vi "Text control 2 v6.6_pump-specific.vi"() -> ()   [LabVIEW 2016]
panel:
  in  "Tab Control":enum32{"Main", "Other parameters"}(tab)
  out "Line running":i32
  out "Total lines":i32
  out "Path":path=path "C:/users/rlp38/09Apr2009LTtesting/test2.txt"
  out "I vs Vg":cluster{"Y data in":dbl[], "X data in":dbl[]}[](graph)
  out "Is max":dbl format="%.2e"
  out "Id max":dbl format="%.2e"
  out "Ig max":dbl format="%.2e"
  out "Imax vs time":cluster{"Y data in":dbl[], "X data in":dbl[]}[](graph)
  out "Imin vs time":cluster{"Y data in":dbl[], "X data in":dbl[]}[](graph)
  out "I vs Vd":cluster{"Y data in":dbl[], "X data in":dbl[]}[](graph)
  in  "Script":string="#-------------------------------------------------------\n# SPM pump cleaning script\n#\n# Version: 0.5\n# Author: Dimitrios Simatos\n# Last updated: 2018-01-05\n#-------------------------------------------------------\n# Description\n#\n# This script is designed to run the cleaning sequence of the SPM OEM pump.\n# This script needs to be run 4 times!\n#-------------------------------------------------------\n# Changes\n#\n# Placed initialization and hard stop commands in the beginning.\n#-------------------------------------------------------\n# Important points\n#\n# Never leave any liquid in the pump to dry after the experiments. If they dry, the residue may block the valve.\n# Always run the cleaning cycle after the experiments.\n# Use clockwise rotation when going up in valve port numbers and vice versa.\n#-------------------------------------------------------\n# Things to do before running the script\n#\n# Set time units to minutes.\n# Set filenames.\n# Replace the tubing, if necessary.\n#-------------------------------------------------------\n# Port connections\n#\n# Port 1: Waste\n# Port 2: Waste\n# Port 3: Various cleaning liquids\n# Port 4: Waste\n# Port 5: Waste\n# Port 6: Waste\n#\n# Between each of the 4 runs, the settings of Port 3 will change, according to the cleaning protocol.\n# The settings for Port 3 are:\n# 1st run: 1% v/v solution of sodium hypochlorite in ultrapure water\n# 2nd run: 0.1% w/v solution of sodium dodecyl sulfate in ultrapure water\n# 3rd run: Ultrapure water\n# 4th run: Waste (in air, not immersed in liquid)\n#-------------------------------------------------------\n# Cleaning protocol for the SPM OEM pump (from the manual)\n#\n# A cleaning procedure should be performed at the end of each day or in between two different experiments.\n# An effective cleaning can be performed in the following manner:\n# • Bleach solution to kill microorganisms\n# 1. Prepare a solution of 1% chlorine bleach and deionized water\n#    NOTE: Prepare a 1% v/v solution of sodium hypochlorite in deionized water\n# 2. Prepare a reservoir and place 1 tubing in the bleach solution and 5 tubings in a waste recipient\n# 3. Pick up the bleach solution through 1 port to entirely fill the syringe\n# 4. Sequentially output the syringe content through the remaining ports and throw it to the waste\n# 5. Repeat operation at least 2 times\n# • Detergent solution to remove debris\n# 1. Prepare a solution of 0.1% detergent and deionized water\n#    NOTE: Prepare a 0.1% w/v solution of sodium dodecyl sulfate in deionized water\n# 2. Move the tubing from the bleach solution reservoir and place it into a reservoir of detergent solution\n# 3. Pick up the detergent solution through 1 port to entirely fill the syringe\n# 4. Sequentially output the detergent solution through the remaining ports into the waste recipient\n# 5. Repeat operation at least 2 times\n# • Rinsing water to prepare the pump for your next experiment\n# 1. Move the tubing from the detergent solution reservoir and place it into a reservoir of deionized water\n# 2. Pick up the rinsing solution through 1 port to entirely fill the syringe\n# 3. Sequentially output the rinse water through the remaining ports into the waste recipient\n# 4. Repeat operation at least 2 times\n# • Replace the tubing, if necessary\n#-------------------------------------------------------\n# Pumping cycles and execution time\n#\n# Execution time for a single cycle: 6 x (1 min + 10 sec) = 7 minutes\n# Total execution time: 4 x 7 = 28 minutes\n# Since the script has to run 4 times, the cleaning lasts for: 4 x 28 = 112 minutes\n# Air must be the last to be pumped through the valve, to remove all liquids.\n# There are 4 pumping cycles. Each one draws a different liquid through port 3 and pumps it sequentially through ports 1,2,4,5,6.\n# During the sequential pumping, each port receives 200 ml of liquid (20% of the total syringe volume = 600 \"plunger units\")\n# The device must be disconnected from the port during the cleaning procedure.\n# All cycles are similar, except cycle 1 has the initialization command uncommented and the first report valve command commented.\n#-------------------------------------------------------\n# Volume of liquid needed\n#\n# Volume of liquid needed per cycle: 1 ml\n# Total volume of liquid needed per script run: 4 x 1 = 4 ml\n# Since the script has to run 4 times, the first 3 with different liquids, I need:\n# 4 ml of 1% v/v solution of sodium hypochlorite in ultrapure water\n# 4 ml of 0.1% w/v solution of sodium dodecyl sulfate in ultrapure water\n# 4 ml of ultrapure water\n#-------------------------------------------------------\n# Parameters\n#\n# Syringe size: 1 ml\n# Step resolution N = 0.01 mm\n# Drawing flow V = 300 pulses/second (6000 ul/min)\n# Pumping flow V = 300 pulses/second (6000 ul/min)\n#-------------------------------------------------------\n# Pump initialization\npump /1T #hard stop pump\npump /1ZR #initialize pump\n#-------------------------------------------------------\n# Cycle 1\n# Fill the syringe\npump /1Q #query pump\npump /1? #report absolute plunger position\n#pump /1?6 #report valve position\nwait-min 1 #wait 1 minute\npump /1N0R #set step resolution: 0.01 mm\npump /1Q #query pump\npump /1? #report absolute plunger position (the plunger should be at 0)\npump /1?6 #report valve position\nwait 1000 #wait 1 second\npump /1V300R #choose speed: 300 steps/s (6000 ul/min)\npump /1Q #query pump\nwait 1000 #wait 1 second\npump /1I3R #go to port 3, clockwise rotation\npump /1Q #query pump\npump /1?6 #report valve position\nwait 1000 #wait 1 second\npump /1A3000R #go to absolute position 3000 (= draw 1 ml)\nwait 30000 #wait 30 seconds\npump /1Q #query pump\npump /1? #report absolute plunger position (the plunger should have finished moving)\n#pump /1?6 #report valve position\n# The sequential pumping begins\n# Port 1\npump /1O1R #switch to port 1, counterclockwise rotation\npump /1Q #query pump\npump /1?6 #report valve position\npump /1A2400R #go to absolute position 2400 (= pump 200 ul)\npump /1Q #query pump\npump /1? #report absolute plunger position (the plunger should be moving to 0)\nwait-min 1 #wait 1 minute\npump /1? #report absolute plunger position (the plunger should have finished moving)\n# Port 2\npump /1I2R #switch to port 2, clockwise rotation\npump /1Q #query pump\npump /1?6 #report valve position\npump /1A1800R #go to absolute position 1800 (= pump 200 ul)\npump /1Q #query pump\npump /1? #report absolute plunger position (the plunger should be moving to 0)\nwait-min 1 #wait 1 minute\npump /1? #report absolute plunger position (the plunger should have finished moving)\n# Port 4\npump /1I4R #switch to port 4, clockwise rotation\npump /1Q #query pump\npump /1?6 #report valve position\npump /1A1200R #go to absolute position 1200 (= pump 200 ul)\npump /1Q #query pump\npump /1? #report absolute plunger position (the plunger should be moving to 0)\nwait-min 1 #wait 1 minute\npump /1? #report absolute plunger position (the plunger should have finished moving)\n# Port 5\npump /1I5R #switch to port 5, clockwise rotation\npump /1Q #query pump\npump /1?6 #report valve position\npump /1A600R #go to absolute position 600 (= pump 200 ul)\npump /1Q #query pump\npump /1? #report absolute plunger position (the plunger should be moving to 0)\nwait-min 1 #wait 1 minute\npump /1? #report absolute plunger position (the plunger should have finished moving)\n# Port 6\npump /1I6R #switch to port 6, clockwise rotation\npump /1Q #query pump\npump /1?6 #report valve position\npump /1A0R #go to absolute position 0 (= pump 200 ul)\npump /1Q #query pump\npump /1? #report absolute plunger position (the plunger should be moving to 0)\nwait-min 1 #wait 1 minute\npump /1? #report absolute plunger position (the plunger should have finished moving)\n#-------------------------------------------------------\n# Cycle 2\n# Fill the syringe\n#pump /1ZR #initialize pump\npump /1Q #query pump\npump /1? #report absolute plunger position\npump /1?6 #report valve position\nwait-min 1 #wait 1 minute\npump /1N0R #set step resolution: 0.01 mm\npump /1Q #query pump\npump /1? #report absolute plunger position (the plunger should be at 0)\npump /1?6 #report valve position\nwait 1000 #wait 1 second\npump /1V300R #choose speed: 300 steps/s (6000 ul/min)\npump /1Q #query pump\nwait 1000 #wait 1 second\npump /1O3R #go to port 3, counterclockwise rotation\npump /1Q #query pump\npump /1?6 #report valve position\nwait 1000 #wait 1 second\npump /1A3000R #go to absolute position 3000 (= draw 1 ml)\nwait 30000 #wait 30 seconds\npump /1Q #query pump\npump /1? #report absolute plunger position (the plunger should have finished moving)\n#pump /1?6 #report valve position\n# The sequential pumping begins\n# Port 1\npump /1O1R #switch to port 1, counterclockwise rotation\npump /1Q #query pump\npump /1?6 #report valve position\npump /1A2400R #go to absolute position 2400 (= pump 200 ul)\npump /1Q #query pump\npump /1? #report absolute plunger position (the plunger should be moving to 0)\nwait-min 1 #wait 1 minute\npump /1? #report absolute plunger position (the plunger should have finished moving)\n# Port 2\npump /1I2R #switch to port 2, clockwise rotation\npump /1Q #query pump\npump /1?6 #report valve position\npump /1A1800R #go to absolute position 1800 (= pump 200 ul)\npump /1Q #query pump\npump /1? #report absolute plunger position (the plunger should be moving to 0)\nwait-min 1 #wait 1 minute\npump /1? #report absolute plunger position (the plunger should have finished moving)\n# Port 4\npump /1I4R #switch to port 4, clockwise rotation\npump /1Q #query pump\npump /1?6 #report valve position\npump /1A1200R #go to absolute position 1200 (= pump 200 ul)\npump /1Q #query pump\npump /1? #report absolute plunger position (the plunger should be moving to 0)\nwait-min 1 #wait 1 minute\npump /1? #report absolute plunger position (the plunger should have finished moving)\n# Port 5\npump /1I5R #switch to port 5, clockwise rotation\npump /1Q #query pump\npump /1?6 #report valve position\npump /1A600R #go to absolute position 600 (= pump 200 ul)\npump /1Q #query pump\npump /1? #report absolute plunger position (the plunger should be moving to 0)\nwait-min 1 #wait 1 minute\npump /1? #report absolute plunger position (the plunger should have finished moving)\n# Port 6\npump /1I6R #switch to port 6, clockwise rotation\npump /1Q #query pump\npump /1?6 #report valve position\npump /1A0R #go to absolute position 0 (= pump 200 ul)\npump /1Q #query pump\npump /1? #report absolute plunger position (the plunger should be moving to 0)\nwait-min 1 #wait 1 minute\npump /1? #report absolute plunger position (the plunger should have finished moving)\n#-------------------------------------------------------\n# Cycle 3\n# Fill the syringe\n#pump /1ZR #initialize pump\npump /1Q #query pump\npump /1? #report absolute plunger position\npump /1?6 #report valve position\nwait-min 1 #wait 1 minute\npump /1N0R #set step resolution: 0.01 mm\npump /1Q #query pump\npump /1? #report absolute plunger position (the plunger should be at 0)\npump /1?6 #report valve position\nwait 1000 #wait 1 second\npump /1V300R #choose speed: 300 steps/s (6000 ul/min)\npump /1Q #query pump\nwait 1000 #wait 1 second\npump /1O3R #go to port 3, counterclockwise rotation\npump /1Q #query pump\npump /1?6 #report valve position\nwait 1000 #wait 1 second\npump /1A3000R #go to absolute position 3000 (= draw 1 ml)\nwait 30000 #wait 30 seconds\npump /1Q #query pump\npump /1? #report absolute plunger position (the plunger should have finished moving)\n#pump /1?6 #report valve position\n# The sequential pumping begins\n# Port 1\npump /1O1R #switch to port 1, counterclockwise rotation\npump /1Q #query pump\npump /1?6 #report valve position\npump /1A2400R #go to absolute position 2400 (= pump 200 ul)\npump /1Q #query pump\npump /1? #report absolute plunger position (the plunger should be moving to 0)\nwait-min 1 #wait 1 minute\npump /1? #report absolute plunger position (the plunger should have finished moving)\n# Port 2\npump /1I2R #switch to port 2, clockwise rotation\npump /1Q #query pump\npump /1?6 #report valve position\npump /1A1800R #go to absolute position 1800 (= pump 200 ul)\npump /1Q #query pump\npump /1? #report absolute plunger position (the plunger should be moving to 0)\nwait-min 1 #wait 1 minute\npump /1? #report absolute plunger position (the plunger should have finished moving)\n# Port 4\npump /1I4R #switch to port 4, clockwise rotation\npump /1Q #query pump\npump /1?6 #report valve position\npump /1A1200R #go to absolute position 1200 (= pump 200 ul)\npump /1Q #query pump\npump /1? #report absolute plunger position (the plunger should be moving to 0)\nwait-min 1 #wait 1 minute\npump /1? #report absolute plunger position (the plunger should have finished moving)\n# Port 5\npump /1I5R #switch to port 5, clockwise rotation\npump /1Q #query pump\npump /1?6 #report valve position\npump /1A600R #go to absolute position 600 (= pump 200 ul)\npump /1Q #query pump\npump /1? #report absolute plunger position (the plunger should be moving to 0)\nwait-min 1 #wait 1 minute\npump /1? #report absolute plunger position (the plunger should have finished moving)\n# Port 6\npump /1I6R #switch to port 6, clockwise rotation\npump /1Q #query pump\npump /1?6 #report valve position\npump /1A0R #go to absolute position 0 (= pump 200 ul)\npump /1Q #query pump\npump /1? #report absolute plunger position (the plunger should be moving to 0)\nwait-min 1 #wait 1 minute\npump /1? #report absolute plunger position (the plunger should have finished moving)\n#-------------------------------------------------------\n# Cycle 4\n# Fill the syringe\n#pump /1ZR #initialize pump\npump /1Q #query pump\npump /1? #report absolute plunger position\npump /1?6 #report valve position\nwait-min 1 #wait 1 minute\npump /1N0R #set step resolution: 0.01 mm\npump /1Q #query pump\npump /1? #report absolute plunger position (the plunger should be at 0)\npump /1?6 #report valve position\nwait 1000 #wait 1 second\npump /1V300R #choose speed: 300 steps/s (6000 ul/min)\npump /1Q #query pump\nwait 1000 #wait 1 second\npump /1O3R #go to port 3, counterclockwise rotation\npump /1Q #query pump\npump /1?6 #report valve position\nwait 1000 #wait 1 second\npump /1A3000R #go to absolute position 3000 (= draw 1 ml)\nwait 30000 #wait 30 seconds\npump /1Q #query pump\npump /1? #report absolute plunger position (the plunger should have finished moving)\n#pump /1?6 #report valve position\n# The sequential pumping begins\n# Port 1\npump /1O1R #switch to port 1, counterclockwise rotation\npump /1Q #query pump\npump /1?6 #report valve position\npump /1A2400R #go to absolute position 2400 (= pump 200 ul)\npump /1Q #query pump\npump /1? #report absolute plunger position (the plunger should be moving to 0)\nwait-min 1 #wait 1 minute\npump /1? #report absolute plunger position (the plunger should have finished moving)\n# Port 2\npump /1I2R #switch to port 2, clockwise rotation\npump /1Q #query pump\npump /1?6 #report valve position\npump /1A1800R #go to absolute position 1800 (= pump 200 ul)\npump /1Q #query pump\npump /1? #report absolute plunger position (the plunger should be moving to 0)\nwait-min 1 #wait 1 minute\npump /1? #report absolute plunger position (the plunger should have finished moving)\n# Port 4\npump /1I4R #switch to port 4, clockwise rotation\npump /1Q #query pump\npump /1?6 #report valve position\npump /1A1200R #go to absolute position 1200 (= pump 200 ul)\npump /1Q #query pump\npump /1? #report absolute plunger position (the plunger should be moving to 0)\nwait-min 1 #wait 1 minute\npump /1? #report absolute plunger position (the plunger should have finished moving)\n# Port 5\npump /1I5R #switch to port 5, clockwise rotation\npump /1Q #query pump\npump /1?6 #report valve position\npump /1A600R #go to absolute position 600 (= pump 200 ul)\npump /1Q #query pump\npump /1? #report absolute plunger position (the plunger should be moving to 0)\nwait-min 1 #wait 1 minute\npump /1? #report absolute plunger position (the plunger should have finished moving)\n# Port 6\npump /1I6R #switch to port 6, clockwise rotation\npump /1Q #query pump\npump /1?6 #report valve position\npump /1A0R #go to absolute position 0 (= pump 200 ul)\npump /1Q #query pump\npump /1? #report absolute plunger position (the plunger should be moving to 0)\nwait-min 1 #wait 1 minute\npump /1? #report absolute plunger position (the plunger should have finished moving)\n#-------------------------------------------------------"
  out "Command running:":string
  out "Serial port data":string
  out "Elapsed Time":dbl caption="Elapsed Time (s)"
  in  "Time Units":u16(ring)=1 items=["Seconds", "Minutes", "Hours"]
  in  "Time Offset":dbl caption="Set Start Time (s)"
  in  "Reset":bool
  in  "Auto Reset":bool
  in  "integration time":u32(slide) max=2 step=1 scale=0.0..2.0
  in  "Interrupt scan":bool
  out "Absolute plunger position vs time":cluster{"Y data in":dbl[], "X data in":dbl[]}[](graph)
  out "Valve position vs time":cluster{"Y data in":dbl[], "X data in":dbl[]}[](graph)
  out "Is on":dbl format="%.2e"
  out "Id on":dbl format="%.2e"
  out "Ig on":dbl format="%.2e"
  out "Ion vs time":cluster{"Y data in":dbl[], "X data in":dbl[]}[](graph)
  out "Ioff vs time":cluster{"Y data in":dbl[], "X data in":dbl[]}[](graph)
  out "Ig min":dbl format="%.2e"
  out "Id min":dbl format="%.2e"
  out "Is min":dbl format="%.2e"
  out "Is off":dbl format="%.2e"
  out "Id off":dbl format="%.2e"
  out "Ig off":dbl format="%.2e"
  in  "Integration time (long)":dbl=0.32 min=0.04 max=2.0 step=0.02 format="%.2f"
  in  "Integration time (short)":dbl=0.0019 min=8e-05 max=0.0019 step=8e-05 format="%^.0e"
  in  "Gate: Compliance":dbl=0.001 format="%.8f"
  in  "Drain: Compliance":dbl=0.001 format="%.8f"
  in  "Hard stop pump":bool
  in  "Halt pump":bool
  in  "Interrupt program":bool
  in  "Suffix (script)":string="step_1_up-H2O_initial_script.txt"
  in  "Filename (variable part)":string="step_1_up-H2O_initial_"
  in  "Plot output curve extrema vs time":bool
  in  "Plot transfer curve extrema vs time":bool=TRUE
  in  "Plot sample extrema vs time":bool
  out "I vs time (Bias Stress)":cluster{"Y data in":dbl[], "X data in":dbl[]}[](graph)
  in  "Gate Range\nmode":u16(ring) items=["Auto", "Limited", "Fixed"]
  in  "Gate Range":u8(slide)=6 max=11 scale=0.0..11.0
  in  "Source/Drain\nRange mode":u16(ring) items=["Auto", "Limited", "Fixed"]
  in  "Source/Drain Range":u8(slide)=6 max=11 scale=0.0..11.0
  in  "Panel Controls":T1={"Emergency Stop"=refnum, "TransGraph Max"=1e-05, "Text/Graph (text=false)"=TRUE} {"TransGraph Max" format="%.2e"}
  in  "Panel Controls 2":T2={"Emergency Stop"=refnum, "TransGraph Max"=1e-05, "Text/Graph (text=false)"=TRUE, "TransGraph Min"=1e-11} {"TransGraph Min" format="%.2e"; "TransGraph Max" format="%.2e"}
  in  "SMU4":cluster{"on/off":bool, "Voltage":dbl} {"Voltage" min=-100.0 max=100.0 format="%.2f"}
  in  "Full Reset":bool
  in  "Standby":T3
  out "error out":errorcluster
  in  "Delay before read (ms)":u32=1000
  in  "byte count":u32=64
  in  "Serial End Mode for Reads":u16(ring)=2 items=["None", "LastBit", "TermChar"]
  in  "Timeout (ms)":u32=10000
  in  "Enable Termination\nChar (T)":bool=TRUE
  in  "Termination char\n(0xA = '\\n' = LF)\n(0xD = '\\r' = CR)":u8=13 format="%.0x"
  in  "flow control":u16(ring) items=["None"=0, "XON/XOFF"=1, "RTS/CTS"=2, "DTR/DSR"=4]
  in  "stop bits":u16(ring)=10 items=["1.0"=10, "1.5"=15, "2.0"=20]
  in  "parity":u16(ring) items=["None", "Odd", "Even", "Mark", "Space"]
  in  "data bits":u16=8 min=5 max=8 step=1
  in  "VISA resource name":refnum<visa-resource-name>="COM6"
  in  "baud rate":u32=9600
  out "Timings Indicator":T4
  in  "Timings (overwritten by the Front Panel)":T5={"integration time"=0, "Short/Long integration time"=0.00064, "hold time (sec)"=0.0, "delay time (sec)"=0.0, "Step Time (0 disables)"=0.0, "sweep method"=0, "Pulse period"=0.005, "Base voltage"=0.0, "Pulse width"=0.0005} {"Pulse width" min=0.0005 max=0.1 step=0.0001 format="%.4f"; "Base voltage" format="%^.4e"; "Pulse period" min=0.005 max=1.0 step=0.0001 format="%.4f"; "sweep method" items=["Continuous", "Pulsed"]; "Step Time (0 disables)" format="%.2f"; "delay time (sec)" format="%.4f"; "hold time (sec)" format="%.4f"; "Short/Long integration time" format="%^.0e"; "integration time" scale=0.0..2.0}
  out "SMU4 Indicator":cluster{"on/off":bool, "Voltage":dbl} {"Voltage" min=-100.0 max=100.0 format="%.2f"}
  in  "Gate":T6={"Gate Start"=0.0, "Gate Stop"=2.0, "Gate Step (linear only)"=1.0, "Gate Compliance"=0.0001, "Gate PComp"=0.0, "Range mode"=0, "Range"=6} {"Range" max=11 scale=0.0..11.0; "Range mode" items=["Auto", "Limited", "Fixed"]; "Gate PComp" format="%^.2e"; "Gate Compliance" format="%^.2e"; "Gate Step (linear only)" format="%^.4e"; "Gate Stop" format="%^.4e"; "Gate Start" format="%^.4e"}
  in  "Drain 2":T7={"Drain Start"=0.0, "Drain Stop"=2.0, "Drain Compliance"=0.0001, "Drain Step"=1.0, "Drain PComp"=0.0, "Range mode"=0, "Range"=6} {"Range" max=11 scale=0.0..11.0; "Range mode" items=["Auto", "Limited", "Fixed"]; "Drain PComp" format="%^.2e"; "Drain Step" format="%^.4e"; "Drain Compliance" format="%^.2e"; "Drain Stop" format="%^.4e"; "Drain Start" format="%^.4e"}
  # "Syntax:\nitime [s|m|l] time(sec): [s|m|l] determines the integration time setting (small|medium|long) and time sets the value.\nNOTE: The value of the integration time has to be within the range allowed by its category (s|m|l), otherwise, the closest value will be used. (e.g. if the category is set to short but the time value is very long, the actual value used will be the maximum short integration time.\nIntegration times:\n    Short: Default: 640 us. Range: 8E-5 - 1.92E-3 seconds.\n    Medium: Fixed at 1 NPL cycle (0.02 seconds).\n    Long: Default: 16 NPL cycles (0.32 seconds). Range: 2-100 NPL cycles (0.04 seconds - 2 seconds).\ngaterangemode [a|l|f]\ndrainrangemode [a|l|f]\npulsed [on|off] PulsePeriod(sec) PulseBaseVoltage PulseONWidth(sec)\nstandby [on l off]\nwait NumMilliseconds\nwait-min NumMinutes\n# texthere = comment\nSMU4 [ON|OFF] Voltage\ntransfer [s|d] VgStart VgStop VgStep VdStart VdStop VdStep\noutput [s|d] VgStart VgStop VgStep VdStart VdStop VdStep\nsample Vg Vd NumSamples Time(s) SampleInterval(s)\nsamplei Idg NumSamples Time(s) SampleInterval(s) VDGcompliance\n100 samples is approximately 13 seconds with medium integration\n# If in doubt use SampleInterval(s) = 0.004\n    NOTE: When doing bias stress measurements, set the Time Units to \"Seconds\", as the \"sample\" command has been configured to give the output to seconds.\nstressV VG VD IGcompliance IDcompliance Duration(sec)\nstressI IDG VDGcompliance Duration(sec)\nvsu2pulse Bias Duration(s)\npulsedstressV [s|d] VEstop VgON VgOFF Period(s) PulseONwidth(s) Vd\nsample-fpp Vg Vd NumSamples Time\nresample-fpp Vg Vd\ntransfer-fpp [s|d] VgStart VgStop VgStep VdStart VdStop VdStep\noutput-fpp [s|d] VgStart VgStop VgStep VdStart VdStop VdStep\nserial SerialPortCommand\npump SerialPortCommand for the SPM pump\n\nSPM Pump Syntax (<x>: pump number, use 1 if only one pump):\nif the command syntax contains [R], then append the letter R to the command\n/<x>Q: query (a query command should follow each command)\n/<x>Z[R] or /<x>Y[R]: initialize pump\n/<x>N<n>[R] (<n>=0,1): <0> (<1>) microstep 0.01 mm (0.00125 mm) resolution\n/<x>I<n> (<n>=0-6): turn to port number n (clockwise)\n/<x>O<n> (<n>=0-6): turn to port number n (counterclockwise)\n/<x>X: Re-execute last command string\n/<x>G<n>[R] (<n>=0-60000): repeat command sequence (default: 0, 0=loop forever)\n/<x>g: Mark the start of a repeat sequence (max = 10)\n/<x>M<n>[R] (<n>=0-86400000): delay command execution by n milliseconds\n/<x>H: Halt; Pause the sequence after finishing the current move\n/<x>T: Hardstop; Interrupt the current move and suppress it from the sequence\n/<x>A<n>[R] (<n>=0-3000 with N=0, 0-24000 with N=1): absolute position\n/<x>P<n>[R] (<n>=0-3000 with N=0, 0-24000 with N=1): relative pickup\n/<x>D<n>[R] (<n>=0-3000 with N=0, 0-24000 with N=1): relative dispense\n/<x>V<n>[R] (<n>=1-1600 default: 150): set peak speed (pulses/sec)\nNOTE: The lowest speed limit is 1 pulse/sec, not 5, as the manual states.\n/<x>S<n>[R] (<n>=10-40 default: 22): set speed (NOT in pulses/sec, look in manual)\nNOTE: When controlled with absolute position, one does not need to pay special attention to the syringe that is mounted on the pump.\nWithdraw from lower stage (ports 3, 5), dispense from higher stage (ports 2, 4, 6).\nConnect Port 1 to waste."
  # "Time"
  # "1\n2\n3\n4\n5\n6\n7\n8\n9\n10\n11\n12\n13\n14\n15\n16\n17\n18\n19\n20"
  # "Serial port settings"
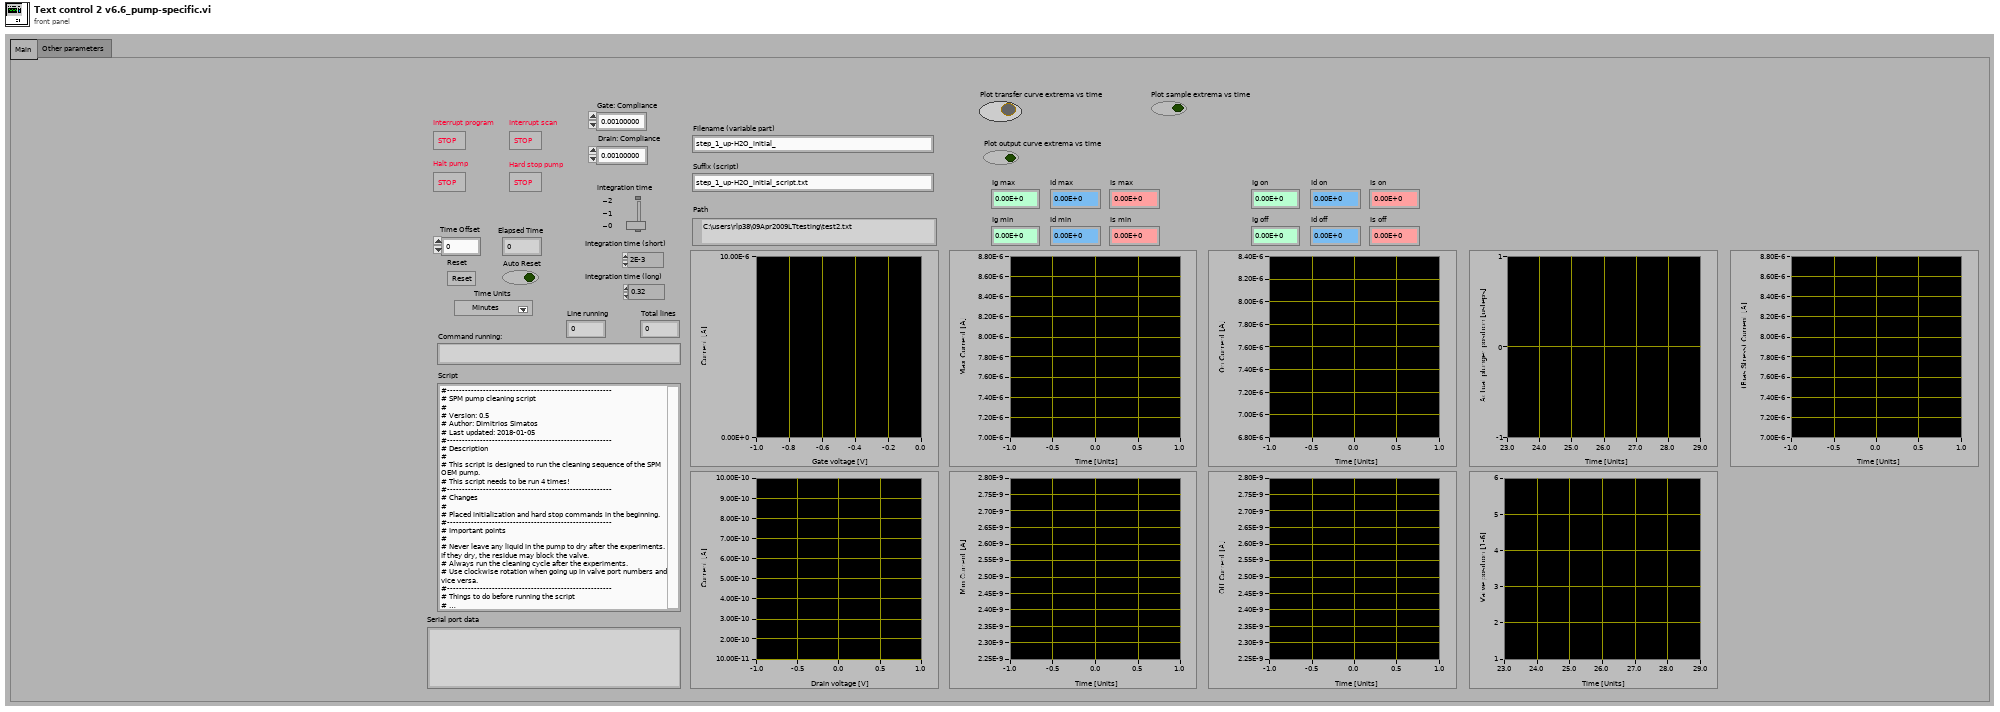
[diagram p1: front panel]
types:
  T1 = cluster{"Emergency Stop":refnum<vi>, "TransGraph Max":dbl, "Text/Graph (text=false)":bool}
  T2 = cluster{"Emergency Stop":refnum<vi>, "TransGraph Max":dbl, "Text/Graph (text=false)":bool, "TransGraph Min":dbl}
  T3 = cluster{"Gate Standby":bool, "Drain Standby":bool}
  T4 = cluster{"integration time (0:s, 1:m, 2:l)":u32, "Short/Long integration time":dbl, "hold time (sec)":dbl, "delay time (sec)":dbl, "Step Time (0 disables)":dbl, "sweep method":u16, "Pulse period":dbl, "Base voltage":dbl, "Pulse width":dbl}
  T5 = cluster{"integration time":u32, "Short/Long integration time":dbl, "hold time (sec)":dbl, "delay time (sec)":dbl, "Step Time (0 disables)":dbl, "sweep method":u16, "Pulse period":dbl, "Base voltage":dbl, "Pulse width":dbl}
  T6 = cluster{"Gate Start":dbl, "Gate Stop":dbl, "Gate Step (linear only)":dbl, "Gate Compliance":dbl, "Gate PComp":dbl, "Range mode":u16, "Range":u8}
  T7 = cluster{"Drain Start":dbl, "Drain Stop":dbl, "Drain Compliance":dbl, "Drain Step":dbl, "Drain PComp":dbl, "Range mode":u16, "Range":u8}
  T8 = enum16{"open", "replace", "create", "open or create", "replace or create", "replace or create with confirmation"}
  T9 = cluster{"V2 Start":dbl, "V2 Step":dbl, "Number of points":i32}
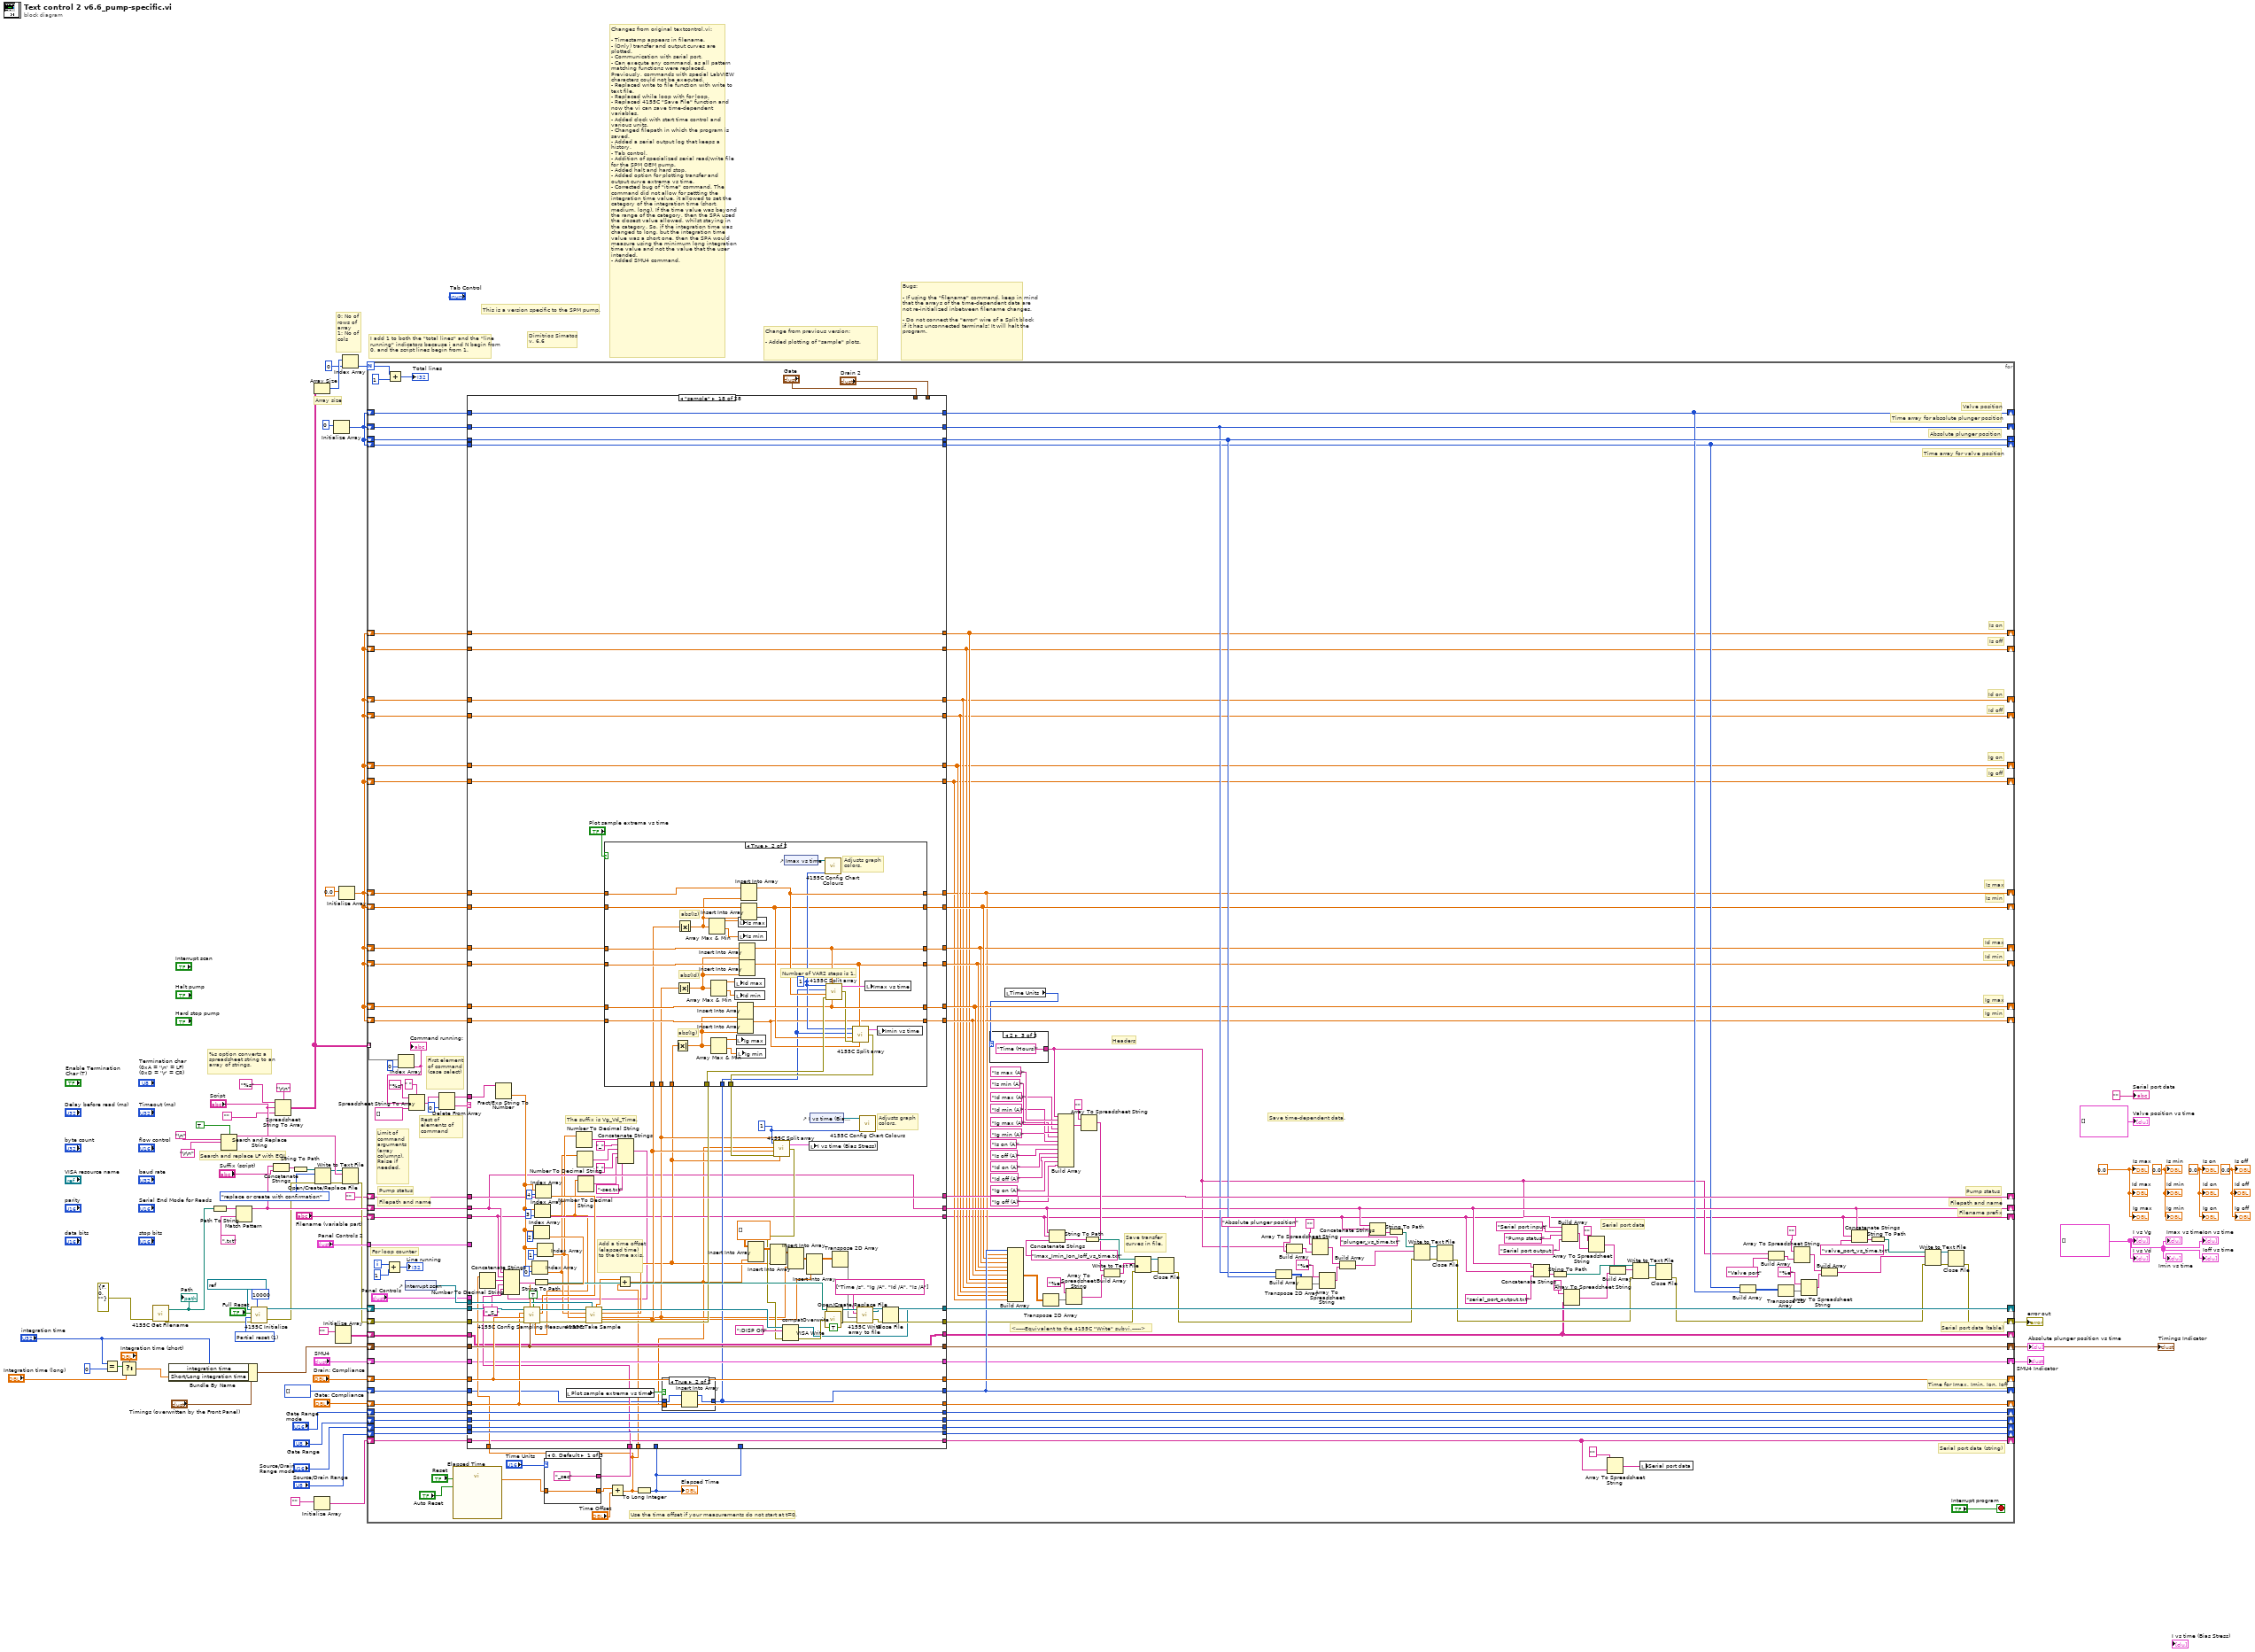
[diagram p0: block diagram]
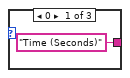
[diagram p2: hidden frame]
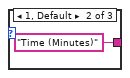
[diagram p3: hidden frame]
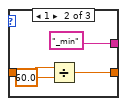
[diagram p4: hidden frame]
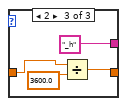
[diagram p5: hidden frame]
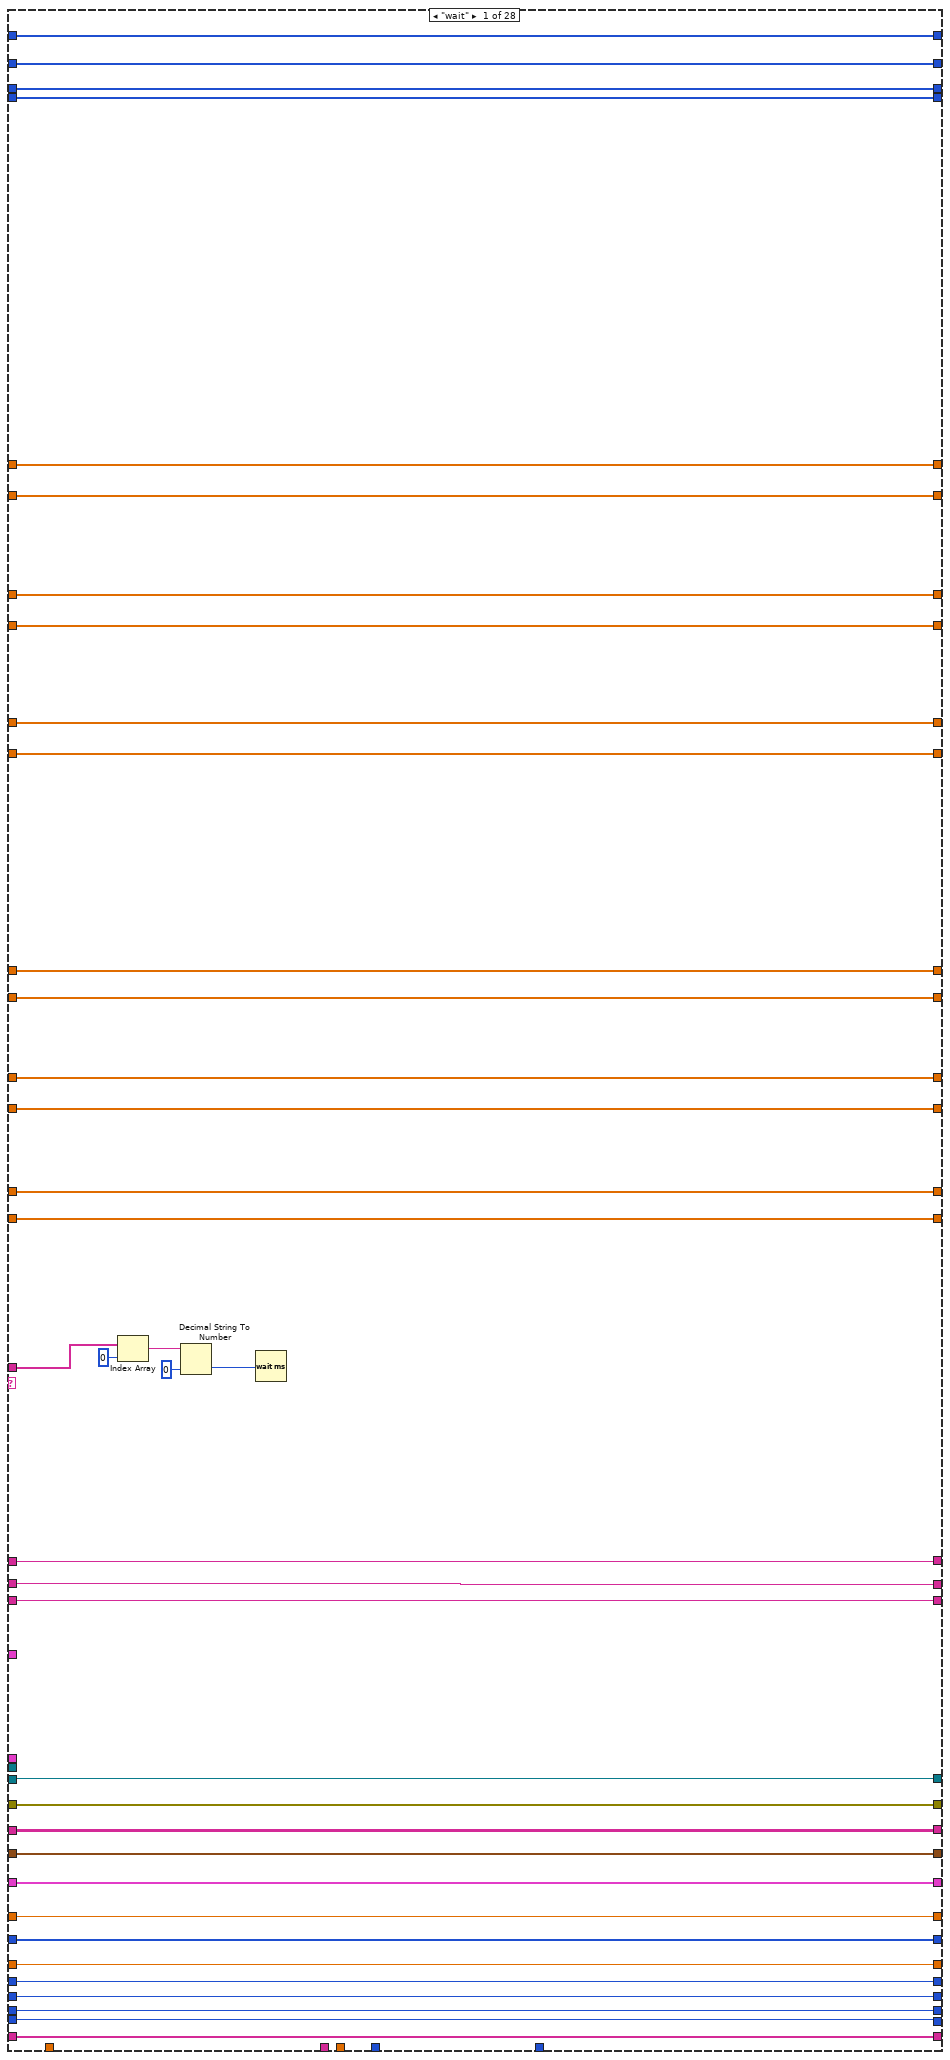
[diagram p6: hidden frame]
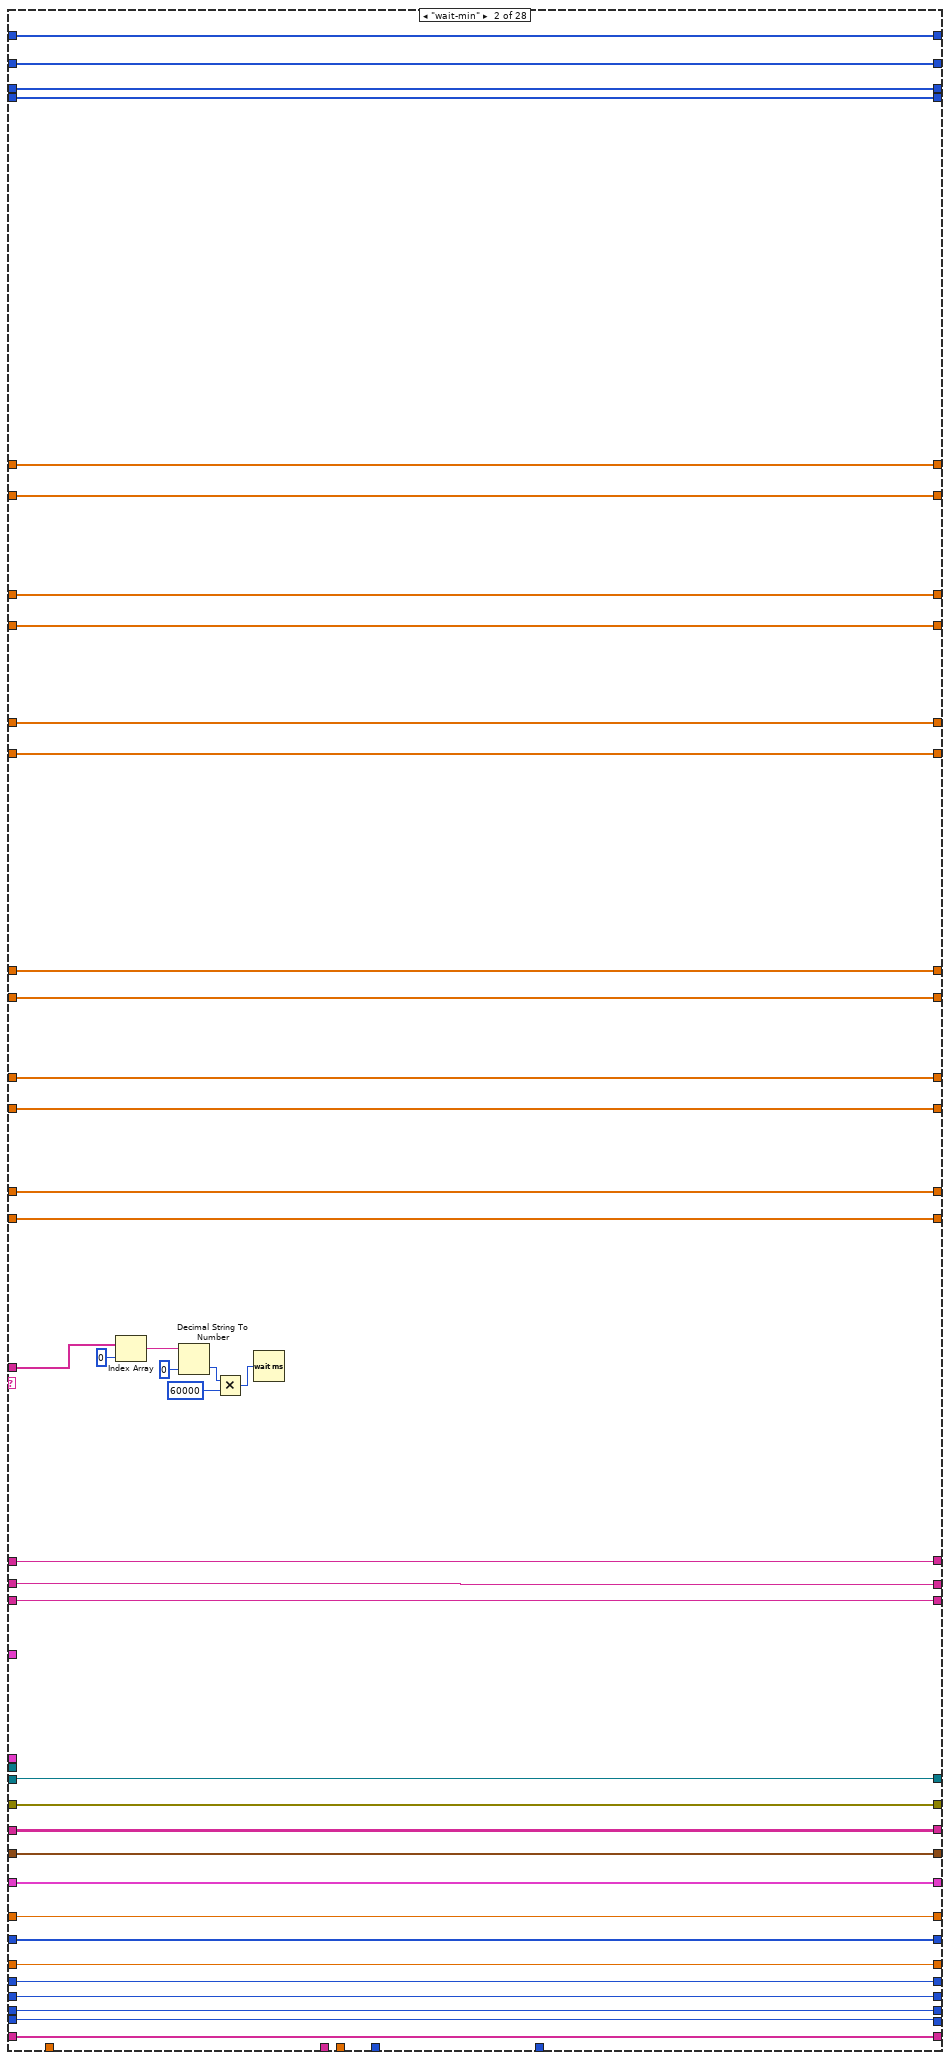
[diagram p7: hidden frame]
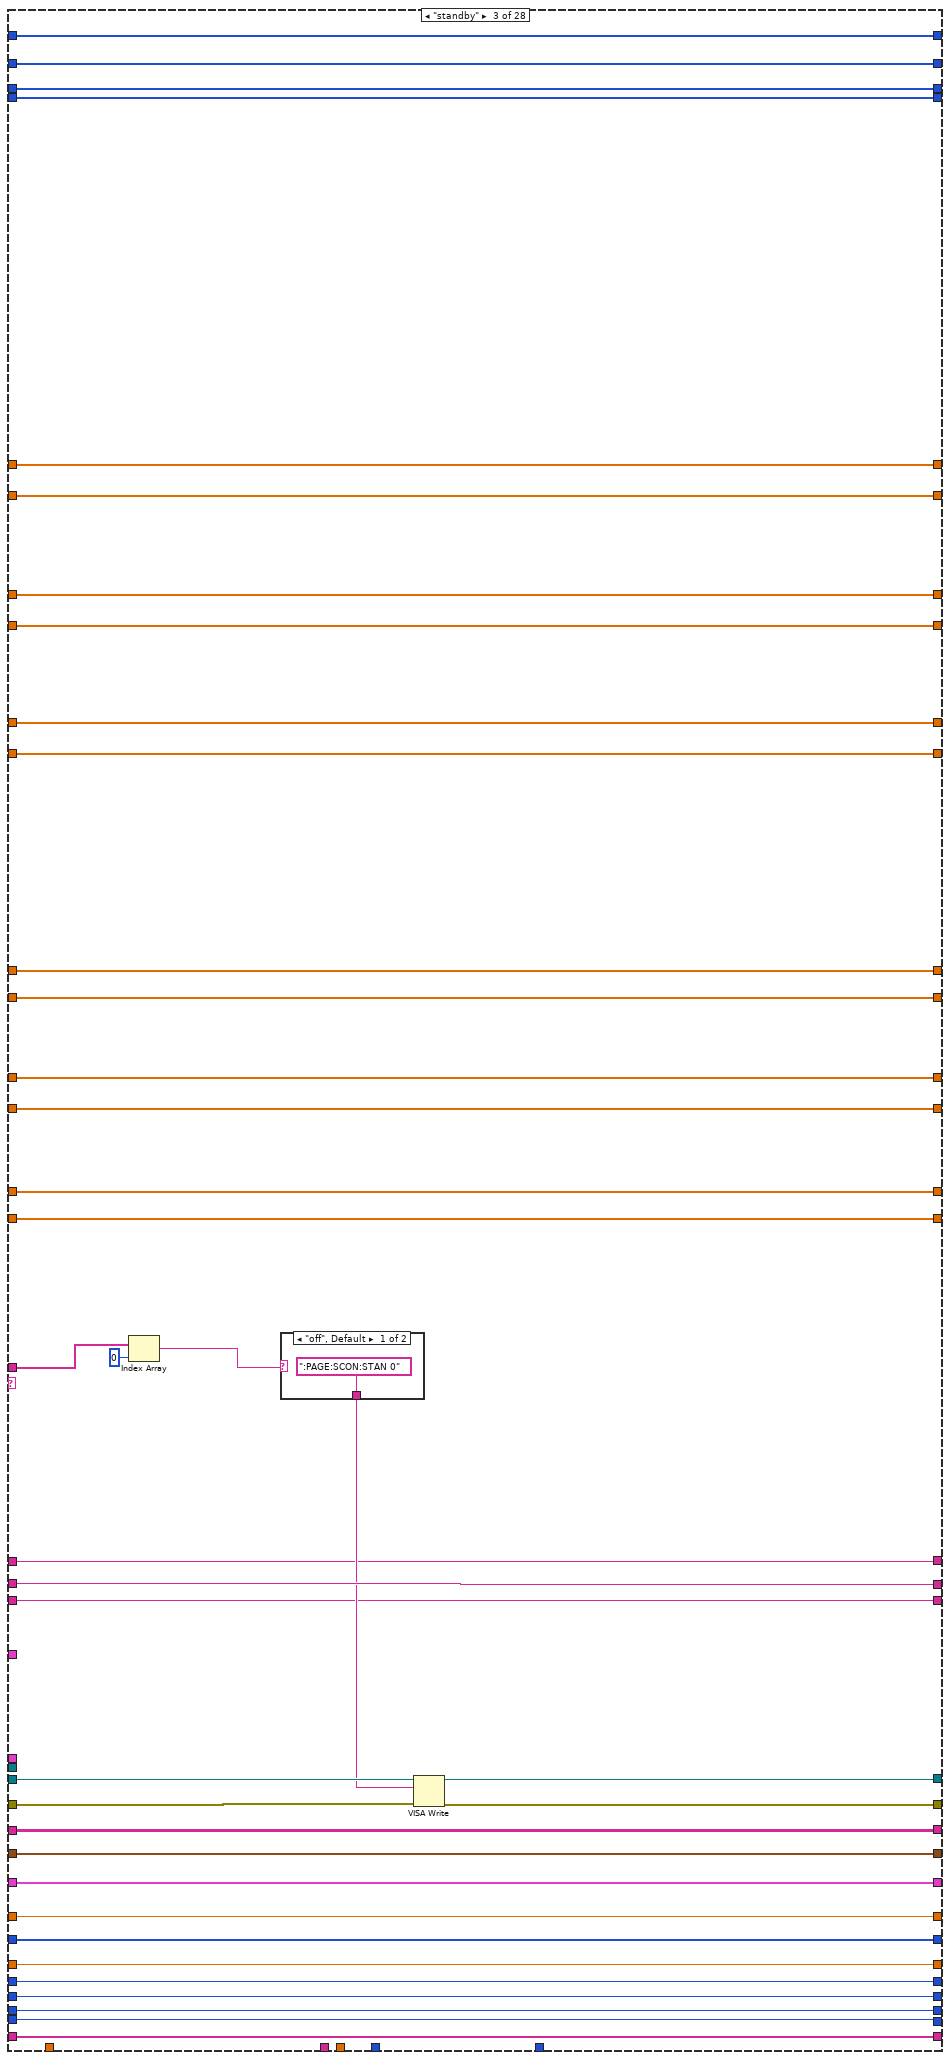
[diagram p8: hidden frame]
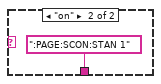
[diagram p9: hidden frame]
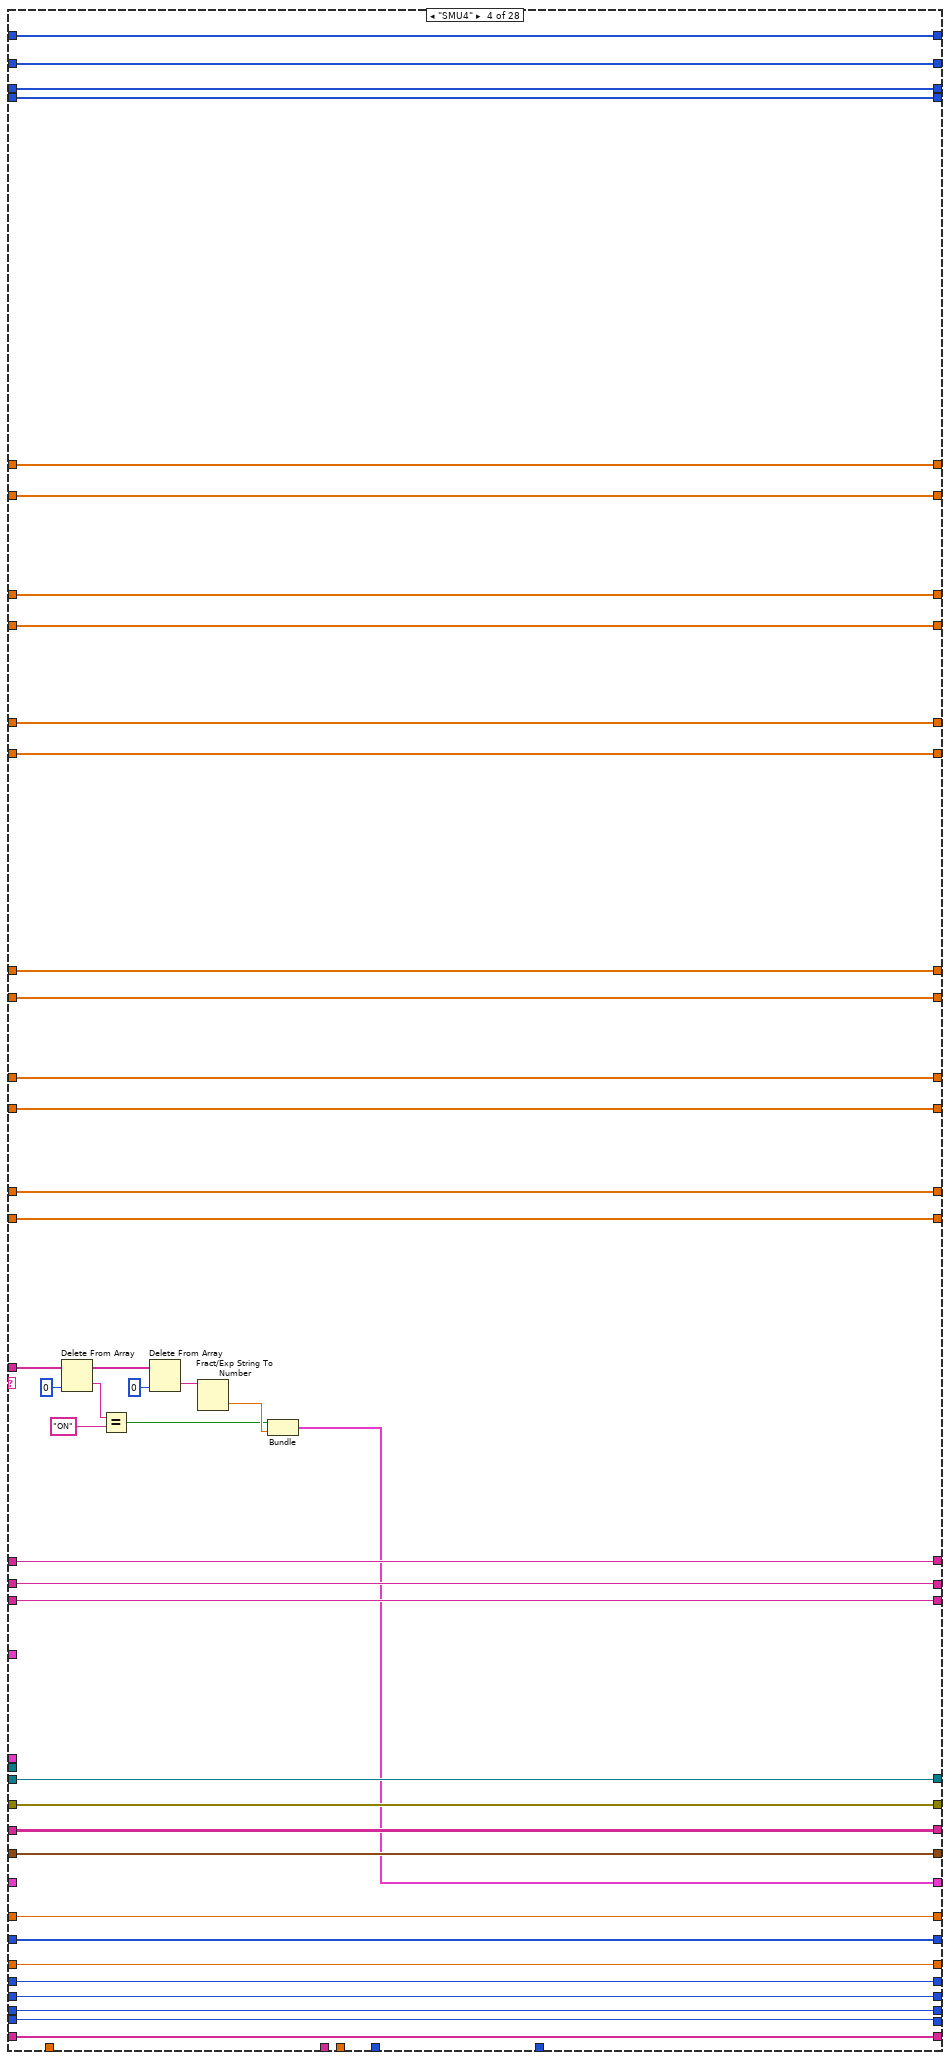
[diagram p10: hidden frame]
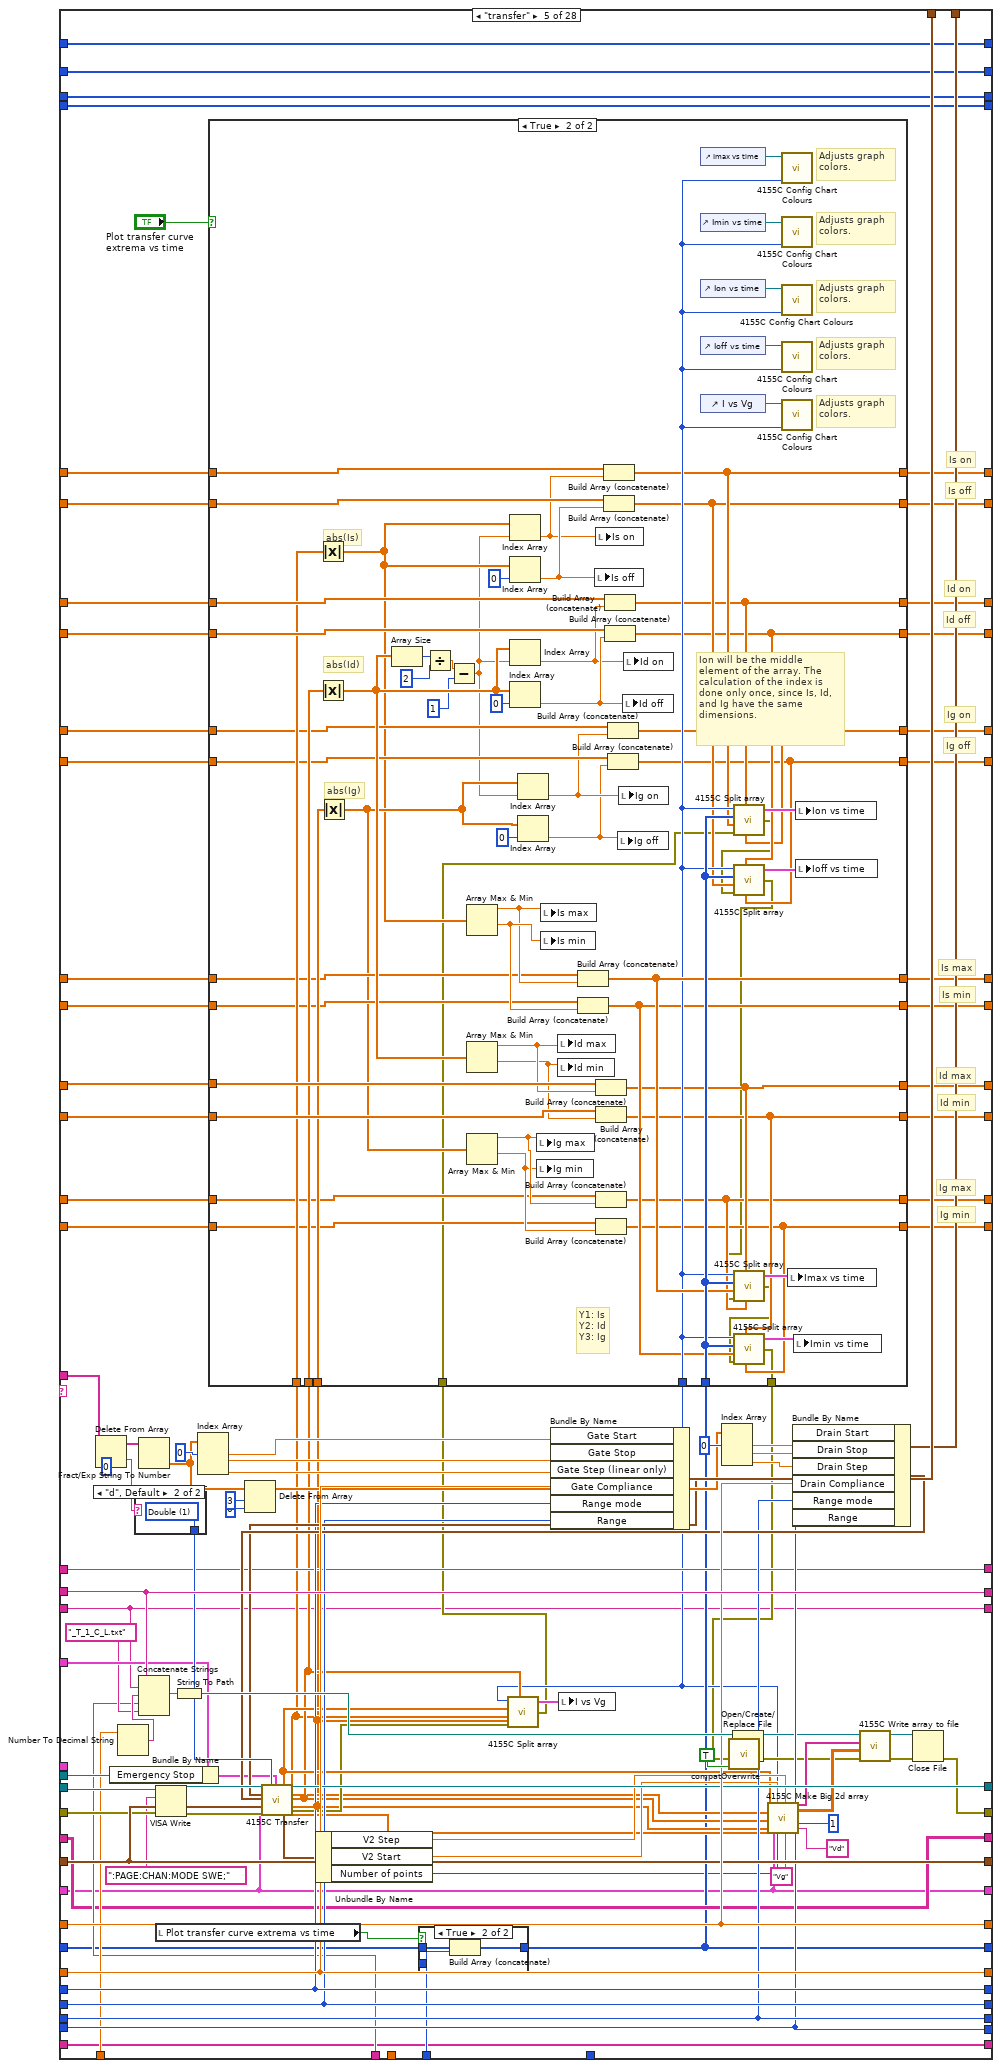
[diagram p11: hidden frame]
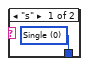
[diagram p14: hidden frame]
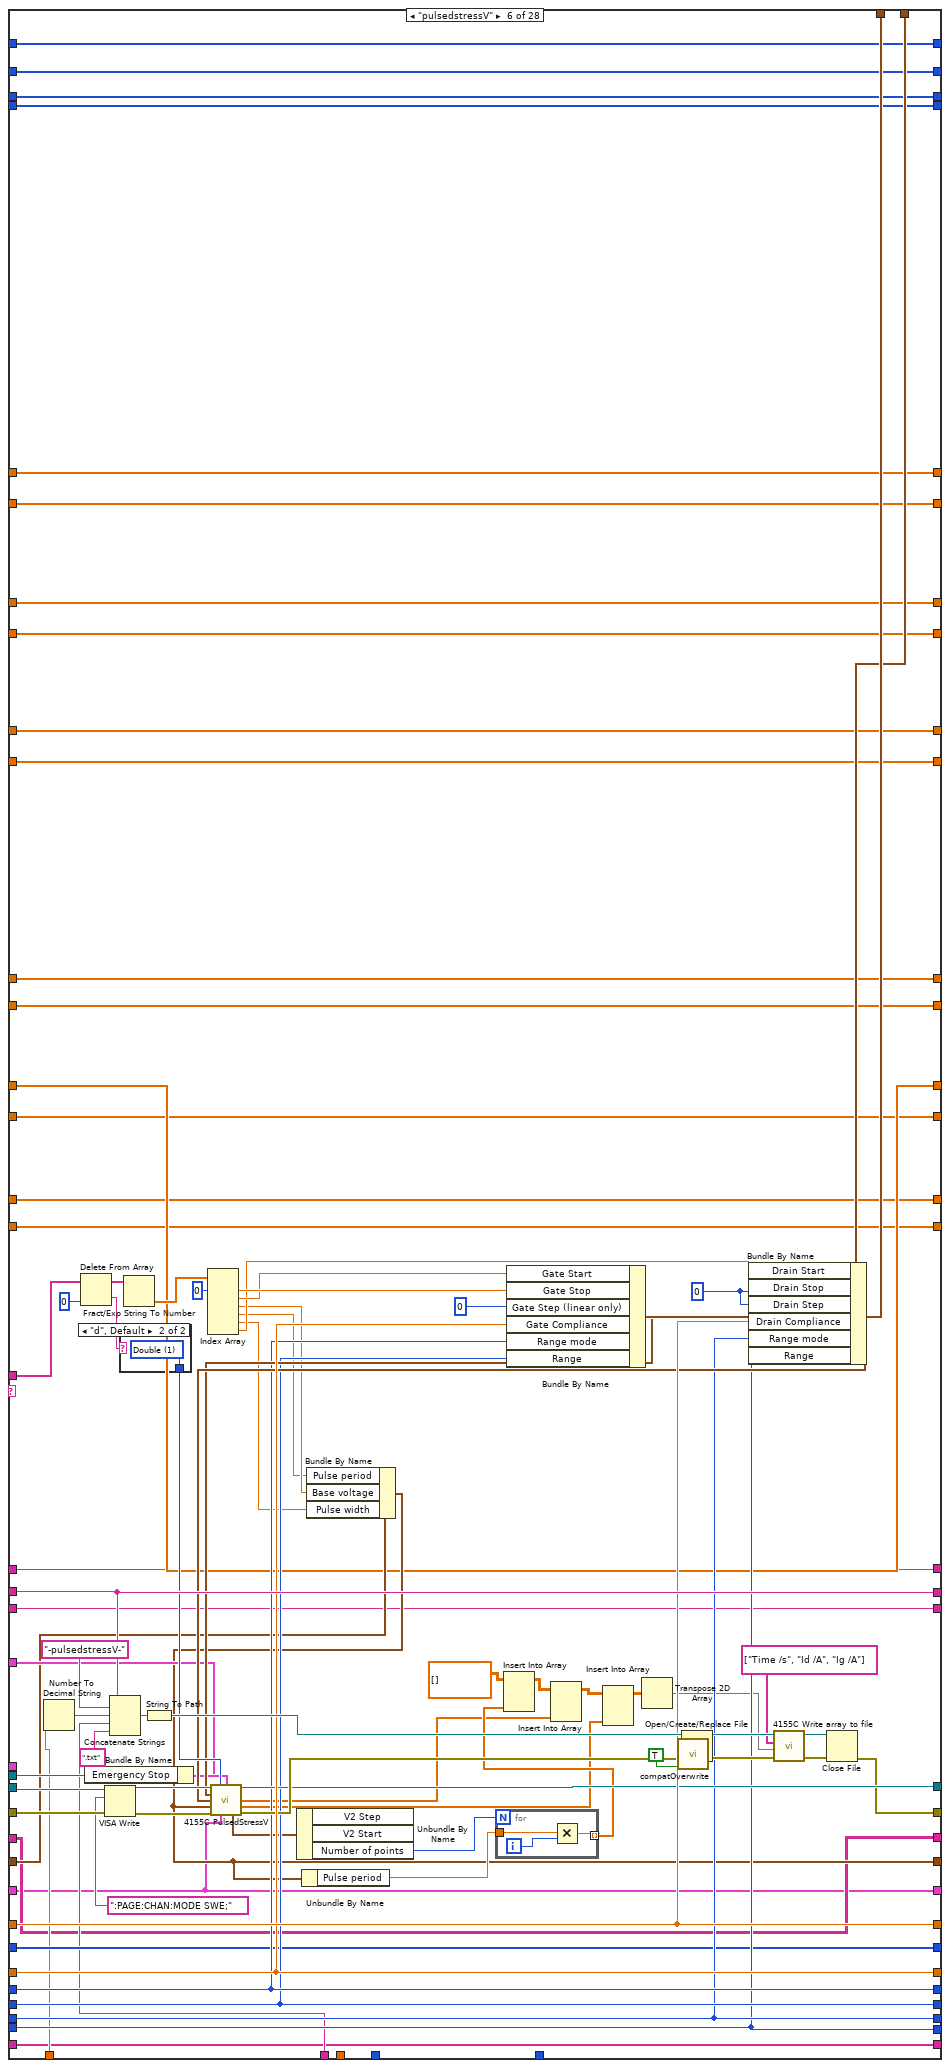
[diagram p15: hidden frame]
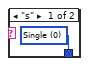
[diagram p16: hidden frame]
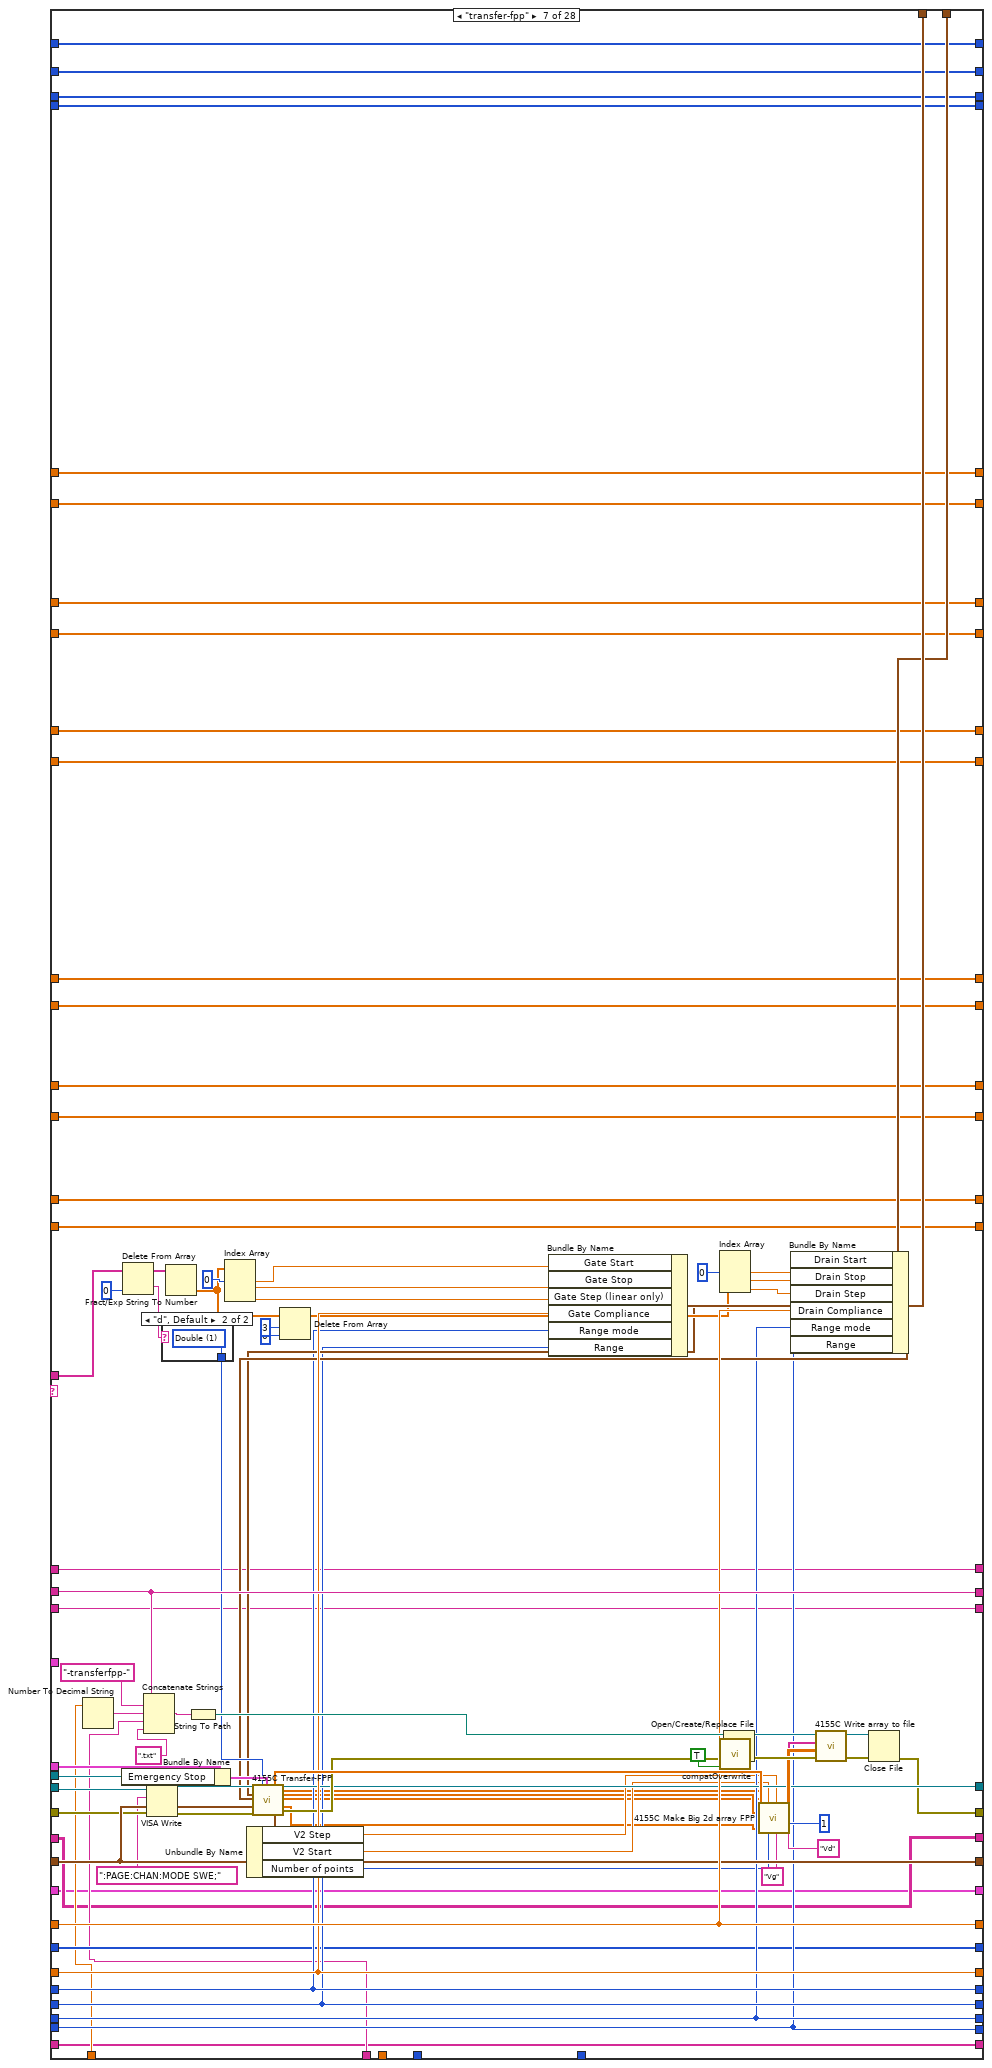
[diagram p17: hidden frame]
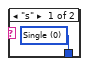
[diagram p18: hidden frame]
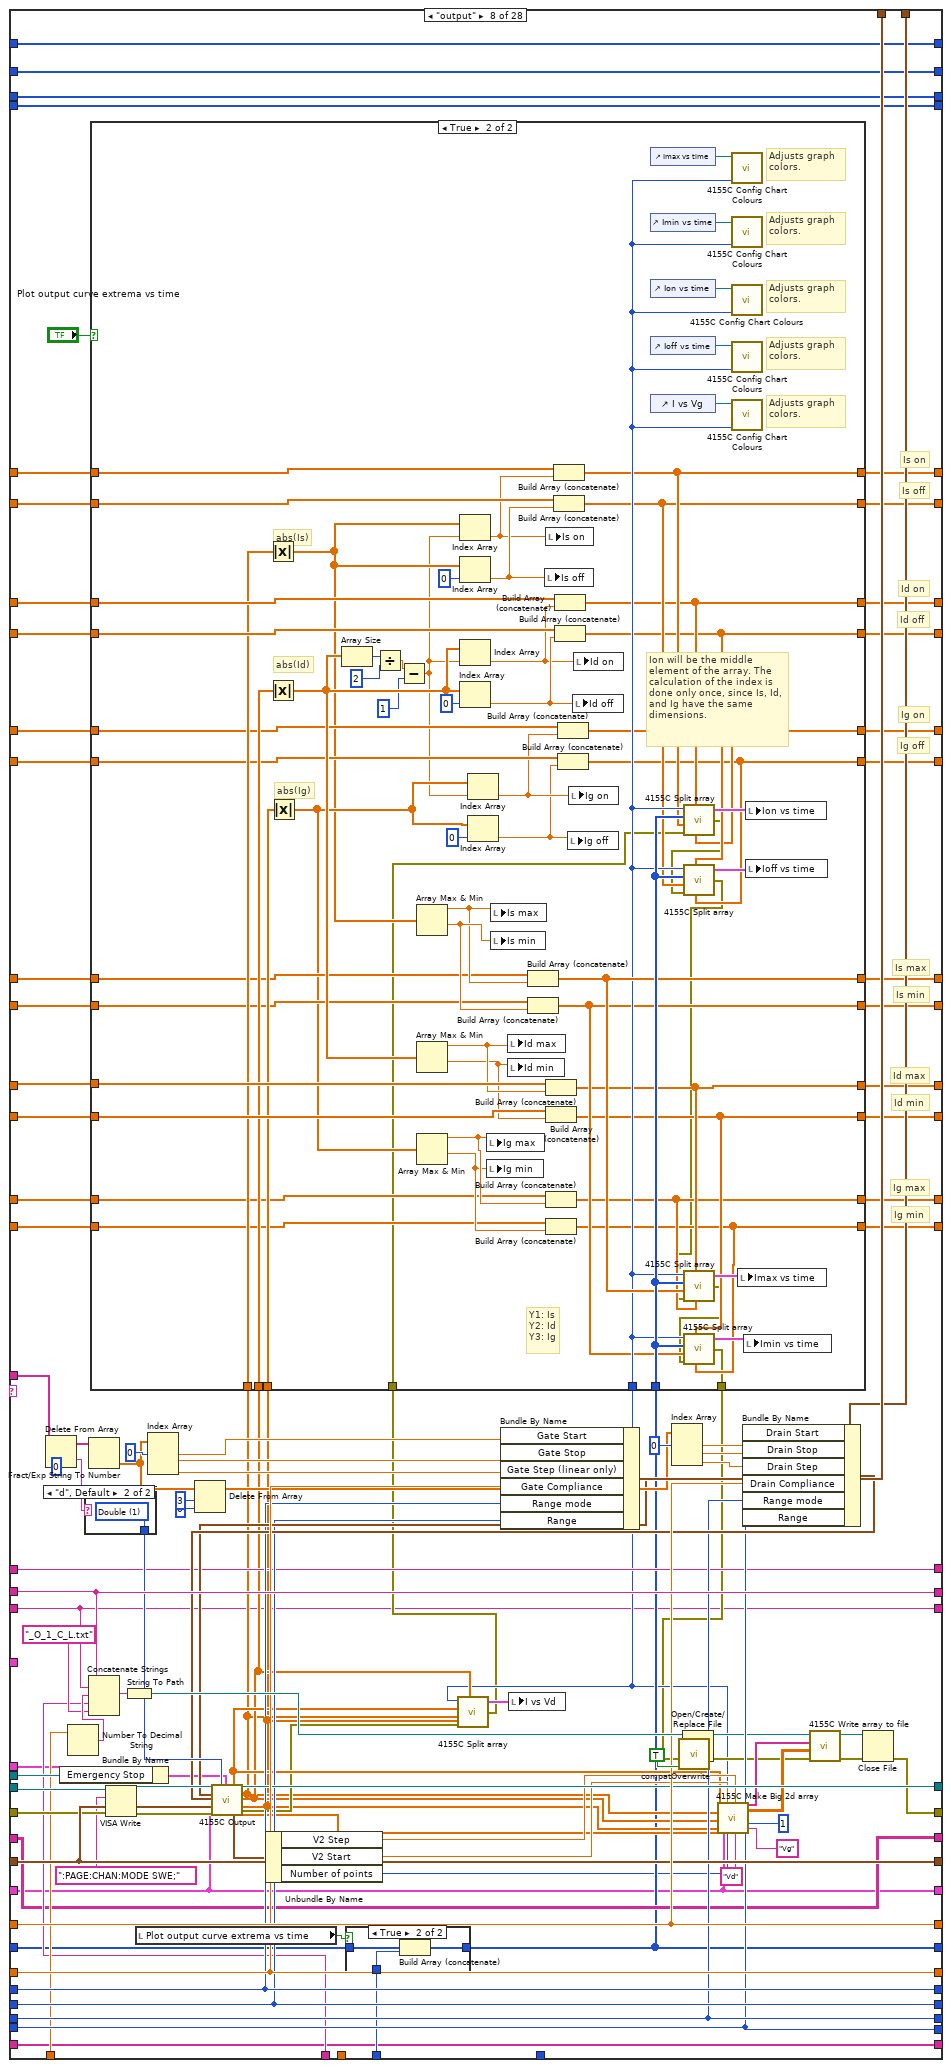
[diagram p19: hidden frame]
diagram:
  w10 = cluster{"Y data in":dbl[], "X data in":dbl[]}[] [] ("I vs Vg")
  w11 = 0.0 ("Is off")
  w12 = 0.0 ("Is on")
  w13 = 0.0 ("Is min")
  w14 = 0.0 ("Is max")
  w63 = u16 1 items=["Reset All", "Partial reset"] ("Type of reset")
  # "Change from previous version:\n\n- Added plotting of \"sample\" plots."
  # "This is a version specific to the SPM pump."
  # "I add 1 to both the \"total lines\" and the \"line running\" indicators because i and N begin from 0, and the script lines begin from 1."
  # "Bugs:\n\n- If using the \"filename\" command, keep in mind that the arrays of the time-dependent data are not re-initialized inbetween filename changes. \n\n- Do not connect the \"error\" wire of a Split block if it has unconnected terminals! It will halt the program."
  # "Array size"
  # "%s option converts a spreadsheet string to an array of strings."
  # "0: No of rows of array\n1: No of cols"
  # "Dimitrios Simatos\nv. 6.6"
  # "Changes from original textcontrol.vi:\n\n- Timestamp appears in filename.\n- (Only) transfer and output curves are plotted.\n- Communication with serial port.\n- Can execute any command, as all pattern matching functions were replaced. Previously, commands with special LabVIEW characters could not be executed.\n- Replaced write to file function with write to text file.\n- Replaced while loop with for loop.\n- Replaced 4155C \"Save File\" function and now the vi can save time-dependent variables.\n- Added clock with start time control and various units.\n- Changed filepath in which the program is saved.\n- Added a serial output log that keeps a history.\n- Tab control.\n- Addition of specialized serial read/write file for the SPM OEM pump.\n- Added halt and hard stop.\n- Added option for plotting transfer and output curve extrema vs time.\n- Corrected bug of \"itime\" command. The command did not allow for settting the integration time value, it allowed to set the category of the integration time (short, medium, long). If the time value was beyond the range of the category, then the SPA used the closest value allowed, whilst staying in the category. So, if the integration time was changed to long, but the integration time value was a short one, then the SPA would measure using the minimum long integration time value and not the value that the user intended.\n- Added SMU4 command."
  # "Search and replace LF with EOL"
  n1 = Equal?(x="integration time", y=u32 0) -> (x = y?=w64:bool)
  n2 = Select(t="Integration time (short)", s=w64, f="Integration time (long)") -> (s? t:f=w15:dbl)
  n3 = call "4155C Get Filename.vi"("error in (no error)"=errorcluster {"status"=FALSE, "code"=0, "source"=""}) -> ("error out"=w58:errorcluster, "path"=w33:path)  [unwired: 2 in, 1 out]
  "Path" <- w33
  n4 = Bundle By Name(cluster="Timings (overwritten by the Front Panel)", "integration time"="integration time", "Short/Long integration time"=w15) -> (w56:T5)
  n5 = Path To String(path=w33) -> (string=w34:string)
  n6 = Search and Replace String(replace all?=TRUE ("replace all? (F)"), input string="Script", search string="\n", replace string="\r\n") -> (result string=w46:string)  [unwired: 4 in, 3 out]
  n7 = Match Pattern(string=w34, regular expression=".txt") -> (before substring=w29:string)  [unwired: 1 in, 3 out]
  n8 = call "4155C Initialise.vi"("VISA resource name in"=refnum<visa-resource-name> "GPIB0::14::INSTR", "Reset"="Full Reset", "Type of reset"=w63, "error in (no error)"=w58, "VISA Timeout Value"=u32 10000) -> ("VISA Resource Name out"=w57:refnum<visa-resource-name>, "error out"=w3:errorcluster)
  n9 = Concatenate Strings(w29, "Suffix (script)") -> (w28:string)
  n10 = Spreadsheet String To Array(delimiter (Tab)="\r\n", format string="%s", spreadsheet string="Script", array type (2D Dbl)="") -> (array=w37:string[][])
  n11 = String To Path(string=w28) -> (path=w6:path)
  n12 = Array Size(array=w37) -> (size(s)=w41:i32[])
  n13 = Initialize Array("") -> (w20:string[])  [unwired: 1 in]
  n14 = Open/Create/Replace File(file path (use dialog)=w6, error in=w3, operation (0:open)=T8."replace or create with confirmation") -> (refnum out=w5:refnum<file>, error out=w4:errorcluster)  [unwired: 3 in, 1 out]
  n15 = Initialize Array(0 ("element")) -> (w22:i32[])  [unwired: 1 in]
  n16 = Initialize Array("") -> (w18:string[][])  [unwired: 2 in]
  n17 = Initialize Array(0.0 ("element")) -> (w24:dbl[])  [unwired: 1 in]
  n18 = Index Array(array=w41, index=0) -> (element=w39:i32)
  n19 = Write to Text File(file (use dialog)=w5, text=w46, error in=w4) -> (error out=w27:errorcluster)  [unwired: 1 in, 2 out]
  n20 = for {
    N: w39 -> [w181]
    shift-left: "Source/Drain Range" -> [w221]
    shift-right: [w217] -> _
    shift-left: "Source/Drain\nRange mode" -> [w222]
    shift-right: [w218] -> _
    shift-left: "Gate Range" -> [w223]
    shift-right: [w219] -> _
    shift-left: "Gate Range\nmode" -> [w224]
    shift-right: [w220] -> _
    shift-left: "Gate: Compliance" -> [w233]
    shift-right: [w229] -> _
    shift-left: "Drain: Compliance" -> [w234]
    shift-right: [w230] -> _
    shift-left: w56 -> [w235]
    shift-right: [w231] -> w16
    shift-left: w27 -> [w236]
    shift-right: [w128] -> w32
    shift-left: w57 -> [w237]
    shift-right: [w232] -> _
    shift-left: w29 -> [w238]
    shift-right: [w132] -> _
    tunnel: "Panel Controls 2" -> [w215]
    shift-right: [w90] -> _
    shift-left: w24 -> [w214]
    shift-right: [w151] -> _
    shift-left: i32[] [] -> [w210]
    tunnel: w37 -> [w209] mode=indexing
    shift-right: [w89] -> _
    shift-left: w24 -> [w186]
    shift-right: [w122] -> _
    shift-left: w20 -> [w173]
    shift-right: [w152] -> _
    shift-left: w22 -> [w168]
    shift-right: [w134] -> _
    shift-left: w22 -> [w167]
    shift-right: [w166] -> _
    shift-left: "" -> [w165]
    shift-right: [w127] -> _
    shift-left: w22 -> [w149]
    shift-right: [w126] -> _
    shift-left: w22 -> [w133]
    shift-right: [w123] -> _
    shift-left: w18 -> [w125]
    shift-right: [w83] -> _
    shift-left: w24 -> [w111]
    shift-right: [w84] -> _
    shift-left: w24 -> [w110]
    shift-right: [w88] -> _
    shift-left: w24 -> [w99]
    shift-right: [w87] -> _
    shift-left: w24 -> [w98]
    shift-right: [w81] -> _
    shift-left: w24 -> [w97]
    shift-right: [w91] -> _
    shift-left: w24 -> [w96]
    shift-right: [w82] -> _
    shift-left: w24 -> [w95]
    shift-right: [w80] -> _
    shift-left: w24 -> [w94]
    shift-right: [w86] -> _
    shift-left: w24 -> [w93]
    shift-right: [w85] -> _
    shift-left: w24 -> [w92]
    shift-right: [w75] -> _
    shift-left: "Filename (variable part)" -> [w74]
    shift-right: [w71] -> w1
    shift-left: "SMU4" -> [w216]
    i -> [w176]
    stop <- "Interrupt program" stop-if-true
    # "Filename prefix"
    # "Is off"
    # "Is on"
    # "Ig off"
    # "Ig on"
    # "Is min"
    # "Is max"
    # "Ig min"
    # "Ig max"
    # "Id min"
    # "Id max"
    # "Id off"
    # "Id on"
    # "Pump status"
    # "Filepath and name"
    # "Pump status"
    # "Limit of command arguments (array columns). Raise if needed."
    # "Serial port data (string)"
    # "Serial port data (table)"
    # "Time array for valve position"
    # "Time array for absolute plunger position"
    # "Valve position"
    # "Absolute plunger position"
    # "Serial port data"
    # "For loop counter"
    # "<-----Equivalent to the 4155C \"Write\" subvi.----->"
    # "Headers"
    # "Save transfer curves in file."
    # "Filepath and name"
    # "Save time-dependent data."
    # "Use the time offset if your measurements do not start at t=0."
    # "Time for Imax, Imin, Ion, Ioff"
    # "Rest of elements of command"
    # "First element of command\n(case select)"
    n21 = Add(x=w176, y=1) -> (x+y=→"Line running":i32)
    n22 = Add(x=w181, y=1) -> (x+y=→"Total lines":i32)
    n23 = Index Array(array=w209, index=0 ("line index")) -> (element=w204:string)
    "Command running:" <- w204
    n24 = control-ref of="Interrupt scan"() -> (w228:refnum<vi>)
    n25 = Spreadsheet String To Array(delimiter (Tab)=" ", format string="%s", spreadsheet string=w204, array type (2D Dbl)=string[] []) -> (array=w202:string[])
    n26 = Delete From Array(array=w202, index=0) -> (deleted portion=w112:string, array with subset deleted=w201:string[])  [unwired: 1 in]
    n27 = call "Elapsed Time"("Reset"="Reset", "Auto Reset"="Auto Reset") -> ("Elapsed Time (s)"=w211:dbl)  [unwired: 10 in, 7 out]
    n28 = case shown="0, Default" "Time Units" {
      tunnel: ["_sec" "_min" "_h"] -> w212
      tunnel: [w242 w246 w249] -> w182
      tunnel: w211 -> [w242 w245 w250]
      frame 0, Default {
      }
      frame 1 {
        n29 = Divide(x=w245, y=60.0) -> (x/y=w246:dbl)
      }
      frame 2 {
        n30 = Divide(x=w250, y=3600.0) -> (x/y=w249:dbl)
      }
    }
    n31 = Add(x=w182, y="Time Offset") -> (x+y=w69:dbl)
    n32 = To Long Integer(number=w69) -> (32bit integer=w70:i32)
    "Elapsed Time" <- w70
    n33 = case shown="\"sample\"" w112 {
      tunnel: w201 -> [w288 w327 w365 w369 w505 w613 w759 w879 w1041 w1069 w1150 w1197 w1242 w1283 w1317 _ _ w1506 w1627 _ w1732 w1796 w1858 w1948 w2030 w2070 w2141 w2196]
      tunnel: w238 -> [w283 w323 w363 w391 w512 w677 w767 w886 w1049 w1092 w1139 w1189 w1235 w1277 w1310 w1349 w1411 w1427 w1609 w1660 w1719 w1783 w1846 w1942 w2026 w2072 w2143 w2198]
      tunnel: w237 -> [w282 w322 w354 w389 w483 w662 w736 w857 w1017 w1093 w1140 w1190 w1236 w1278 w1311 w1354 w1413 w1511 w1633 w1664 w1738 w1802 w1864 w1954 w1984 w2076 w2147 w2200]
      tunnel: w236 -> [w281 w321 w353 w388 w482 w661 w735 w856 w1014 w1094 w1141 w1191 w1237 w1279 w1312 w1353 w1384 w1510 w1632 w1663 w1737 w1801 w1863 w1953 w1983 w2075 w2146 w2201]
      tunnel: w235 -> [w280 w320 w362 w386 w508 w638 w763 w882 w1045 w1102 w1149 w1188 w1234 w1276 w1309 w1352 w1408 w1481 w1601 w1669 w1712 w1776 w1839 w1941 w2025 w2077 w2148 w2203]
      tunnel: w234 -> [w279 w319 w361 w385 w510 w675 w765 w884 w1047 w1101 w1148 w1196 w1241 w1282 w1316 w1351 w1393 w1509 w1631 w1672 w1736 w1800 w1862 w1952 w2034 w2078 w2149 w2204]
      tunnel: w233 -> [w278 w318 w360 w383 w509 w674 w764 w883 w1046 w1100 w1147 w1195 w1240 w1281 w1315 w1350 w1394 w1489 w1610 w1671 w1720 w1784 w1847 w1943 w2027 w2080 w2150 w2206]
      tunnel: [w282 w322 w352 w389 w507 w672 w761 w881 w1043 w1093 w1140 w1190 w1236 w1278 w1311 w1354 w1413 w1482 w1583 w1662 w1713 w1777 w1840 w1894 w1986 w2076 w2147 w2200] -> w232
      tunnel: [w281 w321 w351 w388 w506 w671 w760 w880 w1042 w1094 w1141 w1191 w1237 w1279 w1312 w1353 w1383 w1490 w1584 w1661 w1721 w1785 w1848 w1893 w1985 w2074 w2145 w2201] -> w148
      tunnel: [w280 w320 w362 w386 w508 w634 w763 w882 w1045 w1095 w1142 w1188 w1234 w1276 w1309 w1352 w1408 w1481 w1601 w1669 w1712 w1776 w1839 w1941 w2025 w2077 w2148 w2203] -> w231
      tunnel: [w279 w319 w361 w385 w510 w675 w765 w884 w1047 w1101 w1148 w1196 w1241 w1282 w1316 w1351 w1393 w1509 w1631 w1672 w1736 w1800 w1862 w1952 w2034 w2078 w2149 w2204] -> w230
      tunnel: [w278 w318 w360 w383 w509 w674 w764 w883 w1046 w1100 w1147 w1195 w1240 w1281 w1315 w1350 w1394 w1489 w1610 w1671 w1720 w1784 w1847 w1943 w2027 w2080 w2150 w2206] -> w229
      tunnel: [w283 w323 w363 w391 w512 w677 w767 w886 w1049 w1092 w1139 w1189 w1235 w1277 w1310 w1349 w1411 w1427 w1609 w1660 w1719 w1783 w1846 w1942 w2026 w2072 w2143 w2198] -> w132
      tunnel: w228 -> [_ _ _ _ w514 w681 w772 w888 w1053 _ _ _ _ _ _ _ _ w1486 w1606 _ w1718 w1782 w1845 w1914 w2002 _ _ _]
      tunnel: "Gate" -> [_ _ _ _ w492 w665 w746 w866 w1028 _ _ _ _ _ _ _ _ _ _ _ _ _ _ _ _ _ _ _]
      tunnel: "Drain 2" -> [_ _ _ _ w491 w664 w745 w865 w1027 _ _ _ _ _ _ _ _ _ _ _ _ _ _ _ _ _ _ _]
      tunnel: "Panel Controls" -> [_ _ _ _ _ _ w744 w786 w1026 _ _ _ _ _ _ _ _ _ _ _ _ _ _ _ _ _ _ _]
      tunnel: w224 -> [w277 w317 w359 w382 w476 w655 w729 w850 w1012 w1099 w1146 _ w1233 w1275 w1308 w1348 w1395 w1477 w1597 w1665 w1708 w1772 w1835 w1937 w2021 w2081 w2151 w2207]
      tunnel: w223 -> [w276 w316 w358 w381 w475 w654 w728 w849 w1011 w1098 w1145 w1194 _ w1266 w1314 w1347 w1396 w1478 w1598 w1666 w1709 w1773 w1836 w1938 w2022 w2082 w2152 w2208]
      tunnel: w222 -> [w275 w315 w357 w380 w474 w653 w727 w848 w1010 w1097 w1144 w1193 w1239 w1280 _ w1346 w1397 w1479 w1599 w1667 w1710 w1774 w1837 w1939 w2023 w2083 w2153 w2209]
      tunnel: w221 -> [w274 w314 w356 w379 w473 w652 w726 w847 w1013 w1096 w1143 w1192 w1238 _ w1313 w1345 w1398 w1480 w1600 w1668 w1711 w1775 w1838 w1940 w2024 w2084 w2154 w2210]
      tunnel: [w277 w317 w359 w382 w476 w655 w729 w850 w1012 w1099 w1146 w1187 w1233 w1275 w1308 w1348 w1395 w1477 w1597 w1665 w1708 w1772 w1835 w1937 w2021 w2081 w2151 w2207] -> w220
      tunnel: [w276 w316 w358 w381 w475 w654 w728 w849 w1011 w1098 w1145 w1194 w1225 w1266 w1314 w1347 w1396 w1478 w1598 w1666 w1709 w1773 w1836 w1938 w2022 w2082 w2152 w2208] -> w219
      tunnel: [w275 w315 w357 w380 w474 w653 w727 w848 w1010 w1097 w1144 w1193 w1239 w1280 w1307 w1346 w1397 w1479 w1599 w1667 w1710 w1774 w1837 w1939 w2023 w2083 w2153 w2209] -> w218
      tunnel: [w274 w314 w356 w379 w473 w652 w726 w847 w1013 w1096 w1143 w1192 w1238 w1267 w1313 w1345 w1398 w1480 w1600 w1668 w1711 w1775 w1838 w1940 w2024 w2084 w2154 w2210] -> w217
      tunnel: w216 -> [w252 w289 w328 _ w409 w601 w692 w783 w975 w1066 w1116 w1165 w1203 w1244 w1285 w1323 w1355 w1454 w1557 w1638 w1673 w1741 w1805 w1867 w1955 w2035 w2085 w2194]
      tunnel: w215 -> [_ _ _ _ w467 w649 _ _ _ _ _ _ _ _ _ _ _ _ _ _ _ _ _ _ _ _ _ _]
      tunnel: [w273 w310 w349 w396 w424 w626 w716 w799 w999 w1091 w1137 w1186 w1224 w1265 w1306 w1344 w1379 w1443 w1562 w1659 w1697 w1765 w1829 w1891 w1979 w2073 w2144 w2215] -> w90
      tunnel: w214 -> [w273 w310 w349 w396 w464 w626 w716 w839 w999 w1091 w1137 w1186 w1224 w1265 w1306 w1344 w1379 w1450 w1562 w1659 w1697 w1765 w1829 w1891 w1979 w2073 w2144 w2215]
      tunnel: w69 -> [_ _ _ _ w463 w623 w714 w838 w996 _ _ _ _ _ _ _ w1377 w1470 w1579 _ w1694 w1762 w1826 w1888 w1975 _ _ _]
      tunnel: w212 -> [_ _ _ _ w460 w622 w712 w835 w995 _ _ _ _ _ _ _ w1375 w1468 w1578 _ w1693 w1761 w1825 w1887 w1976 _ w2112 _]
      tunnel: w70 -> [_ _ _ _ w456 _ _ w831 _ _ _ _ _ _ _ _ _ _ _ _ _ _ _ _ _ _ w2115 _]
      tunnel: [w272 w309 w348 w384 w428 w625 w715 w803 w998 w1090 w1136 w1185 w1223 w1264 w1305 w1343 w1378 w1433 w1581 w1658 w1696 w1764 w1828 w1890 w1978 w2079 w2124 w2205] -> w151
      tunnel: w210 -> [w272 w309 w348 w384 w459 w625 w715 w834 w998 w1090 w1136 w1185 w1223 w1264 w1305 w1343 w1378 w1439 w1581 w1658 w1696 w1764 w1828 w1890 w1978 w2079 w2124 w2205]
      tunnel: [w271 w308 w347 w395 w423 w621 w711 w798 w994 w1089 w1135 w1184 w1222 w1263 w1304 w1342 w1374 w1442 w1561 w1657 w1692 w1760 w1824 w1886 w1974 w2068 w2140 w2214] -> w89
      tunnel: w186 -> [w271 w308 w347 w395 w455 w621 w711 w830 w994 w1089 w1135 w1184 w1222 w1263 w1304 w1342 w1374 w1449 w1561 w1657 w1692 w1760 w1824 w1886 w1974 w2068 w2140 w2214]
      tunnel: [w270 w307 w346 w378 w448 w620 w710 w823 w993 w1088 w1134 w1183 w1221 w1262 w1303 w1341 w1373 w1467 w1577 w1656 w1691 w1759 w1823 w1885 w1973 w2067 w2139 w2211] -> w122
      tunnel: w173 -> [w270 w307 w346 w378 w448 w620 w710 w823 w993 w1088 w1134 w1183 w1221 w1262 w1303 w1341 w1373 w1467 w1577 w1656 w1691 w1759 w1823 w1885 w1973 w2066 w2113 w2211]
      tunnel: [w269 w306 w345 w406 w447 w619 w709 w822 w992 w1087 w1133 w1182 w1220 w1261 w1302 w1340 w1372 w1466 w1576 w1655 w1690 w1758 w1822 w1884 w1972 w2052 w2126 w2225] -> w152
      tunnel: w168 -> [w269 w306 w345 w406 w447 w619 w709 w822 w992 w1087 w1133 w1182 w1220 w1261 w1302 w1340 w1372 w1466 w1576 w1655 w1690 w1758 w1822 w1884 w1972 w2052 w2125 w2225]
      tunnel: [w268 w305 w344 w408 w446 w618 w708 w821 w991 w1086 w1132 w1181 w1219 w1260 w1301 w1339 w1371 w1465 w1575 w1654 w1689 w1757 w1821 w1883 w1971 w2051 w2108 w2227] -> w134
      tunnel: w167 -> [w268 w305 w344 w408 w446 w618 w708 w821 w991 w1086 w1132 w1181 w1219 w1260 w1301 w1339 w1371 w1465 w1575 w1654 w1689 w1757 w1821 w1883 w1971 w2051 w2106 w2227]
      tunnel: [w267 w304 w343 w392 w445 w617 w707 w820 w990 w1085 w1131 w1180 w1218 w1259 w1300 w1338 w1370 w1464 w1574 w1653 w1688 w1756 w1820 w1882 w1970 w2050 w2105 w2199] -> w166
      tunnel: w165 -> [w267 w304 w343 w392 w445 w617 w707 w820 w990 w1085 w1131 w1180 w1218 w1259 w1300 w1338 w1370 w1464 w1574 w1653 w1688 w1756 w1820 w1882 w1970 w2050 w2116 w2199]
      tunnel: w70 -> [_ _ _ _ _ _ _ _ _ _ _ _ _ _ _ _ _ _ _ _ _ _ _ _ _ _ w2104 _]
      tunnel: w149 -> [w266 w303 w342 w407 w444 w616 w706 w819 w989 w1084 w1130 w1179 w1217 w1258 w1299 w1337 w1369 w1463 w1573 w1652 w1687 w1755 w1819 w1881 w1969 w2049 w2103 w2226]
      tunnel: [w266 w303 w342 w407 w444 w616 w706 w819 w989 w1084 w1130 w1179 w1217 w1258 w1299 w1337 w1369 w1463 w1573 w1652 w1687 w1755 w1819 w1881 w1969 w2049 w2102 w2226] -> w127
      tunnel: [w265 w302 w341 w405 w443 w615 w705 w818 w988 w1083 w1129 w1178 w1216 w1257 w1298 w1336 w1368 w1462 w1572 w1651 w1686 w1754 w1818 w1880 w1968 w2048 w2101 w2224] -> w126
      tunnel: w133 -> [w265 w302 w341 w405 w443 w615 w705 w818 w988 w1083 w1129 w1178 w1216 w1257 w1298 w1336 w1368 w1462 w1572 w1651 w1686 w1754 w1818 w1880 w1968 w2048 w2100 w2224]
      tunnel: [w264 w301 w340 w387 w442 w614 w704 w817 w987 w1082 w1128 w1177 w1215 w1256 w1297 w1335 w1367 w1461 w1571 w1650 w1685 w1753 w1817 w1879 w1967 w2047 w2098 w2202] -> w123
      tunnel: w125 -> [w264 w301 w340 w387 w442 w614 w704 w817 w987 w1082 w1128 w1177 w1215 w1256 w1297 w1335 w1367 w1461 w1571 w1650 w1685 w1753 w1817 w1879 w1967 w2047 w2097 w2202]
      tunnel: [w262 w299 w338 w401 w417 w611 w702 w792 w985 w1080 w1127 w1176 w1213 w1254 w1295 w1333 w1365 w1460 w1570 w1649 w1684 w1752 w1815 w1878 w1966 w2046 w2096 w2220] -> w83
      tunnel: w111 -> [w262 w299 w338 w401 w441 w611 w702 w816 w985 w1080 w1127 w1176 w1213 w1254 w1295 w1333 w1365 w1460 w1570 w1649 w1684 w1752 w1815 w1878 w1966 w2046 w2096 w2220]
      tunnel: [w263 w300 w339 w402 w418 w612 w703 w793 w986 w1081 w1126 w1175 w1214 w1255 w1296 w1334 w1366 w1459 w1569 w1648 w1683 w1751 w1816 w1877 w1965 w2045 w2095 w2221] -> w84
      tunnel: w110 -> [w263 w300 w339 w402 w440 w612 w703 w815 w986 w1081 w1126 w1175 w1214 w1255 w1296 w1334 w1366 w1459 w1569 w1648 w1683 w1751 w1816 w1877 w1965 w2045 w2095 w2221]
      tunnel: [w255 w292 w331 w394 w422 w608 w700 w797 w983 w1073 w1124 w1173 w1211 w1252 w1293 w1331 w1358 w1441 w1560 w1647 w1676 w1744 w1808 w1870 w1960 w2038 w2094 w2213] -> w88
      tunnel: w99 -> [w255 w292 w331 w394 w436 w608 w700 w811 w983 w1073 w1124 w1173 w1211 w1252 w1293 w1331 w1358 w1448 w1560 w1647 w1676 w1744 w1808 w1870 w1960 w2038 w2094 w2213]
      tunnel: [w254 w291 w330 w393 w421 w609 w701 w796 w984 w1072 w1125 w1174 w1212 w1253 w1294 w1332 w1357 w1440 w1559 w1646 w1675 w1743 w1807 w1869 w1959 w2037 w2093 w2212] -> w87
      tunnel: w98 -> [w254 w291 w330 w393 w435 w609 w701 w810 w984 w1072 w1125 w1174 w1212 w1253 w1294 w1332 w1357 w1447 w1559 w1646 w1675 w1743 w1807 w1869 w1959 w2037 w2093 w2212]
      tunnel: [w257 w294 w333 w398 w427 w607 w698 w802 w981 w1078 w1122 w1171 w1209 w1250 w1291 w1329 w1360 w1445 w1564 w1641 w1678 w1746 w1810 w1872 w1958 w2042 w2091 w2217] -> w81
      tunnel: w97 -> [w257 w294 w333 w398 w434 w607 w698 w809 w981 w1078 w1122 w1171 w1209 w1250 w1291 w1329 w1360 w1452 w1564 w1641 w1678 w1746 w1810 w1872 w1958 w2042 w2091 w2217]
      tunnel: [w256 w293 w332 w397 w425 w610 w699 w800 w982 w1079 w1123 w1172 w1210 w1251 w1292 w1330 w1359 w1444 w1563 w1640 w1677 w1745 w1809 w1871 w1957 w2041 w2092 w2216] -> w91
      tunnel: w96 -> [w256 w293 w332 w397 w433 w610 w699 w808 w982 w1079 w1123 w1172 w1210 w1251 w1292 w1330 w1359 w1451 w1563 w1640 w1677 w1745 w1809 w1871 w1957 w2041 w2092 w2216]
      tunnel: [w259 w296 w335 w400 w416 w606 w696 w791 w979 w1076 w1120 w1169 w1207 w1248 w1289 w1327 w1362 w1456 w1566 w1643 w1680 w1748 w1812 w1874 w1962 w2044 w2089 w2219] -> w82
      tunnel: w95 -> [w259 w296 w335 w400 w432 w606 w696 w807 w979 w1076 w1120 w1169 w1207 w1248 w1289 w1327 w1362 w1456 w1566 w1643 w1680 w1748 w1812 w1874 w1962 w2044 w2089 w2219]
      tunnel: [w258 w295 w334 w399 w415 w605 w697 w790 w980 w1077 w1121 w1170 w1208 w1249 w1290 w1328 w1361 w1455 w1565 w1642 w1679 w1747 w1811 w1873 w1961 w2043 w2090 w2218] -> w80
      tunnel: w94 -> [w258 w295 w334 w399 w431 w605 w697 w806 w980 w1077 w1121 w1170 w1208 w1249 w1290 w1328 w1361 w1455 w1565 w1642 w1679 w1747 w1811 w1873 w1961 w2043 w2090 w2218]
      tunnel: [w261 w298 w337 w404 w420 w604 w694 w795 w977 w1074 w1118 w1167 w1205 w1246 w1287 w1325 w1364 w1458 w1568 w1645 w1682 w1750 w1814 w1876 w1964 w2040 w2087 w2223] -> w86
      tunnel: w93 -> [w261 w298 w337 w404 w430 w604 w694 w805 w977 w1074 w1118 w1167 w1205 w1246 w1287 w1325 w1364 w1458 w1568 w1645 w1682 w1750 w1814 w1876 w1964 w2040 w2087 w2223]
      tunnel: [w260 w297 w336 w403 w419 w603 w695 w794 w978 w1075 w1119 w1168 w1206 w1247 w1288 w1326 w1363 w1457 w1567 w1644 w1681 w1749 w1813 w1875 w1963 w2039 w2088 w2222] -> w85
      tunnel: w92 -> [w260 w297 w336 w403 w429 w603 w695 w804 w978 w1075 w1119 w1168 w1206 w1247 w1288 w1326 w1363 w1457 w1567 w1644 w1681 w1749 w1813 w1875 w1963 w2039 w2088 w2222]
      tunnel: w74 -> [w253 w290 w329 w390 w412 w602 w693 w787 w976 w1071 w1117 w1166 w1204 w1245 w1286 w1324 w1356 w1426 w1558 w1639 w1674 w1742 w1806 w1868 w1956 w2036 w2086 _]
      tunnel: [w253 w290 w329 w390 w412 w602 w693 w787 w976 w1071 w1117 w1166 w1204 w1245 w1286 w1324 w1356 w1426 w1558 w1639 w1674 w1742 w1806 w1868 w1956 w2036 w2086 w2195] -> w75
      tunnel: [w252 w289 w328 w368 w409 w601 w692 w783 w975 w1066 w1116 w1165 w1203 w1244 w1285 w1323 w1355 w1454 w1557 w1638 w1673 w1741 w1805 w1867 w1955 w2035 w2085 w2194] -> w71
      tunnel: w69 -> [_ _ _ _ _ _ _ _ _ _ _ _ _ _ _ _ _ w1424 _ _ _ _ _ _ _ _ _ _]
      frame "wait" {
        n34 = Index Array(array=w288, index=0 ("Index")) -> (element=w286:string)
        n35 = Decimal String To Number(string=w286, default (0L)=u32 0) -> (number=w285:u32)  [unwired: 1 in, 1 out]
        n36 = Wait (ms)(milliseconds to wait=w285) -> ()  [unwired: 1 out]
      }
      frame "wait-min" {
        n37 = Index Array(array=w327, index=0 ("Index")) -> (element=w325:string)
        n38 = Decimal String To Number(string=w325, default (0L)=u32 0) -> (number=w313:u32)  [unwired: 1 in, 1 out]
        n39 = Multiply(x=w313, y=u32 60000) -> (x*y=w312:u32)
        n40 = Wait (ms)(milliseconds to wait=w312) -> ()  [unwired: 1 out]
      }
      frame "standby" {
        n41 = Index Array(array=w365, index=0 ("Index")) -> (element=w355:string)
        n42 = case shown="\"off\", Default" w355 {
          tunnel: [":PAGE:SCON:STAN 0" ":PAGE:SCON:STAN 1"] -> w350
          frame "off", Default {
          }
          frame "on" {
          }
        }
        n43 = VISA Write(VISA resource name=w354, write buffer=w350, error in (no error)=w353) -> (VISA resource name out=w352:refnum<visa-resource-name>, error out=w351:errorcluster)  [unwired: 1 out]
      }
      frame "SMU4" {
        n44 = Delete From Array(array=w369, index=0) -> (deleted portion=w372:string, array with subset deleted=w375:string[])  [unwired: 1 in]
        n45 = Equal?(x=w372, y="ON") -> (x = y?=w370:bool)
        n46 = Delete From Array(array=w375, index=0) -> (deleted portion=w374:string)  [unwired: 1 in, 1 out]
        n47 = Fract/Exp String To Number(string=w374) -> (number=w371:dbl)  [unwired: 3 in, 1 out]
        n48 = Bundle(w370, w371) -> (w368:cluster{bool, dbl})  [unwired: 1 in]
      }
      frame "transfer" {
        # "Is off"
        # "Is on"
        # "Ig off"
        # "Ig on"
        # "Is min"
        # "Is max"
        # "Ig min"
        # "Ig max"
        # "Id min"
        # "Id max"
        # "Id off"
        # "Id on"
        n49 = Delete From Array(array=w505, index=0 ("Index")) -> (deleted portion=w503:string, array with subset deleted=w502:string[])  [unwired: 1 in]
        n50 = Bundle By Name(cluster=w467, "Emergency Stop"=w514) -> (w468:T2)
        n51 = Number To Decimal String(number=w463) -> (decimal integer string=w462:string)  [unwired: 1 in]
        n52 = case shown="\"d\", Default" w503 {
          tunnel: [w599 w600] -> w501
          frame "s" {
            w599 = u16 0 items=["Single", "Double"] ("sweep mode")
          }
          frame "d", Default {
            w600 = u16 1 items=["Single", "Double"] ("sweep mode")
          }
        }
        n53 = Fract/Exp String To Number(string=w502) -> (number=w487:dbl[])  [unwired: 3 in, 1 out]
        n54 = Concatenate Strings(w512, w412, w462, w460, "_T_1_C_L.txt" ("Suffix (transfer)")) -> (w513:string)
        n55 = VISA Write(VISA resource name=w483, write buffer=":PAGE:CHAN:MODE SWE;" ("write buffer (\"\")"), error in (no error)=w482) -> (VISA resource name out=w480:refnum<visa-resource-name>, error out=w481:errorcluster)  [unwired: 1 out]
        n56 = local read "Plot transfer curve extrema vs time"() -> (w410:bool)
        n57 = String To Path(string=w513) -> (path=w511:path)
        n58 = Index Array(array=w487, index #1=0 ("Index")) -> (element #1=w500:dbl, element #2=w499:dbl, element #3=w498:dbl)  [unwired: 2 in]
        n59 = Delete From Array(array=w487, length=3 ("Length"), index=0 ("Index")) -> (array with subset deleted=w485:dbl[])  [unwired: 1 out]
        n60 = case shown="True" w410 {
          tunnel: w459 -> [w516 w519]
          tunnel: w456 -> [_ w518]
          tunnel: [w516 w517] -> w428
          frame False {
          }
          frame True {
            n61 = Build Array (concatenate)(w519, w518) -> (w517:i32[])
          }
        }
        n62 = Bundle By Name(cluster=w492, "Gate Start"=w500, "Gate Stop"=w499, "Gate Step (linear only)"=w498, "Gate Compliance"=w509, "Range mode"=w476, "Range"=w475) -> (w477:T6)
        n63 = Index Array(array=w485, index #1=0 ("Index")) -> (element #1=w495:dbl, element #2=w494:dbl, element #3=w493:dbl)  [unwired: 2 in]
        n64 = call <vilib>:"compatOverwrite.vi"("overwrite (F)"=TRUE) -> ("overwrite?"=w466:T8)
        n65 = Bundle By Name(cluster=w491, "Drain Start"=w495, "Drain Stop"=w494, "Drain Step"=w493, "Drain Compliance"=w510, "Range mode"=w474, "Range"=w473) -> (w478:T7)
        n66 = call "4155C Transfer.vi"("VISA resource name in"=w480, "Gate"=w477, "Drain"=w478, "Timings"=w508, "error in (no error)"=w481, "SMU4"=w409, "sweep mode"=w501, "Panel Controls"=w468) -> ("VG"=w465:dbl[], "Outparams"=w472:T9, "VISA Resource Name out"=w507:refnum<visa-resource-name>, "IS"=w438:dbl[], "ID"=w439:dbl[], "IG"=w437:dbl[], "error out"=w457:errorcluster, "SMU4"=w469:dbl[])  [unwired: 12 in]
        n67 = Unbundle By Name(w472) -> ("V2 Step"=w471:dbl, "V2 Start"=w470:dbl, "Number of points"=w426:i32)
        n68 = call "4155C Split array.vi"("Number of VAR2 steps"=w426, "Y2 data in"=w439, "X data in"=w465, "Y1 data in"=w438, "Y3 data in"=w437, "error in (no error)"=w457) -> ("Array of clusters"=w458:cluster{"Y data in":dbl[], "X data in":dbl[]}[], "error out"=w414:errorcluster)  [unwired: 1 in]
        n69 = case shown="True" "Plot transfer curve extrema vs time" {
          tunnel: w464 -> [w528 w598]
          tunnel: w455 -> [w529 w593]
          tunnel: w441 -> [w522 w589]
          tunnel: w440 -> [w523 w588]
          tunnel: w439 -> [_ w585]
          tunnel: w438 -> [_ w583]
          tunnel: w437 -> [_ w582]
          tunnel: w436 -> [w530 w578]
          tunnel: w435 -> [w531 w577]
          tunnel: w434 -> [w526 w574]
          tunnel: w433 -> [w527 w573]
          tunnel: w432 -> [w521 w570]
          tunnel: w431 -> [w520 w569]
          tunnel: w430 -> [w525 w566]
          tunnel: w429 -> [w524 w565]
          tunnel: w428 -> [_ w558]
          tunnel: [w526 w553] -> w427
          tunnel: w426 -> [_ w552]
          tunnel: [w527 w551] -> w425
          tunnel: [w528 w550] -> w424
          tunnel: [w529 w549] -> w423
          tunnel: [w530 w548] -> w422
          tunnel: [w531 w547] -> w421
          tunnel: [w525 w546] -> w420
          tunnel: [w524 w545] -> w419
          tunnel: [w523 w544] -> w418
          tunnel: [w522 w543] -> w417
          tunnel: [w521 w542] -> w416
          tunnel: [w520 w541] -> w415
          tunnel: w414 -> [w532 w540]
          tunnel: [w532 w536] -> w413
          frame False {
          }
          frame True {
            # "Adjusts graph colors."
            # "Adjusts graph colors."
            # "Ion will be the middle element of the array. The calculation of the index is done only once, since Is, Id, and Ig have the same dimensions."
            # "abs(Ig)"
            # "abs(Is)"
            # "Y1: Is\nY2: Id\nY3: Ig"
            # "abs(Id)"
            # "Adjusts graph colors."
            # "Adjusts graph colors."
            # "Adjusts graph colors."
            n70 = Absolute Value(x=w583) -> (abs(x)=w568:dbl[])
            n71 = Absolute Value(x=w585) -> (abs(x)=w584:dbl[])
            n72 = Absolute Value(x=w582) -> (abs(x)=w571:dbl[])
            n73 = Array Size(array=w584) -> (size(s)=w592:i32)
            n74 = Divide(x=w592, y=2) -> (x/y=w535:dbl)
            n75 = Subtract(x=w535, y=1) -> (x-y=w534:dbl)
            n76 = Array Max & Min(array=w568) -> (max value=w575:dbl, min value=w576:dbl)  [unwired: 2 out]
            n77 = Array Max & Min(array=w584) -> (max value=w597:dbl, min value=w581:dbl)  [unwired: 2 out]
            n78 = Array Max & Min(array=w571) -> (max value=w580:dbl, min value=w579:dbl)  [unwired: 2 out]
            n79 = Index Array(array=w568, index=w534) -> (element=w559:dbl)
            n80 = Index Array(array=w568, index=0) -> (element=w560:dbl)
            n81 = Index Array(array=w584, index=w534) -> (element=w561:dbl)
            n82 = Index Array(array=w584, index=0) -> (element=w562:dbl)
            n83 = Index Array(array=w571, index=w534) -> (element=w564:dbl)
            n84 = Index Array(array=w571, index=0) -> (element=w563:dbl)
            n85 = local write "Ig max"(w580) -> ()
            n86 = local write "Ig min"(w579) -> ()
            n87 = local write "Is max"(w575) -> ()
            n88 = local write "Is min"(w576) -> ()
            n89 = local write "Id max"(w597) -> ()
            n90 = local write "Id min"(w581) -> ()
            n91 = Build Array (concatenate)(w574, w575) -> (w553:dbl[])
            n92 = Build Array (concatenate)(w573, w576) -> (w551:dbl[])
            n93 = local write "Is off"(w560) -> ()
            n94 = local write "Is on"(w559) -> ()
            n95 = Build Array (concatenate)(w598, w597) -> (w550:dbl[])
            n96 = Build Array (concatenate)(w593, w581) -> (w549:dbl[])
            n97 = Build Array (concatenate)(w578, w580) -> (w548:dbl[])
            n98 = Build Array (concatenate)(w577, w579) -> (w547:dbl[])
            n99 = Build Array (concatenate)(w566, w559) -> (w546:dbl[])
            n100 = Build Array (concatenate)(w565, w560) -> (w545:dbl[])
            n101 = Build Array (concatenate)(w588, w561) -> (w544:dbl[])
            n102 = Build Array (concatenate)(w589, w562) -> (w543:dbl[])
            n103 = Build Array (concatenate)(w570, w564) -> (w542:dbl[])
            n104 = Build Array (concatenate)(w569, w563) -> (w541:dbl[])
            n105 = local write "Ig off"(w563) -> ()
            n106 = local write "Ig on"(w564) -> ()
            n107 = local write "Id off"(w562) -> ()
            n108 = local write "Id on"(w561) -> ()
            n109 = control-ref of="Imax vs time"() -> (w587:refnum<vi>)
            n110 = control-ref of="Imin vs time"() -> (w586:refnum<vi>)
            n111 = control-ref of="Ion vs time"() -> (w555:refnum<vi>)
            n112 = control-ref of="Ioff vs time"() -> (w554:refnum<vi>)
            n113 = control-ref of="I vs Vg"() -> (w596:refnum<vi>)
            n114 = call "4155C Split array.vi"("Number of VAR2 steps"=w552, "Y2 data in"=w544, "X data in"=w558, "Y1 data in"=w546, "Y3 data in"=w542, "error in (no error)"=w540) -> ("Array of clusters"=w556:cluster{"Y data in":dbl[], "X data in":dbl[]}[], "error out"=w539:errorcluster)  [unwired: 1 in]
            n115 = call "4155C Split array.vi"("Number of VAR2 steps"=w552, "Y2 data in"=w543, "X data in"=w558, "Y1 data in"=w545, "Y3 data in"=w541, "error in (no error)"=w539) -> ("Array of clusters"=w557:cluster{"Y data in":dbl[], "X data in":dbl[]}[], "error out"=w538:errorcluster)  [unwired: 1 in]
            n116 = call "4155C Split array.vi"("Number of VAR2 steps"=w552, "Y2 data in"=w550, "X data in"=w558, "Y1 data in"=w553, "Y3 data in"=w548, "error in (no error)"=w538) -> ("Array of clusters"=w595:cluster{"Y data in":dbl[], "X data in":dbl[]}[], "error out"=w537:errorcluster)  [unwired: 1 in]
            n117 = call "4155C Split array.vi"("Number of VAR2 steps"=w552, "Y2 data in"=w549, "X data in"=w558, "Y1 data in"=w551, "Y3 data in"=w547, "error in (no error)"=w537) -> ("Array of clusters"=w594:cluster{"Y data in":dbl[], "X data in":dbl[]}[], "error out"=w536:errorcluster)  [unwired: 1 in]
            n118 = call "4155C Config Chart Colours.vi"("Numeric"=w552, "XY Graph 2"=w587) -> ()  [unwired: 6 in]
            n119 = call "4155C Config Chart Colours.vi"("Numeric"=w552, "XY Graph 2"=w586) -> ()  [unwired: 6 in]
            n120 = call "4155C Config Chart Colours.vi"("Numeric"=w552, "XY Graph 2"=w555) -> ()  [unwired: 6 in]
            n121 = call "4155C Config Chart Colours.vi"("Numeric"=w552, "XY Graph 2"=w554) -> ()  [unwired: 6 in]
            n122 = call "4155C Config Chart Colours.vi"("Numeric"=w552, "XY Graph 2"=w596) -> ()  [unwired: 6 in]
            n123 = local write "Imax vs time"(w595) -> ()
            n124 = local write "Imin vs time"(w594) -> ()
            n125 = local write "Ion vs time"(w556) -> ()
            n126 = local write "Ioff vs time"(w557) -> ()
          }
        }
        n127 = local write "I vs Vg"(w458) -> ()
        n128 = Open/Create/Replace File(file path (use dialog)=w511, error in=w413, operation (0:open)=w466) -> (refnum out=w453:refnum<file>, error out=w451:errorcluster)  [unwired: 3 in, 1 out]
        n129 = call "4155C Make Big 2d array.vi"("1D Var1"=w465, "1d IS"=w438, "1d ID"=w439, "1d IG"=w437, "1d SMU4"=w469, "SMU4"=w409, "VAR2 START"=w470, "Number of VAR2 steps"=w426, "VAR2 STEP"=w471, "VAR1 Name"="Vg", "Decimal places in header"=i8 1, "VAR2 Name"="Vd") -> ("Header array"=w454:string[], "Data array"=w452:dbl[][])  [unwired: 14 in]
        n130 = call "4155C Write array to file.vi"("Byte Stream File Refnum"=w453, "Header"=w454, "Data Array"=w452, "error in (no error)"=w451) -> ("dup refnum"=w450:refnum<file>, "error out"=w449:errorcluster)  [unwired: 1 in]
        n131 = Close File(refnum=w450, error in=w449) -> (error out=w506:errorcluster)  [unwired: 1 out]
      }
      frame "pulsedstressV" {
        w632 = 0
        n132 = Number To Decimal String(number=w623) -> (decimal integer string=w678:string)  [unwired: 1 in]
        n133 = Delete From Array(array=w613, index=0 ("Index")) -> (deleted portion=w669:string, array with subset deleted=w668:string[])  [unwired: 1 in]
        n134 = Bundle By Name(cluster=w649, "Emergency Stop"=w681) -> (w650:T2)
        n135 = VISA Write(VISA resource name=w662, write buffer=":PAGE:CHAN:MODE SWE;" ("write buffer (\"\")"), error in (no error)=w661) -> (VISA resource name out=w659:refnum<visa-resource-name>, error out=w660:errorcluster)  [unwired: 1 out]
        n136 = Concatenate Strings(w677, "-pulsedstressV-" ("Substring"), w678, w622, ".txt" ("Substring")) -> (w680:string)
        n137 = case shown="\"d\", Default" w669 {
          tunnel: [w690 w691] -> w667
          frame "s" {
            w690 = u16 0 items=["Single", "Double"] ("sweep mode")
          }
          frame "d", Default {
            w691 = u16 1 items=["Single", "Double"] ("sweep mode")
          }
        }
        n138 = Fract/Exp String To Number(string=w668) -> (number=w663:dbl[])  [unwired: 3 in, 1 out]
        n139 = String To Path(string=w680) -> (path=w676:path)
        n140 = Index Array(array=w663, index #1=0 ("Index")) -> (element #1=w641:dbl, element #2=w640:dbl, element #3=w637:dbl, element #4=w636:dbl, element #5=w635:dbl, element #6=w639:dbl)  [unwired: 5 in]
        n141 = Bundle By Name(cluster=w638, "Pulse period"=w636, "Base voltage"=w637, "Pulse width"=w635) -> (w634:T5)
        n142 = Unbundle By Name(w634) -> ("Pulse period"=w642:dbl)
        n143 = Bundle By Name(cluster=w665, "Gate Start"=w640, "Gate Stop"=w641, "Gate Step (linear only)"=0, "Gate Compliance"=w674, "Range mode"=w655, "Range"=w654) -> (w656:T6)
        n144 = call <vilib>:"compatOverwrite.vi"("overwrite (F)"=TRUE) -> ("overwrite?"=w627:T8)
        n145 = Bundle By Name(cluster=w664, "Drain Start"=w639, "Drain Stop"=w632, "Drain Step"=w632, "Drain Compliance"=w675, "Range mode"=w653, "Range"=w652) -> (w657:T7)
        n146 = call "4155C PulsedStressV.vi"("VISA resource name in"=w659, "sweep mode"=w667, "Panel Controls"=w650, "Gate"=w656, "Drain"=w657, "Timings"=w634, "error in (no error)"=w660, "SMU4"=w601) -> ("VISA Resource Name out"=w672:refnum<visa-resource-name>, "ID"=w630:dbl[], "IG"=w628:dbl[], "Outparams"=w651:T9, "error out"=w673:errorcluster)  [unwired: 3 in]
        n147 = Unbundle By Name(w651) -> ("Number of points"=w629:i32)  [unwired: 2 out]
        n148 = for {
          N: w629 -> [_]
          tunnel: [w687] -> w631 mode=indexing
          tunnel: w642 -> [w689]
          i -> [w688]
          n149 = Multiply(x=w689, y=w688) -> (x*y=w687:dbl)
        }
        n150 = Insert Into Array(array=dbl[][] [] ("Input Array"), new element=w631) -> (w643:dbl[][])  [unwired: 2 in]
        n151 = Insert Into Array(array=w643, new element=w630) -> (w648:dbl[][])  [unwired: 2 in]
        n152 = Insert Into Array(array=w648, new element=w628) -> (w647:dbl[][])  [unwired: 2 in]
        n153 = Transpose 2D Array(2D array=w647) -> (transposed array=w646:dbl[][])
        n154 = Open/Create/Replace File(file path (use dialog)=w676, error in=w673, operation (0:open)=w627) -> (refnum out=w684:refnum<file>, error out=w685:errorcluster)  [unwired: 3 in, 1 out]
        n155 = call "4155C Write array to file.vi"("Byte Stream File Refnum"=w684, "Header"=string[] ["Time /s", "Id /A", "Ig /A"], "Data Array"=w646, "error in (no error)"=w685) -> ("dup refnum"=w682:refnum<file>, "error out"=w683:errorcluster)  [unwired: 1 in]
        n156 = Close File(refnum=w682, error in=w683) -> (error out=w671:errorcluster)  [unwired: 1 out]
      }
      frame "transfer-fpp" {
        n157 = Number To Decimal String(number=w714) -> (decimal integer string=w768:string)  [unwired: 1 in]
        n158 = Bundle By Name(cluster=w744, "Emergency Stop"=w772) -> (w780:T1)
        n159 = Delete From Array(array=w759, index=0 ("Index")) -> (deleted portion=w757:string, array with subset deleted=w756:string[])  [unwired: 1 in]
        n160 = Concatenate Strings(w767, "-transferfpp-" ("Substring"), w768, w712, ".txt" ("Substring")) -> (w770:string)
        n161 = VISA Write(VISA resource name=w736, write buffer=":PAGE:CHAN:MODE SWE;" ("write buffer (\"\")"), error in (no error)=w735) -> (VISA resource name out=w733:refnum<visa-resource-name>, error out=w734:errorcluster)  [unwired: 1 out]
        n162 = case shown="\"d\", Default" w757 {
          tunnel: [w781 w782] -> w755
          frame "s" {
            w781 = u16 0 items=["Single", "Double"] ("sweep mode")
          }
          frame "d", Default {
            w782 = u16 1 items=["Single", "Double"] ("sweep mode")
          }
        }
        n163 = Fract/Exp String To Number(string=w756) -> (number=w740:dbl[])  [unwired: 3 in, 1 out]
        n164 = String To Path(string=w770) -> (path=w766:path)
        n165 = Index Array(array=w740, index #1=0 ("Index")) -> (element #1=w754:dbl, element #2=w753:dbl, element #3=w752:dbl)  [unwired: 2 in]
        n166 = Delete From Array(array=w740, length=3 ("Length"), index=0 ("Index")) -> (array with subset deleted=w738:dbl[])  [unwired: 1 out]
        n167 = Bundle By Name(cluster=w746, "Gate Start"=w754, "Gate Stop"=w753, "Gate Step (linear only)"=w752, "Gate Compliance"=w764, "Range mode"=w729, "Range"=w728) -> (w730:T6)
        n168 = Index Array(array=w738, index #1=0 ("Index")) -> (element #1=w749:dbl, element #2=w748:dbl, element #3=w747:dbl)  [unwired: 2 in]
        n169 = call <vilib>:"compatOverwrite.vi"("overwrite (F)"=TRUE) -> ("overwrite?"=w717:T8)
        n170 = Bundle By Name(cluster=w745, "Drain Start"=w749, "Drain Stop"=w748, "Drain Step"=w747, "Drain Compliance"=w765, "Range mode"=w727, "Range"=w726) -> (w731:T7)
        n171 = call "4155C Transfer-FPP.vi"("VISA resource name in"=w733, "Gate"=w730, "Drain"=w731, "Timings"=w763, "error in (no error)"=w734, "sweep mode"=w755, "Panel Controls"=w780) -> ("VG"=w771:dbl[], "Outparams"=w725:T9, "VISA Resource Name out"=w761:refnum<visa-resource-name>, "Vprobe2"=w721:dbl[], "ID"=w720:dbl[], "IG"=w719:dbl[], "Vprobe1"=w718:dbl[], "error out"=w762:errorcluster)  [unwired: 13 in]
        n172 = Unbundle By Name(w725) -> ("V2 Step"=w724:dbl, "V2 Start"=w723:dbl, "Number of points"=w722:i32)
        n173 = Open/Create/Replace File(file path (use dialog)=w766, error in=w762, operation (0:open)=w717) -> (refnum out=w777:refnum<file>, error out=w778:errorcluster)  [unwired: 3 in, 1 out]
        n174 = call "4155C Make Big 2d array FPP.vi"("1D Var1"=w771, "1d ID"=w720, "1d Vp2"=w721, "1d IG"=w719, "1d Vp1"=w718, "VAR2 START"=w723, "Number of VAR2 steps"=w722, "VAR2 STEP"=w724, "VAR1 Name"="Vg", "Decimal places in header"=i8 1, "VAR2 Name"="Vd") -> ("Header array"=w773:string[], "Data array"=w774:dbl[][])  [unwired: 15 in]
        n175 = call "4155C Write array to file.vi"("Byte Stream File Refnum"=w777, "Header"=w773, "Data Array"=w774, "error in (no error)"=w778) -> ("dup refnum"=w775:refnum<file>, "error out"=w776:errorcluster)  [unwired: 1 in]
        n176 = Close File(refnum=w775, error in=w776) -> (error out=w760:errorcluster)  [unwired: 1 out]
      }
      frame "output" {
        # "Is off"
        # "Is on"
        # "Ig off"
        # "Ig on"
        # "Is min"
        # "Is max"
        # "Ig min"
        # "Ig max"
        # "Id min"
        # "Id max"
        # "Id off"
        # "Id on"
        n177 = Delete From Array(array=w879, index=0 ("Index")) -> (deleted portion=w877:string, array with subset deleted=w876:string[])  [unwired: 1 in]
        n178 = Bundle By Name(cluster=w786, "Emergency Stop"=w888) -> (w842:T1)
        n179 = Number To Decimal String(number=w838) -> (decimal integer string=w837:string)  [unwired: 1 in]
        n180 = case shown="\"d\", Default" w877 {
          tunnel: [w973 w974] -> w875
          frame "s" {
            w973 = u16 0 items=["Single", "Double"] ("sweep mode")
          }
          frame "d", Default {
            w974 = u16 1 items=["Single", "Double"] ("sweep mode")
          }
        }
        n181 = Fract/Exp String To Number(string=w876) -> (number=w861:dbl[])  [unwired: 3 in, 1 out]
        n182 = Concatenate Strings(w886, w787, w837, w835, "_O_1_C_L.txt" ("Suffix (transfer)")) -> (w887:string)
        n183 = VISA Write(VISA resource name=w857, write buffer=":PAGE:CHAN:MODE SWE;" ("write buffer (\"\")"), error in (no error)=w856) -> (VISA resource name out=w854:refnum<visa-resource-name>, error out=w855:errorcluster)  [unwired: 1 out]
        n184 = String To Path(string=w887) -> (path=w885:path)
        n185 = local read "Plot output curve extrema vs time"() -> (w784:bool)
        n186 = Index Array(array=w861, index #1=0 ("Index")) -> (element #1=w874:dbl, element #2=w873:dbl, element #3=w872:dbl)  [unwired: 2 in]
        n187 = Delete From Array(array=w861, length=3 ("Length"), index=0 ("Index")) -> (array with subset deleted=w859:dbl[])  [unwired: 1 out]
        n188 = case shown="True" w784 {
          tunnel: w834 -> [w890 w893]
          tunnel: w831 -> [_ w892]
          tunnel: [w890 w891] -> w803
          frame False {
          }
          frame True {
            n189 = Build Array (concatenate)(w893, w892) -> (w891:i32[])
          }
        }
        n190 = Bundle By Name(cluster=w866, "Gate Start"=w874, "Gate Stop"=w873, "Gate Step (linear only)"=w872, "Gate Compliance"=w883, "Range mode"=w850, "Range"=w849) -> (w851:T6)
        n191 = Index Array(array=w859, index #1=0 ("Index")) -> (element #1=w869:dbl, element #2=w868:dbl, element #3=w867:dbl)  [unwired: 2 in]
        n192 = call <vilib>:"compatOverwrite.vi"("overwrite (F)"=TRUE) -> ("overwrite?"=w841:T8)
        n193 = Bundle By Name(cluster=w865, "Drain Start"=w869, "Drain Stop"=w868, "Drain Step"=w867, "Drain Compliance"=w884, "Range mode"=w848, "Range"=w847) -> (w852:T7)
        n194 = call "4155C Output.vi"("VISA resource name in"=w854, "Gate"=w851, "Drain"=w852, "Timings"=w882, "error in (no error)"=w855, "SMU4"=w783, "sweep mode"=w875, "Panel controls"=w842) -> ("VD"=w840:dbl[], "Outparams"=w846:T9, "VISA Resource Name out"=w881:refnum<visa-resource-name>, "IS"=w813:dbl[], "ID"=w814:dbl[], "IG"=w812:dbl[], "error out"=w832:errorcluster, "SMU4"=w843:dbl[])  [unwired: 12 in]
        n195 = Unbundle By Name(w846) -> ("V2 Step"=w845:dbl, "V2 Start"=w844:dbl, "Number of points"=w801:i32)
        n196 = call "4155C Split array.vi"("Number of VAR2 steps"=w801, "Y2 data in"=w814, "X data in"=w840, "Y1 data in"=w813, "Y3 data in"=w812, "error in (no error)"=w832) -> ("Array of clusters"=w833:cluster{"Y data in":dbl[], "X data in":dbl[]}[], "error out"=w789:errorcluster)  [unwired: 1 in]
        n197 = case shown="True" "Plot output curve extrema vs time" {
          tunnel: w839 -> [w897 w972]
          tunnel: w830 -> [w896 w967]
          tunnel: w816 -> [w902 w963]
          tunnel: w815 -> [w903 w962]
          tunnel: w814 -> [_ w959]
          tunnel: w813 -> [_ w957]
          tunnel: w812 -> [_ w956]
          tunnel: w811 -> [w895 w952]
          tunnel: w810 -> [w894 w951]
          tunnel: w809 -> [w899 w948]
          tunnel: w808 -> [w898 w947]
          tunnel: w807 -> [w901 w944]
          tunnel: w806 -> [w900 w943]
          tunnel: w805 -> [w905 w940]
          tunnel: w804 -> [w904 w939]
          tunnel: w803 -> [_ w932]
          tunnel: [w899 w927] -> w802
          tunnel: w801 -> [_ w926]
          tunnel: [w898 w925] -> w800
          tunnel: [w897 w924] -> w799
          tunnel: [w896 w923] -> w798
          tunnel: [w895 w922] -> w797
          tunnel: [w894 w921] -> w796
          tunnel: [w905 w920] -> w795
          tunnel: [w904 w919] -> w794
          tunnel: [w903 w918] -> w793
          tunnel: [w902 w917] -> w792
          tunnel: [w901 w916] -> w791
          tunnel: [w900 w915] -> w790
          tunnel: w789 -> [w906 w914]
          tunnel: [w906 w910] -> w788
          frame False {
          }
          frame True {
            # "Adjusts graph colors."
            # "Adjusts graph colors."
            # "Ion will be the middle element of the array. The calculation of the index is done only once, since Is, Id, and Ig have the same dimensions."
            # "abs(Ig)"
            # "abs(Is)"
            # "Y1: Is\nY2: Id\nY3: Ig"
            # "abs(Id)"
            # "Adjusts graph colors."
            # "Adjusts graph colors."
            # "Adjusts graph colors."
            n198 = Absolute Value(x=w957) -> (abs(x)=w942:dbl[])
            n199 = Absolute Value(x=w959) -> (abs(x)=w958:dbl[])
            n200 = Absolute Value(x=w956) -> (abs(x)=w945:dbl[])
            n201 = Array Size(array=w958) -> (size(s)=w966:i32)
            n202 = Divide(x=w966, y=2) -> (x/y=w909:dbl)
            n203 = Subtract(x=w909, y=1) -> (x-y=w908:dbl)
            n204 = Array Max & Min(array=w942) -> (max value=w949:dbl, min value=w950:dbl)  [unwired: 2 out]
            n205 = Array Max & Min(array=w958) -> (max value=w971:dbl, min value=w955:dbl)  [unwired: 2 out]
            n206 = Array Max & Min(array=w945) -> (max value=w954:dbl, min value=w953:dbl)  [unwired: 2 out]
            n207 = Index Array(array=w942, index=w908) -> (element=w933:dbl)
            n208 = Index Array(array=w942, index=0) -> (element=w934:dbl)
            n209 = Index Array(array=w958, index=w908) -> (element=w935:dbl)
            n210 = Index Array(array=w958, index=0) -> (element=w936:dbl)
            n211 = Index Array(array=w945, index=w908) -> (element=w938:dbl)
            n212 = Index Array(array=w945, index=0) -> (element=w937:dbl)
            n213 = local write "Ig max"(w954) -> ()
            n214 = local write "Ig min"(w953) -> ()
            n215 = local write "Is max"(w949) -> ()
            n216 = local write "Is min"(w950) -> ()
            n217 = local write "Id max"(w971) -> ()
            n218 = local write "Id min"(w955) -> ()
            n219 = Build Array (concatenate)(w948, w949) -> (w927:dbl[])
            n220 = Build Array (concatenate)(w947, w950) -> (w925:dbl[])
            n221 = local write "Is off"(w934) -> ()
            n222 = local write "Is on"(w933) -> ()
            n223 = Build Array (concatenate)(w972, w971) -> (w924:dbl[])
            n224 = Build Array (concatenate)(w967, w955) -> (w923:dbl[])
            n225 = Build Array (concatenate)(w952, w954) -> (w922:dbl[])
            n226 = Build Array (concatenate)(w951, w953) -> (w921:dbl[])
            n227 = Build Array (concatenate)(w940, w933) -> (w920:dbl[])
            n228 = Build Array (concatenate)(w939, w934) -> (w919:dbl[])
            n229 = Build Array (concatenate)(w962, w935) -> (w918:dbl[])
            n230 = Build Array (concatenate)(w963, w936) -> (w917:dbl[])
            n231 = Build Array (concatenate)(w944, w938) -> (w916:dbl[])
            n232 = Build Array (concatenate)(w943, w937) -> (w915:dbl[])
            n233 = local write "Ig off"(w937) -> ()
            n234 = local write "Ig on"(w938) -> ()
            n235 = local write "Id off"(w936) -> ()
            n236 = local write "Id on"(w935) -> ()
            n237 = control-ref of="Imax vs time"() -> (w961:refnum<vi>)
            n238 = control-ref of="Imin vs time"() -> (w960:refnum<vi>)
            n239 = control-ref of="Ion vs time"() -> (w929:refnum<vi>)
            n240 = control-ref of="Ioff vs time"() -> (w928:refnum<vi>)
            n241 = control-ref of="I vs Vg"() -> (w970:refnum<vi>)
            n242 = call "4155C Split array.vi"("Number of VAR2 steps"=w926, "Y2 data in"=w918, "X data in"=w932, "Y1 data in"=w920, "Y3 data in"=w916, "error in (no error)"=w914) -> ("Array of clusters"=w930:cluster{"Y data in":dbl[], "X data in":dbl[]}[], "error out"=w913:errorcluster)  [unwired: 1 in]
            n243 = call "4155C Split array.vi"("Number of VAR2 steps"=w926, "Y2 data in"=w917, "X data in"=w932, "Y1 data in"=w919, "Y3 data in"=w915, "error in (no error)"=w913) -> ("Array of clusters"=w931:cluster{"Y data in":dbl[], "X data in":dbl[]}[], "error out"=w912:errorcluster)  [unwired: 1 in]
            n244 = call "4155C Split array.vi"("Number of VAR2 steps"=w926, "Y2 data in"=w924, "X data in"=w932, "Y1 data in"=w927, "Y3 data in"=w922, "error in (no error)"=w912) -> ("Array of clusters"=w969:cluster{"Y data in":dbl[], "X data in":dbl[]}[], "error out"=w911:errorcluster)  [unwired: 1 in]
            n245 = call "4155C Split array.vi"("Number of VAR2 steps"=w926, "Y2 data in"=w923, "X data in"=w932, "Y1 data in"=w925, "Y3 data in"=w921, "error in (no error)"=w911) -> ("Array of clusters"=w968:cluster{"Y data in":dbl[], "X data in":dbl[]}[], "error out"=w910:errorcluster)  [unwired: 1 in]
            n246 = call "4155C Config Chart Colours.vi"("Numeric"=w926, "XY Graph 2"=w961) -> ()  [unwired: 6 in]
            n247 = call "4155C Config Chart Colours.vi"("Numeric"=w926, "XY Graph 2"=w960) -> ()  [unwired: 6 in]
            n248 = call "4155C Config Chart Colours.vi"("Numeric"=w926, "XY Graph 2"=w929) -> ()  [unwired: 6 in]
            n249 = call "4155C Config Chart Colours.vi"("Numeric"=w926, "XY Graph 2"=w928) -> ()  [unwired: 6 in]
            n250 = call "4155C Config Chart Colours.vi"("Numeric"=w926, "XY Graph 2"=w970) -> ()  [unwired: 6 in]
            n251 = local write "Imax vs time"(w969) -> ()
            n252 = local write "Imin vs time"(w968) -> ()
            n253 = local write "Ion vs time"(w930) -> ()
            n254 = local write "Ioff vs time"(w931) -> ()
          }
        }
        n255 = local write "I vs Vd"(w833) -> ()
        n256 = Open/Create/Replace File(file path (use dialog)=w885, error in=w788, operation (0:open)=w841) -> (refnum out=w828:refnum<file>, error out=w826:errorcluster)  [unwired: 3 in, 1 out]
        n257 = call "4155C Make Big 2d array.vi"("1D Var1"=w840, "1d IS"=w813, "1d ID"=w814, "1d IG"=w812, "1d SMU4"=w843, "SMU4"=w783, "VAR2 START"=w844, "Number of VAR2 steps"=w801, "VAR2 STEP"=w845, "VAR1 Name"="Vd", "Decimal places in header"=i8 1, "VAR2 Name"="Vg") -> ("Header array"=w829:string[], "Data array"=w827:dbl[][])  [unwired: 14 in]
        n258 = call "4155C Write array to file.vi"("Byte Stream File Refnum"=w828, "Header"=w829, "Data Array"=w827, "error in (no error)"=w826) -> ("dup refnum"=w825:refnum<file>, "error out"=w824:errorcluster)  [unwired: 1 in]
        n259 = Close File(refnum=w825, error in=w824) -> (error out=w880:errorcluster)  [unwired: 1 out]
      }
      frame "output-fpp" {
        n260 = Number To Decimal String(number=w996) -> (decimal integer string=w1050:string)  [unwired: 1 in]
        n261 = Bundle By Name(cluster=w1026, "Emergency Stop"=w1053) -> (w1063:T1)
        n262 = Delete From Array(array=w1041, index=0 ("Index")) -> (deleted portion=w1039:string, array with subset deleted=w1038:string[])  [unwired: 1 in]
        n263 = VISA Write(VISA resource name=w1017, write buffer=":PAGE:CHAN:MODE SWE;" ("write buffer (\"\")"), error in (no error)=w1014) -> (VISA resource name out=w1016:refnum<visa-resource-name>, error out=w1015:errorcluster)  [unwired: 1 out]
        n264 = Concatenate Strings(w1049, "-outputfpp-" ("Substring"), w1050, w995, ".txt" ("Substring")) -> (w1052:string)
        n265 = case shown="\"d\", Default" w1039 {
          tunnel: [w1064 w1065] -> w1037
          frame "s" {
            w1064 = u16 0 items=["Single", "Double"] ("sweep mode")
          }
          frame "d", Default {
            w1065 = u16 1 items=["Single", "Double"] ("sweep mode")
          }
        }
        n266 = Fract/Exp String To Number(string=w1038) -> (number=w1020:dbl[])  [unwired: 3 in, 1 out]
        n267 = String To Path(string=w1052) -> (path=w1048:path)
        n268 = Index Array(array=w1020, index #1=0 ("Index")) -> (element #1=w1036:dbl, element #2=w1035:dbl, element #3=w1034:dbl)  [unwired: 2 in]
        n269 = Delete From Array(array=w1020, length=3 ("Length"), index=0 ("Index")) -> (array with subset deleted=w1019:dbl[])  [unwired: 1 out]
        n270 = Bundle By Name(cluster=w1028, "Gate Start"=w1036, "Gate Stop"=w1035, "Gate Step (linear only)"=w1034, "Gate Compliance"=w1046, "Range mode"=w1012, "Range"=w1011) -> (w1062:T6)
        n271 = Index Array(array=w1019, index #1=0 ("Index")) -> (element #1=w1031:dbl, element #2=w1030:dbl, element #3=w1029:dbl)  [unwired: 2 in]
        n272 = call <vilib>:"compatOverwrite.vi"("overwrite (F)"=TRUE) -> ("overwrite?"=w1000:T8)
        n273 = Bundle By Name(cluster=w1027, "Drain Start"=w1031, "Drain Stop"=w1030, "Drain Step"=w1029, "Drain Compliance"=w1047, "Range mode"=w1010, "Range"=w1013) -> (w1061:T7)
        n274 = call "4155C Output-FPP.vi"("VISA resource name in"=w1016, "Gate"=w1062, "Drain"=w1061, "Timings"=w1045, "error in (no error)"=w1015, "sweep mode"=w1037, "Panel controls"=w1063) -> ("VD"=w1005:dbl[], "Outparams"=w1008:T9, "VISA Resource Name out"=w1043:refnum<visa-resource-name>, "Vprobe2"=w1004:dbl[], "ID"=w1003:dbl[], "IG"=w1002:dbl[], "Vprobe1"=w1001:dbl[], "error out"=w1044:errorcluster)  [unwired: 13 in]
        n275 = Unbundle By Name(w1008) -> ("V2 Step"=w1009:dbl, "V2 Start"=w1007:dbl, "Number of points"=w1006:i32)
        n276 = Open/Create/Replace File(file path (use dialog)=w1048, error in=w1044, operation (0:open)=w1000) -> (refnum out=w1058:refnum<file>, error out=w1059:errorcluster)  [unwired: 3 in, 1 out]
        n277 = call "4155C Make Big 2d array FPP.vi"("1D Var1"=w1005, "1d ID"=w1003, "1d Vp2"=w1004, "1d IG"=w1002, "1d Vp1"=w1001, "VAR2 START"=w1007, "Number of VAR2 steps"=w1006, "VAR2 STEP"=w1009, "VAR1 Name"="Vd", "Decimal places in header"=i8 1, "VAR2 Name"="Vg") -> ("Header array"=w1054:string[], "Data array"=w1055:dbl[][])  [unwired: 15 in]
        n278 = call "4155C Write array to file.vi"("Byte Stream File Refnum"=w1058, "Header"=w1054, "Data Array"=w1055, "error in (no error)"=w1059) -> ("dup refnum"=w1056:refnum<file>, "error out"=w1057:errorcluster)  [unwired: 1 in]
        n279 = Close File(refnum=w1056, error in=w1057) -> (error out=w1042:errorcluster)  [unwired: 1 out]
      }
      frame "itime" {
        n280 = Delete From Array(array=w1069, index=1) -> (deleted portion=w1068:string)  [unwired: 1 in, 1 out]
        n281 = Delete From Array(array=w1069, index=0 ("Index")) -> (deleted portion=w1103:string)  [unwired: 1 in, 1 out]
        n282 = Fract/Exp String To Number(string=w1068) -> (number=w1067:dbl)  [unwired: 3 in, 1 out]
        n283 = case shown="\"l\"" w1103 {
          tunnel: w1102 -> [w1108 w1110 w1114]
          tunnel: [w1107 w1109 w1113] -> w1095
          tunnel: w1067 -> [w1105 _ w1112]
          frame "s" {
            w1106 = u32 0 items=["short  ", "medium  ", "long  "] ("integration time 2")
            n284 = Bundle By Name(cluster=w1108, "integration time"=w1106, "Short/Long integration time"=w1105) -> (w1107:T5)
          }
          frame "m", Default {
            w1111 = u32 1 items=["short  ", "medium  ", "long  "] ("integration time 2")
            n285 = Bundle By Name(cluster=w1110, "integration time"=w1111) -> (w1109:T5)
          }
          frame "l" {
            w1115 = u32 2 items=["short  ", "medium  ", "long  "] ("integration time 2")
            n286 = Bundle By Name(cluster=w1114, "integration time"=w1115, "Short/Long integration time"=w1112) -> (w1113:T5)
          }
        }
      }
      frame "pulsed" {
        n287 = Delete From Array(array=w1150, index=0 ("Index")) -> (deleted portion=w1151:string, array with subset deleted=w1138:string[])  [unwired: 1 in]
        n288 = case shown="\"on\", Default" w1151 {
          tunnel: w1149 -> [w1161 w1164]
          tunnel: [w1160 w1163] -> w1142
          tunnel: w1138 -> [w1158 _]
          frame "on", Default {
            w1159 = u16 1 items=["Continuous", "Pulsed"] ("sweep method")
            n289 = Fract/Exp String To Number(string=w1158) -> (number=w1156:dbl[])  [unwired: 3 in, 1 out]
            n290 = Index Array(array=w1156, index #1=0 ("Index")) -> (element #1=w1155:dbl, element #2=w1154:dbl, element #3=w1153:dbl)  [unwired: 2 in]
            n291 = Bundle By Name(cluster=w1161, "sweep method"=w1159, "Pulse period"=w1155, "Base voltage"=w1154, "Pulse width"=w1153) -> (w1160:T5)
          }
          frame "off" {
            w1162 = u16 0 items=["Continuous", "Pulsed"] ("sweep method")
            n292 = Bundle By Name(cluster=w1164, "sweep method"=w1162) -> (w1163:T5)
          }
        }
      }
      frame "gaterangemode" {
        n293 = Delete From Array(array=w1197, index=0 ("Index")) -> (deleted portion=w1198:string)  [unwired: 1 in, 1 out]
        n294 = case shown="\"f\"" w1198 {
          tunnel: [w1200 w1201 w1202] -> w1187
          frame "a", Default {
            w1200 = u16 0 items=["Auto", "Limited", "Fixed"] ("Gate Range\nmode 2")
          }
          frame "f" {
            w1201 = u16 2 items=["Auto", "Limited", "Fixed"] ("Gate Range\nmode 2")
          }
          frame "l" {
            w1202 = u16 1 items=["Auto", "Limited", "Fixed"] ("Gate Range\nmode 2")
          }
        }
      }
      frame "gaterange" {
        (unwired) u8 11 items=["10fA  ", "100fA  ", "1nA  ", "10nA", "100nA", "1uA", "10uA", "100uA", "1mA", "10mA", "100mA", "1A"] ("Gate Range 2")
        n295 = Delete From Array(array=w1242, index=0 ("Index")) -> (deleted portion=w1232:string)  [unwired: 1 in, 1 out]
        n296 = Scan Value(string=w1232, format string="") -> (value=w1230:dbl)  [unwired: 1 in, 1 out]
        n297 = Logarithm Base 10(1:w1230) -> (0:w1229:dbl)
        n298 = Round To Nearest(number=w1229) -> (nearest integer value=w1228:dbl)
        n299 = Add(x=w1228, y=11.0) -> (x+y=w1226:dbl)
        n300 = To Unsigned Byte Integer(number=w1226) -> (unsigned 8bit integer=w1225:u8)
      }
      frame "drainrange" {
        (unwired) u8 11 items=["10fA  ", "100fA  ", "1nA  ", "10nA", "100nA", "1uA", "10uA", "100uA", "1mA", "10mA", "100mA", "1A"] ("Gate Range 2")
        n301 = Delete From Array(array=w1283, index=0 ("Index")) -> (deleted portion=w1274:string)  [unwired: 1 in, 1 out]
        n302 = Scan Value(string=w1274, format string="") -> (value=w1272:dbl)  [unwired: 1 in, 1 out]
        n303 = Logarithm Base 10(1:w1272) -> (0:w1271:dbl)
        n304 = Round To Nearest(number=w1271) -> (nearest integer value=w1270:dbl)
        n305 = Add(x=w1270, y=11.0) -> (x+y=w1268:dbl)
        n306 = To Unsigned Byte Integer(number=w1268) -> (unsigned 8bit integer=w1267:u8)
      }
      frame "drainrangemode" {
        n307 = Delete From Array(array=w1317, index=0 ("Index")) -> (deleted portion=w1318:string)  [unwired: 1 in, 1 out]
        n308 = case shown="\"f\"" w1318 {
          tunnel: [w1320 w1321 w1322] -> w1307
          frame "a", Default {
            w1320 = u16 0 items=["Auto", "Limited", "Fixed"] ("Gate Range\nmode 2")
          }
          frame "f" {
            w1321 = u16 2 items=["Auto", "Limited", "Fixed"] ("Gate Range\nmode 2")
          }
          frame "l" {
            w1322 = u16 1 items=["Auto", "Limited", "Fixed"] ("Gate Range\nmode 2")
          }
        }
      }
      frame "Error", Default {
      }
      frame "logfile" {
        n309 = Number To Decimal String(number=w1377) -> (decimal integer string=w1412:string)  [unwired: 1 in]
        n310 = Concatenate Strings(w1411, "logfile" ("Substring"), w1412, w1375, ".txt" ("Substring")) -> (w1409:string)
        n311 = String To Path(string=w1409) -> (path=w1382:path)
        n312 = Unbundle(w1408) -> ("integration time"=w1407:u32, "Short/Long integration time"=w1406:dbl, "hold time (sec)"=w1405:dbl, "delay time (sec)"=w1404:dbl, "Step Time (0 disables)"=w1403:dbl, "sweep method"=w1402:u16, "Pulse period"=w1401:dbl, "Base voltage"=w1400:dbl, "Pulse width"=w1399:dbl)
        n313 = Build Array(w1407, w1406, w1405, w1404, w1403, w1402, w1401, w1400, w1399, w1393, w1394, w1395, w1396, w1397, w1398) -> (w1386:dbl[])
        n314 = Insert Into Array(array=dbl[][] [] ("Input Array"), new element=w1386) -> (w1385:dbl[][])  [unwired: 2 in]
        n315 = call <vilib>:"compatOverwrite.vi"("overwrite (F)"=TRUE) -> ("overwrite?"=w1380:T8)
        n316 = Open/Create/Replace File(file path (use dialog)=w1382, error in=w1384, operation (0:open)=w1380) -> (refnum out=w1390:refnum<file>, error out=w1389:errorcluster)  [unwired: 3 in, 1 out]
        n317 = call "4155C Write array to file.vi"("Byte Stream File Refnum"=w1390, "Header"=string[] ["Int Time", "Short/Long Itime", "Hold time", "Delay time", "Step time", "Sweep method", "Pulse period", "Base Voltage", "Pulse width", "Drain compliance", "Gate compliance", "Gate range mode", "Gate range", "S/D range mode", "S/D range"], "Data Array"=w1385, "error in (no error)"=w1389) -> ("dup refnum"=w1392:refnum<file>, "error out"=w1391:errorcluster)  [unwired: 1 in]
        n318 = Close File(refnum=w1392, error in=w1391) -> (error out=w1383:errorcluster)  [unwired: 1 out]
      }
      frame "sample" {
        w1436 = 1
        # "The suffix is Vg_Vd_Time."
        # "Add a time offset (elapsed time) to the time axis."
        # "Adjusts graph colors."
        n319 = Number To Decimal String(number=w1470) -> (decimal integer string=w1508:string)  [unwired: 1 in]
        n320 = Fract/Exp String To Number(string=w1506) -> (number=w1474:dbl[])  [unwired: 3 in, 1 out]
        n321 = Index Array(array=w1474, index=0 ("Index")) -> (element=w1420:dbl)
        n322 = Index Array(array=w1474, index=2 ("Index")) -> (element=w1502:dbl)
        n323 = Index Array(array=w1474, index=3 ("Index")) -> (element=w1417:dbl)
        n324 = Index Array(array=w1474, index=4 ("Index")) -> (element=w1473:dbl)
        n325 = call "4155C Config Sampling Measurements.vi"("Sampling interval"=w1473, "Sample time"=w1417, "Display on/off"=TRUE, "Timings"=w1481, "Num Points"=w1502, "error in (no error)"=w1510, "Drain Compliance"=w1509, "Gate Compliance"=w1489, "VISA session"=w1511) -> ("error out"=w1512:errorcluster, "dup VISA resource name"=w1513:refnum<visa-resource-name>)  [unwired: 1 in]
        n326 = Index Array(array=w1474, index=1 ("Index")) -> (element=w1422:dbl)
        n327 = local read "Plot sample extrema vs time"() -> (w1438:bool)
        n328 = Number To Decimal String(number=w1422) -> (decimal integer string=w1423:string)  [unwired: 1 in]
        n329 = Number To Decimal String(number=w1420) -> (decimal integer string=w1419:string)  [unwired: 1 in]
        n330 = Number To Decimal String(number=w1417) -> (decimal integer string=w1416:string)  [unwired: 1 in]
        n331 = call "4155C Take Sample.vi"("Emergency Stop"=w1486, "error in (no error)"=w1512, "Vd"=w1422, "Vg"=w1420, "VISA resource name in"=w1513) -> ("error out"=w1446:errorcluster, "Id"=w1430:dbl[], "Ig"=w1429:dbl[], "VISA Resource Name out"=w1483:refnum<visa-resource-name>, "Is"=w1431:dbl[], "Time"=w1432:dbl[])  [unwired: 1 in]
        n332 = Add(x=w1432, y=w1424) -> (x+y=w1425:dbl[])
        n333 = Concatenate Strings(w1423, "_" ("Substring"), w1419, "_" ("Substring"), w1416, "-sec.txt" ("Substring")) -> (w1414:string)
        n334 = Concatenate Strings(w1427, w1426, w1508, w1468, "_S_" ("Substring"), w1414) -> (w1507:string)
        n335 = String To Path(string=w1507) -> (path=w1492:path)
        n336 = case shown="True" w1438 {
          tunnel: w1425 -> [_ w1516]
          tunnel: [w1514 w1517] -> w1433
          tunnel: w1439 -> [w1514 w1515]
          frame False {
          }
          frame True {
            n337 = Insert Into Array(array=w1515, new element=w1516) -> (w1517:i32[])  [unwired: 1 in]
          }
        }
        n338 = case shown="True" "Plot sample extrema vs time" {
          tunnel: w1431 -> [_ w1546]
          tunnel: w1430 -> [_ w1547]
          tunnel: w1429 -> [_ w1548]
          tunnel: [w1524 w1534] -> w1435
          tunnel: w1446 -> [w1524 w1539]
          tunnel: w1452 -> [w1523 w1551]
          tunnel: w1451 -> [w1522 w1550]
          tunnel: w1450 -> [w1521 w1552]
          tunnel: w1449 -> [w1520 w1549]
          tunnel: w1448 -> [w1519 w1554]
          tunnel: w1447 -> [w1518 w1553]
          tunnel: [w1523 w1538] -> w1445
          tunnel: [w1522 w1532] -> w1444
          tunnel: [w1521 w1536] -> w1443
          tunnel: [w1520 w1531] -> w1442
          tunnel: [w1519 w1537] -> w1441
          tunnel: [w1518 w1530] -> w1440
          tunnel: w1433 -> [_ w1528]
          frame False {
          }
          frame True {
            w1533 = 1
            # "Number of VAR2 steps is 1."
            # "abs(Ig)"
            # "abs(Is)"
            # "abs(Id)"
            # "Adjusts graph colors."
            n339 = Absolute Value(x=w1548) -> (abs(x)=w1525:dbl[])
            n340 = Absolute Value(x=w1547) -> (abs(x)=w1526:dbl[])
            n341 = Absolute Value(x=w1546) -> (abs(x)=w1527:dbl[])
            n342 = Array Max & Min(array=w1527) -> (max value=w1545:dbl, min value=w1542:dbl)  [unwired: 2 out]
            n343 = Array Max & Min(array=w1526) -> (max value=w1544:dbl, min value=w1541:dbl)  [unwired: 2 out]
            n344 = Array Max & Min(array=w1525) -> (max value=w1543:dbl, min value=w1540:dbl)  [unwired: 2 out]
            n345 = local write "Id max"(w1544) -> ()
            n346 = local write "Id min"(w1541) -> ()
            n347 = local write "Ig max"(w1543) -> ()
            n348 = local write "Ig min"(w1540) -> ()
            n349 = Insert Into Array(array=w1554, new element=w1525) -> (w1537:dbl[])  [unwired: 1 in]
            n350 = Insert Into Array(array=w1553, new element=w1525) -> (w1530:dbl[])  [unwired: 1 in]
            n351 = local write "Is max"(w1545) -> ()
            n352 = local write "Is min"(w1542) -> ()
            n353 = Insert Into Array(array=w1552, new element=w1526) -> (w1536:dbl[])  [unwired: 1 in]
            n354 = Insert Into Array(array=w1549, new element=w1526) -> (w1531:dbl[])  [unwired: 1 in]
            n355 = Insert Into Array(array=w1551, new element=w1527) -> (w1538:dbl[])  [unwired: 1 in]
            n356 = Insert Into Array(array=w1550, new element=w1527) -> (w1532:dbl[])  [unwired: 1 in]
            n357 = control-ref of="Imax vs time"() -> (w1555:refnum<vi>)
            n358 = call "4155C Config Chart Colours.vi"("Numeric"=w1533, "XY Graph 2"=w1555) -> ()  [unwired: 6 in]
            n359 = call "4155C Split array.vi"("Number of VAR2 steps"=w1533, "Y2 data in"=w1536, "X data in"=w1528, "Y1 data in"=w1538, "Y3 data in"=w1537, "error in (no error)"=w1539) -> ("Array of clusters"=w1556:cluster{"Y data in":dbl[], "X data in":dbl[]}[], "error out"=w1535:errorcluster)  [unwired: 1 in]
            n360 = call "4155C Split array.vi"("Number of VAR2 steps"=w1533, "Y2 data in"=w1531, "X data in"=w1528, "Y1 data in"=w1532, "Y3 data in"=w1530, "error in (no error)"=w1535) -> ("Array of clusters"=w1529:cluster{"Y data in":dbl[], "X data in":dbl[]}[], "error out"=w1534:errorcluster)  [unwired: 1 in]
            n361 = local write "Imax vs time"(w1556) -> ()
            n362 = local write "Imin vs time"(w1529) -> ()
          }
        }
        n363 = Insert Into Array(array=dbl[][] [] ("Input Array"), new element=w1425) -> (w1496:dbl[][])  [unwired: 2 in]
        n364 = Insert Into Array(array=w1496, new element=w1429) -> (w1495:dbl[][])  [unwired: 2 in]
        n365 = call "4155C Split array.vi"("Number of VAR2 steps"=w1436, "Y2 data in"=w1430, "X data in"=w1425, "Y1 data in"=w1431, "Y3 data in"=w1429, "error in (no error)"=w1435) -> ("Array of clusters"=w1437:cluster{"Y data in":dbl[], "X data in":dbl[]}[], "error out"=w1434:errorcluster)  [unwired: 1 in]
        n366 = VISA Write(VISA resource name=w1483, write buffer=":DISP ON" ("write buffer (\"\")"), error in (no error)=w1434) -> (VISA resource name out=w1482:refnum<visa-resource-name>, error out=w1484:errorcluster)  [unwired: 1 out]
        n367 = Insert Into Array(array=w1495, new element=w1430) -> (w1494:dbl[][])  [unwired: 2 in]
        n368 = Insert Into Array(array=w1494, new element=w1431) -> (w1488:dbl[][])  [unwired: 2 in]
        n369 = local write "I vs time (Bias Stress)"(w1437) -> ()
        n370 = control-ref of="I vs time (Bias Stress)"() -> (w1428:refnum<vi>)
        n371 = call <vilib>:"compatOverwrite.vi"("overwrite (F)"=TRUE) -> ("overwrite?"=w1471:T8)
        n372 = Open/Create/Replace File(file path (use dialog)=w1492, error in=w1484, operation (0:open)=w1471) -> (refnum out=w1499:refnum<file>, error out=w1498:errorcluster)  [unwired: 3 in, 1 out]
        n373 = Transpose 2D Array(2D array=w1488) -> (transposed array=w1487:dbl[][])
        n374 = call "4155C Write array to file.vi"("Byte Stream File Refnum"=w1499, "Header"=string[] ["Time /s", "Ig /A", "Id /A", "Is /A"], "Data Array"=w1487, "error in (no error)"=w1498) -> ("dup refnum"=w1501:refnum<file>, "error out"=w1500:errorcluster)  [unwired: 1 in]
        n375 = call "4155C Config Chart Colours.vi"("Numeric"=w1436, "XY Graph 2"=w1428) -> ()  [unwired: 6 in]
        n376 = Close File(refnum=w1501, error in=w1500) -> (error out=w1490:errorcluster)  [unwired: 1 out]
      }
      frame "samplei" {
        n377 = Number To Decimal String(number=w1579) -> (decimal integer string=w1630:string)  [unwired: 1 in]
        n378 = Concatenate Strings(w1609, "-samplei-" ("Substring"), w1630, w1578, ".txt" ("Substring")) -> (w1628:string)
        n379 = Fract/Exp String To Number(string=w1627) -> (number=w1594:dbl[])  [unwired: 3 in, 1 out]
        n380 = String To Path(string=w1628) -> (path=w1612:path)
        n381 = Index Array(array=w1594, index=4 ("Index")) -> (element=w1588:dbl)
        n382 = Index Array(array=w1594, index=3 ("Index")) -> (element=w1589:dbl)
        n383 = Index Array(array=w1594, index=1 ("Index")) -> (element=w1591:dbl)
        n384 = Index Array(array=w1594, index=0 ("Index")) -> (element=w1592:dbl)
        n385 = Index Array(array=w1594, index=2 ("Index")) -> (element=w1590:dbl)
        n386 = call "4155C Config SamplingI Measurements.vi"("Sample time"=w1590, "Display on/off"=TRUE, "Timings"=w1601, "Num Points"=w1591, "error in (no error)"=w1632, "Sampling interval"=w1589, "VISA session"=w1633) -> ("error out"=w1634:errorcluster, "dup VISA resource name"=w1635:refnum<visa-resource-name>)  [unwired: 3 in]
        n387 = call "4155C Take SampleI.vi"("Emergency Stop"=w1606, "error in (no error)"=w1634, "Idg 2"=w1592, "Vdg compliance 2"=w1588, "VISA resource name in"=w1635) -> ("error out"=w1604:errorcluster, "Idg"=w1637:dbl[], "Vdg"=w1614:dbl[], "VISA Resource Name out"=w1602:refnum<visa-resource-name>, "Is"=w1636:dbl[], "Time"=w1618:dbl[])  [unwired: 1 in]
        n388 = Insert Into Array(array=dbl[][] [] ("Input Array"), new element=w1618) -> (w1617:dbl[][])  [unwired: 2 in]
        n389 = Insert Into Array(array=w1617, new element=w1614) -> (w1616:dbl[][])  [unwired: 2 in]
        n390 = Insert Into Array(array=w1616, new element=w1637) -> (w1615:dbl[][])  [unwired: 2 in]
        n391 = VISA Write(VISA resource name=w1602, write buffer=":DISP ON" ("write buffer (\"\")"), error in (no error)=w1604) -> (VISA resource name out=w1587:refnum<visa-resource-name>, error out=w1603:errorcluster)  [unwired: 1 out]
        n392 = Insert Into Array(array=w1615, new element=w1636) -> (w1608:dbl[][])  [unwired: 2 in]
        n393 = call <vilib>:"compatOverwrite.vi"("overwrite (F)"=TRUE) -> ("overwrite?"=w1582:T8)
        n394 = Open/Create/Replace File(file path (use dialog)=w1612, error in=w1603, operation (0:open)=w1582) -> (refnum out=w1621:refnum<file>, error out=w1620:errorcluster)  [unwired: 3 in, 1 out]
        n395 = Transpose 2D Array(2D array=w1608) -> (transposed array=w1607:dbl[][])
        n396 = call "4155C Write array to file.vi"("Byte Stream File Refnum"=w1621, "Header"=string[] ["Time /s", "Vdg /V", "Idg /A", "Is /A"], "Data Array"=w1607, "error in (no error)"=w1620) -> ("dup refnum"=w1623:refnum<file>, "error out"=w1622:errorcluster)  [unwired: 1 in]
        n397 = Close File(refnum=w1623, error in=w1622) -> (error out=w1585:errorcluster)  [unwired: 1 out]
        n398 = VISA Write(VISA resource name=w1587, write buffer=";:PAGE:SCON:STAN OFF;:PAGE:CHAN:VSU2:DIS;" ("write buffer (\"\")"), error in (no error)=w1585) -> (VISA resource name out=w1583:refnum<visa-resource-name>, error out=w1584:errorcluster)  [unwired: 1 out]
      }
      frame "#" {
        n399 = VISA Write(VISA resource name=w1664, write buffer=":DISP ON" ("write buffer (\"\")"), error in (no error)=w1663) -> (VISA resource name out=w1662:refnum<visa-resource-name>, error out=w1661:errorcluster)  [unwired: 1 out]
      }
      frame "stressV" {
        n400 = Number To Decimal String(number=w1694) -> (decimal integer string=w1735:string)  [unwired: 1 in]
        n401 = Concatenate Strings(w1719, "-stressV-" ("Substring"), w1735, w1693, ".txt" ("Substring")) -> (w1733:string)
        n402 = Fract/Exp String To Number(string=w1732) -> (number=w1705:dbl[])  [unwired: 3 in, 1 out]
        n403 = String To Path(string=w1733) -> (path=w1723:path)
        n404 = Index Array(array=w1705, index=3 ("Index")) -> (element=w1702:dbl)
        n405 = Index Array(array=w1705, index=1 ("Index")) -> (element=w1700:dbl)
        n406 = Index Array(array=w1705, index=0 ("Index")) -> (element=w1699:dbl)
        n407 = Index Array(array=w1705, index=4 ("Index")) -> (element=w1704:dbl)
        n408 = Index Array(array=w1705, index=2 ("Index")) -> (element=w1701:dbl)
        n409 = call "4155C Config V Stress.vi"("VISA session"=w1738, "ID compliance"=w1702, "VD"=w1700, "VG"=w1699, "IG compliance"=w1701, "error in (no error)"=w1737, "Display on/off"=TRUE) -> ("dup VISA resource name"=w1740:refnum<visa-resource-name>, "error out"=w1739:errorcluster)
        n410 = call "4155C Apply Stress.vi"("error in (no error)"=w1739, "Duration"=w1704, "Emergency Stop"=w1718, "VISA resource name in"=w1740) -> ("error out"=w1716:errorcluster, "VISA Resource Name out"=w1714:refnum<visa-resource-name>)
        n411 = VISA Write(VISA resource name=w1714, write buffer=":DISP ON" ("write buffer (\"\")"), error in (no error)=w1716) -> (VISA resource name out=w1713:refnum<visa-resource-name>, error out=w1715:errorcluster)  [unwired: 1 out]
        n412 = call <vilib>:"compatOverwrite.vi"("overwrite (F)"=TRUE) -> ("overwrite?"=w1698:T8)
        n413 = Open/Create/Replace File(file path (use dialog)=w1723, error in=w1715, operation (0:open)=w1698) -> (refnum out=w1726:refnum<file>, error out=w1725:errorcluster)  [unwired: 3 in, 1 out]
        n414 = call "4155C Write array to file.vi"("Byte Stream File Refnum"=w1726, "Header"=string[] ["V stress completed successfully", ""], "error in (no error)"=w1725) -> ("dup refnum"=w1728:refnum<file>, "error out"=w1727:errorcluster)  [unwired: 2 in]
        n415 = Close File(refnum=w1728, error in=w1727) -> (error out=w1721:errorcluster)  [unwired: 1 out]
      }
      frame "stressI" {
        n416 = Number To Decimal String(number=w1762) -> (decimal integer string=w1799:string)  [unwired: 1 in]
        n417 = Concatenate Strings(w1783, "-stressI-" ("Substring"), w1799, w1761, ".txt" ("Substring")) -> (w1797:string)
        n418 = Fract/Exp String To Number(string=w1796) -> (number=w1771:dbl[])  [unwired: 3 in, 1 out]
        n419 = Index Array(array=w1771, index=1 ("Index")) -> (element=w1767:dbl)
        n420 = Index Array(array=w1771, index=0 ("Index")) -> (element=w1768:dbl)
        n421 = call "4155C Config I Stress.vi"("VISA session"=w1802, "IDG"=w1768, "VDG compliance"=w1767, "error in (no error)"=w1801, "Display on/off"=TRUE) -> ("dup VISA resource name"=w1804:refnum<visa-resource-name>, "error out"=w1803:errorcluster)
        n422 = Index Array(array=w1771, index=2 ("Index")) -> (element=w1769:dbl)
        n423 = String To Path(string=w1797) -> (path=w1787:path)
        n424 = call "4155C Apply Stress.vi"("error in (no error)"=w1803, "Duration"=w1769, "Emergency Stop"=w1782, "VISA resource name in"=w1804) -> ("error out"=w1780:errorcluster, "VISA Resource Name out"=w1778:refnum<visa-resource-name>)
        n425 = VISA Write(VISA resource name=w1778, write buffer=":DISP ON" ("write buffer (\"\")"), error in (no error)=w1780) -> (VISA resource name out=w1777:refnum<visa-resource-name>, error out=w1779:errorcluster)  [unwired: 1 out]
        n426 = call <vilib>:"compatOverwrite.vi"("overwrite (F)"=TRUE) -> ("overwrite?"=w1766:T8)
        n427 = Open/Create/Replace File(file path (use dialog)=w1787, error in=w1779, operation (0:open)=w1766) -> (refnum out=w1790:refnum<file>, error out=w1789:errorcluster)  [unwired: 3 in, 1 out]
        n428 = call "4155C Write array to file.vi"("Byte Stream File Refnum"=w1790, "Header"=string[] ["I stress completed successfully", ""], "error in (no error)"=w1789) -> ("dup refnum"=w1792:refnum<file>, "error out"=w1791:errorcluster)  [unwired: 2 in]
        n429 = Close File(refnum=w1792, error in=w1791) -> (error out=w1785:errorcluster)  [unwired: 1 out]
      }
      frame "vsu2pulse" {
        n430 = Number To Decimal String(number=w1826) -> (decimal integer string=w1861:string)  [unwired: 1 in]
        n431 = Concatenate Strings(w1846, "-vsu2-" ("Substring"), w1861, w1825, ".txt" ("Substring")) -> (w1859:string)
        n432 = Fract/Exp String To Number(string=w1858) -> (number=w1834:dbl[])  [unwired: 3 in, 1 out]
        n433 = String To Path(string=w1859) -> (path=w1850:path)
        n434 = Index Array(array=w1834, index=1 ("Index")) -> (element=w1833:dbl)
        n435 = Index Array(array=w1834, index=0 ("Index")) -> (element=w1831:dbl)
        n436 = call "4155C Config VSU2 Stress.vi"("error in (no error)"=w1863, "VSU2"=w1831, "Display on/off"=TRUE, "VISA session"=w1864) -> ("error out"=w1865:errorcluster, "dup VISA resource name"=w1866:refnum<visa-resource-name>)
        n437 = call "4155C Apply Stress.vi"("error in (no error)"=w1865, "Duration"=w1833, "Emergency Stop"=w1845, "VISA resource name in"=w1866) -> ("error out"=w1843:errorcluster, "VISA Resource Name out"=w1841:refnum<visa-resource-name>)
        n438 = VISA Write(VISA resource name=w1841, write buffer=":DISP ON" ("write buffer (\"\")"), error in (no error)=w1843) -> (VISA resource name out=w1840:refnum<visa-resource-name>, error out=w1842:errorcluster)  [unwired: 1 out]
        n439 = call <vilib>:"compatOverwrite.vi"("overwrite (F)"=TRUE) -> ("overwrite?"=w1830:T8)
        n440 = Open/Create/Replace File(file path (use dialog)=w1850, error in=w1842, operation (0:open)=w1830) -> (refnum out=w1853:refnum<file>, error out=w1852:errorcluster)  [unwired: 3 in, 1 out]
        n441 = call "4155C Write array to file.vi"("Byte Stream File Refnum"=w1853, "Header"=string[] ["VSU2 pulse completed successfully", ""], "error in (no error)"=w1852) -> ("dup refnum"=w1855:refnum<file>, "error out"=w1854:errorcluster)  [unwired: 2 in]
        n442 = Close File(refnum=w1855, error in=w1854) -> (error out=w1848:errorcluster)  [unwired: 1 out]
      }
      frame "sample-fpp" {
        w1899 = string[] ["Time /s", "Id VgVd /A", "Ig VgVd /A", "Vp1 VgVd /V", "Vp2 VgVd /V"] ("Header")
        w1903 = "%d" ("format string")
        n443 = Number To Decimal String(number=w1888) -> (decimal integer string=w1951:string)  [unwired: 1 in]
        n444 = Fract/Exp String To Number(string=w1948) -> (number=w1936:dbl[])  [unwired: 3 in, 1 out]
        n445 = Concatenate Strings(w1942, "-samplefpp-" ("Substring"), w1951, w1887, ".txt" ("Substring")) -> (w1949:string)
        n446 = String To Path(string=w1949) -> (path=w1911:path)
        n447 = Index Array(array=w1936, index=0 ("Index")) -> (element=w1897:dbl)
        n448 = Index Array(array=w1936, index=1 ("Index")) -> (element=w1896:dbl)
        n449 = Index Array(array=w1936, index=2 ("Index")) -> (element=w1944:dbl)
        n450 = Index Array(array=w1936, index=3 ("Index")) -> (element=w1934:dbl)
        n451 = call "4155C Config Sampling Measurements FPP.vi"("VISA session"=w1954, "Num Points"=w1944, "Vg"=w1897, "Display on/off"=TRUE, "Gate Compliance"=w1943, "Drain Compliance"=w1952, "Standby"="Standby", "error in (no error)"=w1953, "Timings"=w1941, "Vd"=w1896, "Sample time"=w1934) -> ("dup VISA resource name"=w1913:refnum<visa-resource-name>, "error out"=w1912:errorcluster)  [unwired: 3 in]
        n452 = Number To Decimal String(number=w1897) -> (decimal integer string=w1923:string)  [unwired: 1 in]
        n453 = call "4155C Take Sample FPP.vi"("VISA resource name in"=w1913, "error in (no error)"=w1912, "Emergency Stop"=w1914) -> ("Time"=w1918:dbl[], "Vp1"=w1928:dbl[], "VISA Resource Name out"=w1894:refnum<visa-resource-name>, "Ig"=w1916:dbl[], "Id"=w1917:dbl[], "Vp2"=w1926:dbl[], "error out"=w1915:errorcluster)  [unwired: 10 in]
        n454 = Insert Into Array(array=dbl[][] [] ("Input Array"), new element=w1918) -> (w1932:dbl[][])  [unwired: 2 in]
        n455 = Number To Decimal String(number=w1896) -> (decimal integer string=w1921:string)  [unwired: 1 in]
        n456 = Insert Into Array(array=w1932, new element=w1917) -> (w1931:dbl[][])  [unwired: 2 in]
        n457 = Concatenate Strings("(Vg = " ("Substring"), w1923, "V, Vd = " ("Substring"), w1921, "V)" ("Substring")) -> (w1919:string)
        n458 = Insert Into Array(array=w1931, new element=w1916) -> (w1930:dbl[][])  [unwired: 2 in]
        n459 = Insert Into Array(array=w1930, new element=w1928) -> (w1927:dbl[][])  [unwired: 2 in]
        n460 = Insert Into Array(array=w1927, new element=w1926) -> (w1895:dbl[][])  [unwired: 2 in]
        n461 = Transpose 2D Array(2D array=w1895) -> (transposed array=w1925:dbl[][])
        n462 = call <vilib>:"compatOverwrite.vi"("overwrite (F)"=TRUE) -> ("overwrite?"=w1892:T8)
        n463 = Open/Create/Replace File(file path (use dialog)=w1911, error in=w1915, operation (0:open)=w1892) -> (refnum out=w1908:refnum<file>, error out=w1909:errorcluster)  [unwired: 3 in, 1 out]
        n464 = Array To Spreadsheet String(array=w1899, 3:w1903) -> (spreadsheet string=w1905:string)  [unwired: 1 in]
        n465 = Search and Replace String(replace all?=TRUE ("replace all? (F)"), input string=w1905, search string="VgVd", replace string=w1919) -> (result string=w1901:string)  [unwired: 4 in, 3 out]
        n466 = Spreadsheet String To Array(format string=w1903, spreadsheet string=w1901, array type (2D Dbl)=w1899) -> (array=w1900:string[])  [unwired: 1 in]
        n467 = call "4155C Write array to file.vi"("Byte Stream File Refnum"=w1908, "Header"=w1900, "Data Array"=w1925, "error in (no error)"=w1909) -> ("dup refnum"=w1906:refnum<file>, "error out"=w1907:errorcluster)  [unwired: 1 in]
        n468 = Close File(refnum=w1906, error in=w1907) -> (error out=w1893:errorcluster)  [unwired: 1 out]
      }
      frame "resample-fpp" {
        w1989 = string[] ["Time /s", "Id VgVd /A", "Ig VgVd /A", "Vp1 VgVd /V", "Vp2 VgVd /V"] ("Header")
        w1993 = "%d" ("format string")
        n469 = Number To Decimal String(number=w1975) -> (decimal integer string=w2033:string)  [unwired: 1 in]
        n470 = Fract/Exp String To Number(string=w2030) -> (number=w1982:dbl[])  [unwired: 3 in, 1 out]
        n471 = Concatenate Strings(w2026, "-resamplefpp-" ("Substring"), w2033, w1976, ".txt" ("Substring")) -> (w2031:string)
        n472 = String To Path(string=w2031) -> (path=w2001:path)
        n473 = Index Array(array=w1982, index=0 ("Index")) -> (element=w1988:dbl)
        n474 = Index Array(array=w1982, index=1 ("Index")) -> (element=w1987:dbl)
        n475 = Number To Decimal String(number=w1988) -> (decimal integer string=w2011:string)  [unwired: 1 in]
        n476 = call "4155C Take Sample FPP.vi"("VISA resource name in"=w1984, "error in (no error)"=w1983, "Emergency Stop"=w2002) -> ("Time"=w2006:dbl[], "Vp1"=w2016:dbl[], "VISA Resource Name out"=w1986:refnum<visa-resource-name>, "Ig"=w2004:dbl[], "Id"=w2005:dbl[], "Vp2"=w2014:dbl[], "error out"=w2003:errorcluster)  [unwired: 10 in]
        n477 = Insert Into Array(array=dbl[][] [] ("Input Array"), new element=w2006) -> (w2020:dbl[][])  [unwired: 2 in]
        n478 = Number To Decimal String(number=w1987) -> (decimal integer string=w2009:string)  [unwired: 1 in]
        n479 = Insert Into Array(array=w2020, new element=w2005) -> (w2019:dbl[][])  [unwired: 2 in]
        n480 = Concatenate Strings("(Vg = " ("Substring"), w2011, "V, Vd = " ("Substring"), w2009, "V)" ("Substring")) -> (w2007:string)
        n481 = Insert Into Array(array=w2019, new element=w2004) -> (w2018:dbl[][])  [unwired: 2 in]
        n482 = Insert Into Array(array=w2018, new element=w2016) -> (w2015:dbl[][])  [unwired: 2 in]
        n483 = Insert Into Array(array=w2015, new element=w2014) -> (w1981:dbl[][])  [unwired: 2 in]
        n484 = call <vilib>:"compatOverwrite.vi"("overwrite (F)"=TRUE) -> ("overwrite?"=w1980:T8)
        n485 = Open/Create/Replace File(file path (use dialog)=w2001, error in=w2003, operation (0:open)=w1980) -> (refnum out=w1998:refnum<file>, error out=w1999:errorcluster)  [unwired: 3 in, 1 out]
        n486 = Array To Spreadsheet String(array=w1989, 3:w1993) -> (spreadsheet string=w1995:string)  [unwired: 1 in]
        n487 = Transpose 2D Array(2D array=w1981) -> (transposed array=w2013:dbl[][])
        n488 = Search and Replace String(replace all?=TRUE ("replace all? (F)"), input string=w1995, search string="VgVd", replace string=w2007) -> (result string=w1991:string)  [unwired: 4 in, 3 out]
        n489 = Spreadsheet String To Array(format string=w1993, spreadsheet string=w1991, array type (2D Dbl)=w1989) -> (array=w1990:string[])  [unwired: 1 in]
        n490 = call "4155C Write array to file.vi"("Byte Stream File Refnum"=w1998, "Header"=w1990, "Data Array"=w2013, "error in (no error)"=w1999) -> ("dup refnum"=w1996:refnum<file>, "error out"=w1997:errorcluster)  [unwired: 1 in]
        n491 = Close File(refnum=w1996, error in=w1997) -> (error out=w1985:errorcluster)  [unwired: 1 out]
      }
      frame "serial" {
        n492 = local read "Termination char\n(0xA = '\\n' = LF)\n(0xD = '\\r' = CR)"() -> (w2062:u8)
        n493 = local read "Enable Termination\nChar (T)"() -> (w2063:bool)
        n494 = Index Array(array=w2070, index=0 ("Index")) -> (element=w2069:string)
        n495 = local read "parity"() -> (w2053:u16)
        n496 = local read "Delay before read (ms)"() -> (w2064:u32)
        n497 = local read "byte count"() -> (w2061:u32)
        n498 = local read "Timeout (ms)"() -> (w2060:u32)
        n499 = local read "VISA resource name"() -> (w2057:refnum<visa-resource-name>)
        n500 = local read "baud rate"() -> (w2056:u32)
        n501 = local read "Serial End Mode for Reads"() -> (w2055:u16)
        n502 = local read "data bits"() -> (w2054:u16)
        n503 = local read "stop bits"() -> (w2059:u16)
        n504 = local read "flow control"() -> (w2058:u16)
        n505 = call "Serial write and read v0.5.vi"("Delay before read (ms)"=w2064, "Termination char\n(0xA = '\\n' = LF)\n(0xD = '\\r' = CR)"=w2062, "Enable Termination\nChar (T)"=w2063, "parity"=w2053, "stop bits"=w2059, "string to write"=w2069, "flow control"=w2058, "byte count"=w2061, "Serial Settings:Serial End Mode for Reads"=w2055, "Timeout (ms)"=w2060, "error in (no error)"=w2075, "VISA resource name"=w2057, "baud rate"=w2056, "data bits"=w2054) -> ("Serial port output"=w2065:string, "error out"=w2074:errorcluster)
        n506 = Build Array (concatenate)(w2065, w2066) -> (w2067:string[])
      }
      frame "pump" {
        # "Time array for valve position"
        # "Time array for absolute plunger position"
        # "Valve position"
        # "Absolute plunger position"
        # "Remove \"_\""
        # "Check if hard stop is pressed."
        # "Check if halt is pressed."
        # "Check if pump is idle. Else halt."
        n507 = Index Array(array=w2141, index=0 ("Index")) -> (element=w2118:string)
        n508 = case shown="\"No error\", Default" w2116 {
          tunnel: w2118 -> [w2177 _ w2179 w2180 w2181 w2182 _ _ w2185 w2186 _]
          tunnel: [w2177 "/1H" w2179 w2180 w2181 w2182 "/1H" "/1H" w2185 w2186 "/1H"] -> w2117
          frame "No error", Default {
          }
          frame "Initialization" {
          }
          frame "Invalid command" {
          }
          frame "Invalid operand" {
          }
          frame "Device not initialized" {
          }
          frame "Internal failure" {
          }
          frame "Plunger overload" {
          }
          frame "Valve overload" {
          }
          frame "Plunger move not allowed" {
          }
          frame "A/D converter failure" {
          }
          frame "Command overflow" {
          }
        }
        n509 = local read "Hard stop pump"() -> (w2120:bool)
        n510 = local read "Halt pump"() -> (w2123:bool)
        n511 = local read "Serial End Mode for Reads"() -> (w2129:u16)
        n512 = local read "flow control"() -> (w2132:u16)
        n513 = local read "stop bits"() -> (w2133:u16)
        n514 = local read "parity"() -> (w2127:u16)
        n515 = local read "Delay before read (ms)"() -> (w2138:u32)
        n516 = local read "byte count"() -> (w2135:u32)
        n517 = local read "Timeout (ms)"() -> (w2134:u32)
        n518 = local read "VISA resource name"() -> (w2131:refnum<visa-resource-name>)
        n519 = local read "baud rate"() -> (w2130:u32)
        n520 = local read "Enable Termination\nChar (T)"() -> (w2137:bool)
        n521 = local read "Termination char\n(0xA = '\\n' = LF)\n(0xD = '\\r' = CR)"() -> (w2136:u8)
        n522 = case shown="True" w2123 {
          tunnel: [w2191 "/1H"] -> w2122
          tunnel: w2117 -> [w2191 _]
          frame False {
          }
          frame True {
            n523 = local write "Halt pump"(FALSE) -> ()
          }
        }
        n524 = case shown="True" w2120 {
          tunnel: [w2188 "/1T"] -> w2121
          tunnel: w2122 -> [w2188 _]
          frame False {
          }
          frame True {
            n525 = local write "Hard stop pump"(FALSE) -> ()
          }
        }
        n526 = local read "data bits"() -> (w2128:u16)
        n527 = String Subset(string=w2112, offset (0)=1) -> (substring=w2110:string)  [unwired: 1 in]
        n528 = call "SPM Pump v0.6.vi"("Termination char\n(0xA = '\\n' = LF)\n(0xD = '\\r' = CR)"=w2136, "Enable Termination\nChar (T)"=w2137, "Timeout (ms)"=w2134, "Serial Settings:Serial End Mode for Reads"=w2129, "byte count"=w2135, "Delay before read (ms)"=w2138, "Time <input>"=w2115, "error in (no error)"=w2146, "Serial port input"=w2121, "VISA resource name"=w2131, "parity"=w2127, "baud rate"=w2130, "stop bits"=w2133, "data bits"=w2128, "flow control"=w2132, "Time units <input>"=w2110) -> ("Input command"=w2109:string, "Serial port data"=w2099:string[], "Pump status"=w2105:string, "Valve position"=w2107:i32, "Absolute plunger position"=w2119:i32, "Serial port"=w2114:string, "error out"=w2145:errorcluster)  [unwired: 1 in, 4 out]
        n529 = case shown="\"?6\"" w2109 {
          tunnel: [w2158 w2166 w2172] -> w2126
          tunnel: w2125 -> [w2158 w2165 w2172]
          tunnel: w2119 -> [_ w2164 _]
          tunnel: w2106 -> [w2157 w2163 w2173]
          tunnel: [w2157 w2163 w2175] -> w2108
          tunnel: w2107 -> [_ _ w2174]
          tunnel: w2104 -> [_ w2162 w2170]
          tunnel: w2103 -> [w2156 w2161 w2171]
          tunnel: [w2156 w2160 w2171] -> w2102
          tunnel: [w2155 w2159 w2169] -> w2101
          tunnel: w2100 -> [w2155 w2159 w2168]
          frame "Q", Default {
          }
          frame "?" {
            n530 = Build Array (concatenate)(w2165, w2164) -> (w2166:i32[])
            n531 = Build Array (concatenate)(w2161, w2162) -> (w2160:i32[])
            n532 = call "4155C Split array.vi"("X data in"=w2160, "Y1 data in"=w2166) -> ("Array of clusters"=w2167:cluster{"Y data in":dbl[], "X data in":dbl[]}[])  [unwired: 5 in, 1 out]
            n533 = local write "Absolute plunger position vs time"(w2167) -> ()
          }
          frame "?6" {
            n534 = Build Array (concatenate)(w2173, w2174) -> (w2175:i32[])
            n535 = Build Array (concatenate)(w2168, w2170) -> (w2169:i32[])
            n536 = call "4155C Split array.vi"("X data in"=w2169, "Y1 data in"=w2175) -> ("Array of clusters"=w2176:cluster{"Y data in":dbl[], "X data in":dbl[]}[])  [unwired: 5 in, 1 out]
            n537 = local write "Valve position vs time"(w2176) -> ()
          }
        }
        n538 = Build Array (concatenate)(w2097, w2099) -> (w2098:string[][])
        n539 = Build Array (concatenate)(w2113, w2114) -> (w2139:string[])
      }
      frame "filename" {
        n540 = Index Array(array=w2196, index=0 ("Index")) -> (element=w2195:string)
      }
    }
    n541 = local read "Time Units"() -> (w73:u16)
    n542 = case shown="2" w73 {
      tunnel: ["Time (Seconds)" ("element") "Time (Minutes)" ("element") "Time (Hours)" ("element")] -> w113
      frame 0 {
      }
      frame 1, Default {
      }
      frame 2 {
      }
    }
    n543 = Build Array(w151, w81, w91, w90, w89, w88, w87, w86, w85, w84, w83, w82, w80) -> (w189:dbl[][])
    n544 = Transpose 2D Array(2D array=w189) -> (transposed array=w188:dbl[][])
    n545 = Concatenate Strings(w132, w75, "Imax_Imin_Ion_Ioff_vs_time.txt" ("Suffix (Imax,Imin,Ion,Ioff)")) -> (w199:string)
    n546 = Build Array(w113, "Is max (A)" ("VAR2 Name"), "Is min (A)" ("VAR2 Name"), "Id max (A)" ("VAR2 Name"), "Id min (A)" ("VAR2 Name"), "Ig max (A)" ("VAR2 Name"), "Ig min (A)" ("VAR2 Name"), "Is on (A)" ("VAR2 Name"), "Is off (A)" ("VAR2 Name"), "Id on (A)" ("VAR2 Name"), "Id off (A)" ("VAR2 Name"), "Ig on (A)" ("VAR2 Name"), "Ig off (A)" ("VAR2 Name")) -> (w194:string[])
    n547 = Array To Spreadsheet String(array=w188, 3:"%e" ("format string")) -> (spreadsheet string=w192:string)  [unwired: 1 in]
    n548 = Array To Spreadsheet String(array=w194, 3:"" ("format string")) -> (spreadsheet string=w193:string)  [unwired: 1 in]
    n549 = String To Path(string=w199) -> (path=w198:path)
    n550 = Build Array(w193, w192) -> (w191:string[])
    n551 = Write to Text File(file (use dialog)=w198, text=w191, error in=w148) -> (refnum out=w200:refnum<file>, error out=w190:errorcluster)  [unwired: 1 in, 1 out]
    n552 = Close File(refnum=w200, error in=w190) -> (error out=w131:errorcluster)  [unwired: 1 out]
    n553 = Build Array(w127, w152) -> (w157:i32[][])
    n554 = Build Array(w113, "Absolute plunger position" ("VAR2 Name")) -> (w160:string[])
    n555 = Transpose 2D Array(2D array=w157) -> (transposed array=w150:i32[][])
    n556 = Array To Spreadsheet String(array=w160, 3:"" ("format string")) -> (spreadsheet string=w159:string)  [unwired: 1 in]
    n557 = Array To Spreadsheet String(array=w150, 3:"%e" ("format string")) -> (spreadsheet string=w156:string)  [unwired: 1 in]
    n558 = Build Array(w159, w156) -> (w162:string[])
    n559 = Concatenate Strings(w132, w75, "plunger_vs_time.txt" ("Suffix (plunger)")) -> (w154:string)
    n560 = String To Path(string=w154) -> (path=w153:path)
    n561 = Write to Text File(file (use dialog)=w153, text=w162, error in=w131) -> (refnum out=w155:refnum<file>, error out=w164:errorcluster)  [unwired: 1 in, 1 out]
    n562 = Close File(refnum=w155, error in=w164) -> (error out=w130:errorcluster)  [unwired: 1 out]
    n563 = Concatenate Strings(w132, w75, "serial_port_output.txt" ("Suffix (serial port log)")) -> (w170:string)
    n564 = String To Path(string=w170) -> (path=w169:path)
    n565 = Build Array(w113, "Serial port input" ("VAR2 Name"), "Pump status" ("VAR2 Name"), "Serial port output: ") -> (w117:string[])
    n566 = Array To Spreadsheet String(array=w123, 3:"" ("format string")) -> (spreadsheet string=w114:string)  [unwired: 1 in]
    n567 = Array To Spreadsheet String(array=w117, 3:"" ("format string")) -> (spreadsheet string=w115:string)  [unwired: 1 in]
    n568 = Array To Spreadsheet String(array=w122, 3:"" ("format string")) -> (spreadsheet string=w175:string)  [unwired: 1 in]
    n569 = Build Array(w115, w114) -> (w116:string[])
    n570 = Write to Text File(file (use dialog)=w169, text=w116, error in=w130) -> (refnum out=w171:refnum<file>, error out=w172:errorcluster)  [unwired: 1 in, 1 out]
    n571 = local write "Serial port data"(w175) -> ()
    n572 = Close File(refnum=w171, error in=w172) -> (error out=w129:errorcluster)  [unwired: 1 out]
    n573 = Build Array(w126, w134) -> (w140:i32[][])
    n574 = Build Array(w113, "Valve port" ("VAR2 Name")) -> (w143:string[])
    n575 = Transpose 2D Array(2D array=w140) -> (transposed array=w135:i32[][])
    n576 = Array To Spreadsheet String(array=w143, 3:"" ("format string")) -> (spreadsheet string=w142:string)  [unwired: 1 in]
    n577 = Array To Spreadsheet String(array=w135, 3:"%e" ("format string")) -> (spreadsheet string=w139:string)  [unwired: 1 in]
    n578 = Build Array(w142, w139) -> (w145:string[])
    n579 = Concatenate Strings(w132, w75, "valve_port_vs_time.txt" ("Suffix (valve)")) -> (w137:string)
    n580 = String To Path(string=w137) -> (path=w136:path)
    n581 = Write to Text File(file (use dialog)=w136, text=w145, error in=w129) -> (refnum out=w138:refnum<file>, error out=w147:errorcluster)  [unwired: 1 in, 1 out]
    n582 = Close File(refnum=w138, error in=w147) -> (error out=w128:errorcluster)  [unwired: 1 out]
  }
  "error out" <- w32
  "Timings Indicator" <- w16
  "SMU4 Indicator" <- w1
  "Is max" <- w14
  "Id max" <- w14
  "Ig max" <- w14
  "Imax vs time" <- w10
  "I vs Vg" <- w10
  "Imin vs time" <- w10
  "I vs Vd" <- w10
  "Serial port data" <- "" ("Serial port data")
  "Valve position vs time" <- cluster{"Y data in":dbl[], "X data in":dbl[]}[] [] ("Valve position vs time")
  "Is min" <- w13
  "Id min" <- w13
  "Ig min" <- w13
  "Ion vs time" <- w10
  "Ioff vs time" <- w10
  "Is on" <- w12
  "Id on" <- w12
  "Ig on" <- w12
  "Is off" <- w11
  "Id off" <- w11
  "Ig off" <- w11
